vi "DATA.vi"(6 "Torsiometro":refnum<vi>, 7 "simulazione":bool, 8 "error in (no error)":errorcluster, 9 "BANCO":i32=1, 10 "variant":variant, 11 "Queue Name":string) -> (0 "error out":errorcluster, 2 "Stopped":bool)   [LabVIEW 2019]
uses:
  TypeDef/MISURE WT.ctl
  TypeDef/Cluster INFO.ctl
  TypeDef/WT SELECTION.ctl
  TypeDef/Definizione linea.ctl
  TypeDef/Collegamenti_elettrici.ctl
  TypeDef/Control Calcoli.ctl
  TypeDef/Cluster MISURE.ctl
  TypeDef/MISURE NM.ctl
  TypeDef/Cluster misure ALL.ctl
  TypeDef/Cluster NI.ctl
  cDAQ_PLC Folder/controls/StatoAO_cdaq.ctl
  cDAQ_PLC Folder/controls/statoDO_Cdaq.ctl
  TypeDef/ClusterRes.ctl
  TypeDef/INTERFACCIA.ctl
  TypeDef/Lista AO sistema.ctl
  TypeDef/DOinterfaccia.ctl
  cDAQ_PLC Folder/ST1200_LIST_IO/STATO PLC 1.ctl
  cDAQ_PLC Folder/ST1200_LIST_IO/Uscite PLC 1.ctl
  cDAQ_PLC Folder/controls/statoAO_plc_1.ctl
  cDAQ_PLC Folder/ST1200_LIST_IO/StatoDO_PLC_1.ctl
  SINUS PENTA SANTERNO/controls/Parametri inverter letti.ctl
  cDAQ_PLC Folder/ST1200_LIST_IO/STATO PLC 2.ctl
  cDAQ_PLC Folder/ST1200_LIST_IO/Uscite PLC 2.ctl
  cDAQ_PLC Folder/controls/statoAO_plc_2.ctl
  cDAQ_PLC Folder/ST1200_LIST_IO/StatoDO_PLC_2.ctl
  cDAQ_PLC Folder/ST1200_LIST_IO/STATO PLC 3.ctl
  cDAQ_PLC Folder/ST1200_LIST_IO/Uscite PLC 3.ctl
  cDAQ_PLC Folder/controls/statoAO_plc_3.ctl
  cDAQ_PLC Folder/ST1200_LIST_IO/StatoDO_PLC_3.ctl
  DCREG/Parametri DCREG letti.ctl
  TypeDef/sett T e R.ctl
  <vilib>/Analysis/baseanly.llb/Mean (DBL).vi
  Globals.vi
  <vilib>/Utility/file.llb/Read Delimited Spreadsheet (string).vi
  Global prova in corso.vi
  <vilib>/Analysis/NI_AALBase.lvlib
panel:
  out "Cluster READ NI":T1 {"AI (4-20mA)"."AI 15" format="%#_6f"; "AI (4-20mA)"."AI 14" format="%#_6f"; "AI (4-20mA)"."AI 13" format="%#_6f"; "AI (4-20mA)"."AI 11" format="%#_6f"; "AI (4-20mA)"."AI 10" format="%#_6f"; "AI (4-20mA)"."AI 9" format="%#_6f"; "AI (4-20mA)"."AI 4" format="%#_6f"; "AI (4-20mA)"."AI 12" format="%#_6f"; "AI (4-20mA)"."AI 0" format="%#_6f"; "AI (4-20mA)"."AI 1" format="%#_6f"; "AI (4-20mA)"."AI 2" format="%#_6f"; "AI (4-20mA)"."AI 3" format="%#_6f"; "AI (4-20mA)"."AI 5" format="%#_6f"; "AI (4-20mA)"."AI 6" format="%#_6f"; "AI (4-20mA)"."AI 7" format="%#_6f"; "AI (4-20mA)"."AI 8" format="%#_6f"; "AI (0-10V)"."AI 31" format="%#_6f"; "AI (0-10V)"."AI 30" format="%#_6f"; "AI (0-10V)"."AI 29" format="%#_6f"; "AI (0-10V)"."AI 28" format="%#_6f"; "AI (0-10V)"."AI 27" format="%#_6f"; "AI (0-10V)"."AI 26" format="%#_6f"; "AI (0-10V)"."AI 25" format="%#_6f"; "AI (0-10V)"."AI 24" format="%#_6f"; "AI (0-10V)"."AI 23" format="%#_6f"; "AI (0-10V)"."AI 22" format="%#_6f"; "AI (0-10V)"."AI 21" format="%#_6f"; "AI (0-10V)"."AI 20" format="%#_6f"; "AI (0-10V)"."AI 19" format="%#_6f"; "AI (0-10V)"."AI 18" format="%#_6f"; "AI (0-10V)"."AI 17" format="%#_6f"; "AI (0-10V)"."AI 16" format="%#_6f"; "AI (0-10V)"."AI 15" format="%#_6f"; "AI (0-10V)"."AI 14" format="%#_6f"; "AI (0-10V)"."AI 13" format="%#_6f"; "AI (0-10V)"."AI 11" format="%#_6f"; "AI (0-10V)"."AI 10" format="%#_6f"; "AI (0-10V)"."AI 9" format="%#_6f"; "AI (0-10V)"."AI 4" format="%#_6f"; "AI (0-10V)"."AI 12" format="%#_6f"; "AI (0-10V)"."AI 0" format="%#_6f"; "AI (0-10V)"."AI 1" format="%#_6f"; "AI (0-10V)"."AI 2" format="%#_6f"; "AI (0-10V)"."AI 3" format="%#_6f"; "AI (0-10V)"."AI 5" format="%#_6f"; "AI (0-10V)"."AI 6" format="%#_6f"; "AI (0-10V)"."AI 7" format="%#_6f"; "AI (0-10V)"."AI 8" format="%#_6f"}
  out "tamb":dbl
  out "Acq res resistomat":bool=TRUE
  out "simulazione 2":bool
  out "assoc input sensori":string[][](array[string])
  out "Elements in queue":i32
  out "Task READ WT ok":bool
  out "Caratteristiche sensori in":string[][](array[string])
  out "SEND_Main2?":bool
  out "SEND_Main?":bool
  in  "Tab Control":T4(tab)
  out "Cluster Resistenze":T5
  out "MISURE WT":T6
  out "Cluster MISURE":T7={"MISURE NM"={"Banco"="", "Anno"="", "Numero"="", "Ntabella"="", "Misura"="", "Tipo Prova"="", "ProgressivoAcq"="", "Descrizione"="", "Data_ora"="", "t. acq [h:m:s]"="", "t. acq [min]"="", "t. acq [s]"="", "n [rpm]"="", "f [Hz]"="", "U1[V]"="", "U2 [V]"="", "U3 [V]"="", "U123_media [V]"="", "I1[A]"="", "I2[A]"="", "I3[A]"="", "I123_media [A]*I"="", "I_123_sbil [%]"="", "Ulin[V]"="", "Uc [V]"="", "Uaux [V]"="", "Ilin[A]*I"="", "Imar[A]"="", "Iaux[A]"="", "Uarm[V]"="", "Uecc[V]"="", "Iarm[A]*I"="", "Iecc[A]"="", "pf"="", "P1 [W]"="", "P1 [kW]"="", "Q [VAR]"="", "Q [kVAR]"="", "S [VA]"="", "S [kVA]"="", "P1arm[W]"="", "P1ecc[W]"="", "Parm[kW]"="", "P1ecc[kW]"="", "Cond[uF]"="", "P1_linea_6fili[W]"="", "P1_linea_6fili[kW]"="", "eta_gr_6fili [%]"="", "eta_inverter_6fili [%]"="", "pf_linea_6fili"="", "U4 [V]"="", "U5 [V]"="", "U6 [V]"="", "U456_media [V]"="", "I4 [A]"="", "I5 [A]"="", "I6 [A]"="", "I456_media [A]"="", "C [Nm]*C"="", "Cric [Nm]"="", "Cric\\Cnom"="", "Iric[A]"="", "Iric\\Inom"="", "P2_mecc [W]"="", "P2_mecc [kW]"="", "eta motore [%]"="", "Scorr[%]"="", "Tamb[°C]"="", "R1[ohm]"="", "R2[ohm]"="", "R3[ohm]"="", "Rmedia[ohm]"="", "DT_R1[°C]"="", "DT_R2[°C]"="", "DT_R3[°C]"="", "DT_media[°C]"="", "R_marcia[ohm]"="", "R_aux[ohm]"="", "DT_marcia[°C]"="", "DT_aux[°C]"="", "R_Arm[ohm]"="", "R_Ecc[ohm]"="", "DT_Arm[°C]"="", "DT_Ecc[°C]"="", "TambFreddo[°C]"="", "R1_freddo[ohm]"="", "R2_freddo[ohm]"="", "R3_freddo[ohm]"="", "Rmedia_freddo[ohm]"="", "R_Marcia_freddo[ohm]"="", "R_Aux_freddo[ohm]"="", "R_Arm_freddo[ohm]"="", "R_Ecc_freddo[ohm]"="", "TC1 [°C]"="", "TC2 [°C]"="", "TC3 [°C]"="", "TC4 [°C]"="", "TC5 [°C]"="", "TC6 [°C]"="", "TC7 [°C]"="", "TC8 [°C]"="", "PT1000_1[°C]"="", "PT1000_2[°C]"="", "PT1000_3[°C]"="", "Vdc eccitatrice[V]"="", "Idc eccitatrice[A]"="", "Vdc rotore[V]"="", "Idc rotore[A]"="", "Vac rotore[V]"="", "Iac rotore[V]"="", "V dinamo[V]"="", "Portata Q"="", "Pressione H"="", "U1'[V]"="", "U2'[V]"="", "U3'[V]"="", "I1'[A]"="", "I2'[A]"="", "I3'[A]"="", "U''R-N"="", "U''S-N"="", "U'' T-N"="", "U''R-S"="", "U''R-T"="", "U''S-T"="", "I1''[A]"="", "I2''[A]"="", "I3''[A]"="", "F''[Hz]"="", "P''[kW]"="", "CosFi''"="", "PT1000_4[°C]"="", "Scorta 3"=""}, "MISURE ALL"={"Cluster READ NI"={"AI (0-10V)"={"AI 0"=0.0, "AI 1"=0.0, "AI 2"=0.0, "AI 3"=0.0, "AI 4"=0.0, "AI 5"=0.0, "AI 6"=0.0, "AI 7"=0.0, "AI 8"=0.0, "AI 9"=0.0, "AI 10"=0.0, "AI 11"=0.0, "AI 12"=0.0, "AI 13"=0.0, "AI 14"=0.0, "AI 15"=0.0, "AI 16"=0.0, "AI 17"=0.0, "AI 18"=0.0, "AI 19"=0.0, "AI 20"=0.0, "AI 21"=0.0, "AI 22"=0.0, "AI 23"=0.0, "AI 24"=0.0, "AI 25"=0.0, "AI 26"=0.0, "AI 27"=0.0, "AI 28"=0.0, "AI 29"=0.0, "AI 30"=0.0, "AI 31"=0.0}, "StatoAO_Cdaq[0-10V]"={"AO 1"=0.0, "AO 2"=0.0, "AO 3"=0.0, "AO 4"=0.0}, "Contatori [rpm]"={"RPM 1"=0.0, "RPM 2"=0.0}, "StatoAO_Cdaq [4-20mA]"={"Cdaq_AO [0-10V] 0 for Torque"=0.0, "Cdaq_AO [0-10V] 1"=0.0, "Cdaq_AO [0-10V] 2"=0.0, "Cdaq_AO [0-10V] 3"=0.0}, "StatoDO_Cdaq"={"Scorta 0"=FALSE, "Scorta 1"=FALSE, "Scorta 2"=FALSE, "Scorta 3"=FALSE, "Scorta 4"=FALSE, "Scorta 5"=FALSE, "Scorta 6"=FALSE, "Scorta 7"=FALSE, "Scorta 8"=FALSE, "Scorta 9"=FALSE, "Scorta 10"=FALSE, "Scorta 11"=FALSE, "Scorta 12"=FALSE, "Scorta 13"=FALSE, "Scorta 14"=FALSE, "Scorta 15"=FALSE, "Scorta 16"=FALSE, "Scorta 17"=FALSE, "Scorta 18"=FALSE, "Scorta 19"=FALSE, "Scorta 20"=FALSE, "Scorta 21"=FALSE, "Scorta 22"=FALSE, "Scorta 23"=FALSE, "Scorta 24"=FALSE, "Scorta 25"=FALSE, "Scorta 26"=FALSE, "Scorta 27"=FALSE, "Scorta 28"=FALSE, "Scorta 29"=FALSE, "Scorta 30"=FALSE, "Scorta 31"=FALSE}, "DI"={"Scorta 0"=FALSE, "Scorta 1"=FALSE, "Scorta 2"=FALSE, "Scorta 3"=FALSE, "Scorta 4"=FALSE, "Scorta 5"=FALSE, "Scorta 6"=FALSE, "Scorta 7"=FALSE, "Scorta 8"=FALSE, "Scorta 9"=FALSE, "Scorta 10"=FALSE, "Scorta 11"=FALSE, "Scorta 12"=FALSE, "Scorta 13"=FALSE, "Scorta 14"=FALSE, "Scorta 15"=FALSE, "Scorta 16"=FALSE, "Scorta 17"=FALSE, "Scorta 18"=FALSE, "Scorta 19"=FALSE, "Scorta 20"=FALSE, "Scorta 21"=FALSE, "Scorta 22"=FALSE, "Scorta 23"=FALSE, "Scorta 24"=FALSE, "Scorta 25"=FALSE, "Scorta 26"=FALSE, "Scorta 27"=FALSE, "Scorta 28"=FALSE, "Scorta 29"=FALSE, "Scorta 30"=FALSE, "Scorta 31"=FALSE}, "AI (4-20mA)"={"AI 0"=0.0, "AI 1"=0.0, "AI 2"=0.0, "AI 3"=0.0, "AI 4"=0.0, "AI 5"=0.0, "AI 6"=0.0, "AI 7"=0.0, "AI 8"=0.0, "AI 9"=0.0, "AI 10"=0.0, "AI 11"=0.0, "AI 12"=0.0, "AI 13"=0.0, "AI 14"=0.0, "AI 15"=0.0}, "TC [°C]"={"tc 1"=0.0, "tc 2"=0.0, "tc 3"=0.0, "tc 4"=0.0}, "NI Read Values"={"RPM"=0.0, "Frequency"=0.0, "Mod 1"={"Torsiometro 1"=0.0, "Torsiometro 2"=0.0, "Strin Gauge 1"=0.0, "Strin Gauge 2"=0.0}, "Mod 2"={"Termocoppia 1"=0.0, "Termocoppia 2"=0.0, "Termocoppia 3"=0.0, "Termocoppia 4"=0.0}, "Mod 3"={"PT 100 1"=0.0, "PT 100 2"=0.0, "PT 100 3"=0.0, "PT 100 4"=0.0}}}, "MISURE WT"={"URMS 1"=0.0, "IRMS 1"=0.0, "P 1"=0.0, "S 1"=0.0, "Q 1"=0.0, "LAMBDA 1"=0.0, "PHI 1"=0.0, "F U 1"=0.0, "F I 1"=0.0, "NONE 1"=0.0, "URMS 2"=0.0, "IRMS 2"=0.0, "P 2"=0.0, "S 2"=0.0, "Q 2"=0.0, "LAMBDA 2"=0.0, "PHI 2"=0.0, "F U 2"=0.0, "F I 2"=0.0, "NONE 2"=0.0, "URMS 3"=0.0, "IRMS 3"=0.0, "P 3"=0.0, "S 3"=0.0, "Q 3"=0.0, "LAMBDA 3"=0.0, "PHI 3"=0.0, "F U 3"=0.0, "F I 3"=0.0, "NONE 3"=0.0, "URMS SIGMA"=0.0, "IRMS SIGMA"=0.0, "P SIGMA"=0.0, "S SIGMA"=0.0, "Q SIGMA"=0.0, "LAMBDA SIGMA"=0.0, "PHI SIGMA"=0.0, "F U SIGMA"=0.0, "F I SIGMA"=0.0, "NONE 4"=0.0}, "Resistenze Resistomat"={"Res Ch1"=0.0, "Res Ch2"=0.0, "Res Ch3"=0.0, "Tamb"=0.0}, "INTERFACCIA"={"AI"={"Portate"=[], "Pressioni"=[], "Coppie[Nm]"=[], "Valvole prop %"=[], "RPM"=[], "Livelli"=[], "Temperature"=[], "Riferimenti %"=[], "TENSIONI"=[], "CORRENTI"=[]}, "DI (logici)"={"Start da pulsantiera"=FALSE, "Stop da pulsantiera"=FALSE, "Reset da pulsantiera"=FALSE, "Sistema OK"=FALSE, "Collaudo abilitato"=FALSE, "Potenza trifase abilitata"=FALSE, "Potenza monofase abilitata"=FALSE, "Potenza DC abilitata"=FALSE, "Potenza DC ECC abilitata"=FALSE, "Start alimentazione AC"=FALSE, "Start alimentazione DC"=FALSE, "Start DC eccitazione"=FALSE, "Teleruttore WT abilitato"=FALSE, "Teleruttore Resistomat abilitato"=FALSE, "Teleruttore corto fasi"=FALSE, "Ramo 1 resistomat"=FALSE, "Ramo 2 resistomat"=FALSE, "Ramo 3 resistomat"=FALSE, "B1 Scelta linea elettrica 1"=FALSE, "B1 Scelta linea elettrica 2"=FALSE, "B1 Scelta linea elettrica 3"=FALSE, "B1 Scelta linea elettrica 4"=FALSE, "B1 Scelta linea elettrica 5"=FALSE, "B2 Scelta linea elettrica 1"=FALSE, "B2 Scelta linea elettrica 2"=FALSE, "B2 Scelta linea elettrica 3"=FALSE, "B2 Scelta linea elettrica 4"=FALSE, "B2 Scelta linea elettrica 5"=FALSE, "Rotore bloccato 1"=FALSE, "Rotore bloccato 2"=FALSE, "FRENO 1 abilitato"=FALSE, "FRENO 1 run"=FALSE, "FRENO 1 senso rotaz"=FALSE, "FRENO 1 ctrl velocità"=FALSE, "FRENO 2 abilitato"=FALSE, "FRENO 2 run"=FALSE, "FRENO 2 senso rotaz"=FALSE, "FRENO 2 ctrl velocità"=FALSE, "ALIM 1 abilitato"=FALSE, "ALIM 1 run"=FALSE, "ALIM 2 abilitato"=FALSE, "ALIM 2 run"=FALSE, "ALIM 3 abilitato"=FALSE, "ALIM 3 run"=FALSE, "FRENO 1 ctrl coppia"=FALSE, "FRENO 2 ctrl coppia"=FALSE, "FRENO 3 ctrl coppia"=FALSE, "DI (logici) aggiuntivi impianto"={"Solo freno abilitato"=FALSE, "Carico resistivo abilitato"=FALSE, "AFE+freno abilitato"=FALSE, "Protezioni chiuse"=FALSE, "Start potenza AFE"=FALSE, "AFE in marcia"=FALSE}, "Misura corrente diretta WT"=FALSE, "Misura corrente sens ext"=FALSE, "Sens ext abilitati"=FALSE}, "AO non scalati"={"FRENO1 rif vel"=0.0, "FRENO1 rif Coppia"=0.0, "FRENO2 rif vel"=0.0, "FRENO2 rif Coppia"=0.0, "ALIM1 rif V"=0.0, "ALIM1 rif F"=0.0, "ALIM2 rif V"=0.0, "ALIM2 rif F"=0.0, "ALIM3 rif V"=0.0, "ALIM3 rif F"=0.0, "Fnom keb"=0.0, "Rpm nom keb"=0.0, "Pnom keb"=0.0, "Inom keb"=0.0, "Vnom keb"=0.0, "Rpm max keb"=0.0, "Tempo rampa keb"=0.0, "Tipo Mot keb"=0.0, "FRENO  rif Coppia "=0.0, "FRENO  rif  Corrente"=0.0}, "AO scalati"={"FRENO1 rif vel"=0.0, "FRENO1 rif Coppia"=0.0, "FRENO2 rif vel"=0.0, "FRENO2 rif Coppia"=0.0, "ALIM1 rif V"=0.0, "ALIM1 rif F"=0.0, "ALIM2 rif V"=0.0, "ALIM2 rif F"=0.0, "ALIM3 rif V"=0.0, "ALIM3 rif F"=0.0, "Fnom keb"=0.0, "Rpm nom keb"=0.0, "Pnom keb"=0.0, "Inom keb"=0.0, "Vnom keb"=0.0, "Rpm max keb"=0.0, "Tempo rampa keb"=0.0, "Tipo Mot keb"=0.0, "FRENO  rif Coppia "=0.0, "FRENO  rif  Corrente"=0.0}, "DO (logici)"={"Scelta banco 1"=FALSE, "Scelta banco 2"=FALSE, "Scelta banco 3"=FALSE, "FRENO 1 abilita"=FALSE, "FRENO 1 start"=FALSE, "FRENO 1 senso rotaz"=FALSE, "FRENO 1 ctrl velocità"=FALSE, "FRENO 2 abilita"=FALSE, "FRENO 2 start"=FALSE, "FRENO 2 senso rotaz"=FALSE, "FRENO 2 ctrl velocità"=FALSE, "ALIM 1 abilita"=FALSE, "ALIM 1 start"=FALSE, "ALIM 2 abilita"=FALSE, "ALIM 2 start"=FALSE, "ALIM 3 abilita"=FALSE, "ALIM 3 start"=FALSE, "Abilita linea trifase"=FALSE, "Abilita linea monofase"=FALSE, "Abilita linea dc"=FALSE, "Abilita linea dc eccit"=FALSE, "B1 Linea elettrica 1"=FALSE, "B1 Linea elettrica 2"=FALSE, "B1 Linea elettrica 3"=FALSE, "B1 Linea elettrica 4"=FALSE, "B1 Linea elettrica 5"=FALSE, "B2 Linea elettrica 1"=FALSE, "B2 Linea elettrica 2"=FALSE, "B2 Linea elettrica 3"=FALSE, "B2 Linea elettrica 4"=FALSE, "B2 Linea elettrica 5"=FALSE, "Start potenza AC"=FALSE, "Stop pontenza AC"=FALSE, "Start potenza DC"=FALSE, "Stop potenza DC"=FALSE, "Start potenza eccitaz"=FALSE, "Stop potenza eccitaz"=FALSE, "Reset allarmi"=FALSE, "watchdog"=FALSE, "Scala torsiometro B1"=FALSE, "Controllo torsiom B1"=FALSE, "Scala torsiometro B2"=FALSE, "Controllo torsiom B2"=FALSE, "Teleruttore WT abilita"=FALSE, "Teleruttore Resistomat abilita"=FALSE, "Teleruttore corto fasi"=FALSE, "Ramo 1 resistomat"=FALSE, "Ramo 2 resistomat"=FALSE, "Ramo 3 resistomat"=FALSE, "Collaudo in corso"=FALSE, "Allarme presente"=FALSE, "Enable Res Meter"=FALSE, "Bypass Res Meter"=FALSE, "2nd canale Res Meter"=FALSE, "Scala 200/2000 res meter"=FALSE, "Taratura res meter"=FALSE, "FRENO 1 ctrl coppia"=FALSE, "FRENO 2 ctrl coppia"=FALSE, "FRENO 3 ctrl coppia"=FALSE, "Aggiuntivi impianto"={"Senso rotazione alim 1"=FALSE, "Senso rotazione alim 2"=FALSE}, "ALIM 1 stop"=FALSE, "ALIM 2 stop"=FALSE, "ALIM 3 stop"=FALSE, "FRENO 1 stop"=FALSE, "FRENO 2 stop"=FALSE, "FRENO 3 stop"=FALSE, "B1 configurazione freno B"=FALSE, "B2 configurazione freno B"=FALSE, "Abilita scrittura KEB"=FALSE, "Bench Selection (0-B1,1-B2)"=FALSE, "Select current mode"=FALSE, "Select torque mode"=FALSE, "Select speed mode"=FALSE, "Start"=FALSE, "Stop"=FALSE, "Block"=FALSE, "Enable Force mode"=FALSE, "Abilita linea 125 A"=FALSE, "Abilita linea 63 A"=FALSE, "Abilita linea 16 A"=FALSE, "Aum Tensione Variac"=FALSE, "Dim Tesnione Variac"=FALSE, "Abilita ellectro stractura"=FALSE, "Risprinito Emergence"=FALSE, "Abilita collaudo"=FALSE, "Disabilita collaudo"=FALSE, "External Alaram"=FALSE, "Enable external program"=FALSE, "Reset"=FALSE, "Abilita Ingresso Variac"=FALSE, "Abilita Ventilatore Variac"=FALSE, "Abilita Uscita Variac "=FALSE}}, "FREDDO resistomat"={"Res Ch1"=0.0, "Res Ch2"=0.0, "tAMB"=0.0, "Res Ch3"=0.0}, "STATO PLC 1"={"USCITE PLC"={"AO (real) 2"={"SCORTA 1"=0.0, "SCORTA 2"=0.0, "SCORTA 3"=0.0, "SCORTA 4"=0.0, "SCORTA 5"=0.0, "SCORTA 6"=0.0, "SCORTA 7"=0.0, "SCORTA 8"=0.0}, "statoAO_PLC out"={"Rif Lim coppia freno [%]"=nan, "Rif rpm freno [%]"=nan, "Rif coppia freno [%]"=0.0, "Rif V alimentatore [%]"=0.0, "Rif F alimentatore [%]"=0.0}, "DO (bit)"={"Scelta banco 1"=FALSE, "Set dati motore freno 2"=FALSE, "Diretto inverter"=FALSE, "Filtro LC"=FALSE, "Marcia ALIM (1s)"=FALSE, "Marcia FRENO (1s)"=FALSE, "Stop AFE (1s)"=FALSE, "Stop freno (1s)"=FALSE, "Reset allarmi"=FALSE, "Watchdog"=FALSE, "Senso rotazione"=FALSE, "Abilita collaudo (1s)"=FALSE, "Disabilita collaudo (1s)"=FALSE, "Abilitazione ALIM"=FALSE, "Abilitazione FRENO"=FALSE, "Teleruttore WT"=FALSE, "Senso rot motore prova"=FALSE, "Scorta 7"=FALSE, "Scorta 8"=FALSE, "Scorta 9"=FALSE, "Scorta 10"=FALSE, "Scorta 11"=FALSE, "Scorta 12"=FALSE, "Scorta 13"=FALSE}}, "Stato DI_PLC"={"Sistema OK"=FALSE, "Rotore bloccato"=FALSE, "Scorta 1"=FALSE, "Prova diretto inverter"=FALSE, "Prova con filtro LC"=FALSE, "Teleruttore WT abilitato"=FALSE, "Alim sinus penta abilitato"=FALSE, "Alim sinus penta in marcia"=FALSE, "Freno abilitato"=FALSE, "Freno in marcia"=FALSE, "Senso rotazione freno"=FALSE, "Potenza abilitata"=FALSE, "Scorta 3"=FALSE, "Scorta 4"=FALSE, "scorta 5"=FALSE, "scorta 6"=FALSE}, "AI plc"={"Allarmi 1"=0.0, "Allarmi 2"=0.0, "Scorta 1"=0.0, "Scorta 2"=0.0, "RPM mot prova"=0.0, "I mot prova"=0.0, "RPM freno"=0.0, "I freno"=0.0, "Scorta 3"=0.0, "Scorta 4"=0.0}}, "Res Ch2"=0.0, "Res Ch2 2"=0.0, "FREDDO res meter"={"Res Ch1"=0.0, "Res Ch2"=0.0, "tAMB"=0.0, "Res Ch3"=0.0}, "Resistenze Res Meter"={"Res Ch1"=0.0, "Res Ch2"=0.0, "Res Ch3"=0.0, "Tamb"=0.0}, "READ SINUS PENTA"={"Menù Misure motore (M000-M030)"={"Rif vel a regime (int)"=0, "Rif vel a regime (dec)"=0, "Rif vel dopo rampe (int)"=0, "Rif vel dopo rampe (dec)"=0, "RPM motore (int)"=0, "RPM motore (dec)"=0, "FREQout inverter"=0, "Rif coppia a regime(Nm)"=0, "Richiesta di coppia (Nm)"=0, "Coppia generata dal motore(Nm)"=0, "Rif coppia a regime(%)"=0, "Richiesta di coppia (%)"=0, "Coppia generata dal motore(%)"=0, "Coppia max richiesta prima delle rampe(Nm)"=0, "Coppia max richiesta dopo le rampe(Nm)"=0, "Limite di velocità prima delle rampe"=0, "Limite di velocità dopo le rampe"=0, "Coppia max richiesta prima delle rampe(%)"=0, "Coppia max richiesta dopo le rampe(%)"=0, "Rif di flusso"=0, "Corrente di uscita"=0, "Capacità termica del motore"=0, "Tensione di uscita"=0, "Potenza di uscita"=0, "Energia consumata (LSword)"=0, "Energia consumata (MSword)"=0, "Tensione bus DC"=0, "Tensione di rete"=0}, "Menù regolatore PID (M018-M024)"={"Rif PID a regime(%)"=0, "Rif pid dopo rampe(%)"=0, "Retroazione del pid(%)"=0, "Errore del pid(%)"=0, "uscita del pid(%)"=0, "Rif del pid dopo le rampe"=0, "Retroazione del pid"=0}, "Menù ingressi digitali (M031-M036)"={"Ingressi digitali ritardati"=0, "Ingressi digitali istantanei"=0, "Moresettiera comando loc"=0, "Morsett comando da seriale"=0, "Morsett comando bus di campo"=0, "Ing dig ausiliari da morsettiera"=0, "Ing dig ausiliari da seriale"=0}, "Menù riferimenti (M037-M051)"={"Rif analog est REF"=0, "Rif analog est AIN1"=0, "Rif analog est AIN2"=0, "Rif analog est XAIN4"=0, "Rif analog est XAIN5"=0, "Rif velocità da seriale(int)"=0, "Rif velocità bus di campo(int)"=0, "Rif coppia da seriale"=0, "Rif coppia bus di campo"=0, "Rif del PID da seriale"=0, "Rif del PID da bus di campo"=0, "Retroazione del PID da seriale"=0, "Retroazione del PIDda bus di campo"=0, "Rif da encoder"=0, "Rif in frequenza"=0, "Rif velocità da seriale(dec)"=0, "Rif velocità bus di campo(dec)"=0}, "Menù rampe (P009-P033)"={"Tempo di dec rampa di vel 1"=0, "Tempo di acc rampa di vel 2"=0, "Tempo di dec rampa di vel 2"=0, "Tempo di acc rampa di vel 1"=0, "Unità di mis tempi rampe vel 1/2"=0, "Tempo di acc rampa di vel 3"=0, "Tempo di dec rampa di vel 3"=0, "Tempo di acc rampa di vel 4"=0, "Tempo di dec rampa di vel 4"=0, "Unità di mis tempi rampe vel 3/4"=0, "Selettore arrottondam rampe"=0, "Tempo di arrotond iniz rampa acc"=0, "Tempo di arrotond finale rampa acc"=0, "Tempo di arrotond iniz rampa dec"=0, "Tempo di rampa di salita rif coppia"=0, "Tempo di rampa di discesa rif coppia"=0, "Unità di misura rampa coppia"=0, "Tempo rampa acc marcia jog"=0, "Tempo rampa dec marcia jog"=0, "Reset acc ai cambi pendenza"=0, "rampa di acc in fire mode"=0, "rampa di dec in fire mode"=0, "Tempo di arrotond finale rampa dec"=0}, "Menù controllo motore(C008-C128)"={"Numero motori configurati"=0, "Tipo algoritmo di controllo Mot1"=0, "Tipo rif Mot1"=0, "Tensione nominale rete"=0, "Retroaz di vel da encoder Mot1"=0, "Tipo curva V/f Mot1"=0, "Rotazione delle fasi Mot1"=0, "Freq nominale del motore Mot1"=0, "RPM nominali del motore Mot1"=0, "Potenza nominale del motore Mot1"=0, "Corrente nominale del motore Mot1"=0, "Tensione nominale del motore mot1"=0, "Potenza a vuoto del motore Mot1"=0, "Corrente a vuoto del motore Mot1"=0, "Resistenza statorica del motore Mot1"=0, "Induttanza di dispersione Mot1"=0, "Induttanza mutua motore"=0, "Costante di tempo rotorica"=0, "Costante di tempo filtro pb"=0, "Velocità minima motore"=0, "Velocità massima motore"=0}, "Menù configurazione PID"={"Selezione riferimento n.1"=0, "Selezione retroazione n.1"=0, "Modalità di fuzionamento PID"=0, "Termine derivativo calcolato su err o mis"=0, "Proporz moltiplica deriv e integrale"=0, "Azione del PID"=0}, "ID"=0.0, "Menù uscite digitali"={"MDO4 Inverter pronto"=0}, "Fcarrier"={"Fcarrier Min (Hz)"=0, "Fcarrier Max (Hz)"=0}, "stato inverter M089"=0.0, "Riferimenti"={"Rif tensione"=0, "Rif velocità"=0}, "Comunicazione"=FALSE, "Modalità stop"=0.0}, "STATO PLC 2"={"USCITE PLC"={"AO (real) 2"={"SCORTA 1"=0.0, "SCORTA 2"=0.0, "SCORTA 3"=0.0, "SCORTA 4"=0.0, "SCORTA 5"=0.0, "SCORTA 6"=0.0, "SCORTA 7"=0.0, "SCORTA 8"=0.0}, "statoAO_PLC out"={"Condensatori"=0.0, "Scorta 1"=0.0, "Scorta 2"=0.0}, "DO (bit)"={"Relè misura resistomat"=FALSE, "Misura res ramo 1"=FALSE, "Misura res ramo 2"=FALSE, "Misura res ramo 3"=FALSE, "Scelta banco 2"=FALSE, "Scala Torsiometro"=FALSE, "Ctrl torsiometro"=FALSE, "Select current mode"=FALSE, "Select Torque mode"=FALSE, "Select speed mode"=FALSE, "Watchdog"=FALSE, "Scorta"=FALSE, "Scorta 2"=FALSE, "Scorta 3"=FALSE, "Scorta 4"=FALSE, "Scorta 5"=FALSE, "Bench selection"=FALSE, "External alarm"=FALSE, "Enable external program"=FALSE, "Reset allarmi"=FALSE, "Start"=FALSE, "Stop"=FALSE, "Block"=FALSE, "Scorta 6"=FALSE}}, "Stato DI_PLC"={"Sistema ok"=FALSE, "Relè Resistomat abilitato"=FALSE, "Freno abilitato"=FALSE, "Freno in marcia"=FALSE, "scorta b"=FALSE, "scorta a"=FALSE, "scorta 1"=FALSE, "scorta 2"=FALSE, "scorta 3"=FALSE, "scorta 4"=FALSE, "Scorta 5"=FALSE, "Scorta 6"=FALSE, "Scorta 7"=FALSE, "Scorta 8"=FALSE, "Scorta 9"=FALSE, "Scorta 10"=FALSE}, "AI plc"={"Allarmi 1"=0.0, "Allarmi 2"=0.0, "TC 1"=0.0, "TC 2"=0.0, "TC 3"=0.0, "TC 4"=0.0, "TC 5"=0.0, "TC 6"=0.0, "TC 7"=0.0, "TC 8"=0.0, "PT1000 1"=0.0, "PT1000 2"=0.0, "PT1000 3"=0.0, "PT1000 4"=0.0}}, "STATO PLC 3"={"USCITE PLC"={"AO (real) 2"={"SCORTA 1"=0.0, "SCORTA 2"=0.0, "SCORTA 3"=0.0, "SCORTA 4"=0.0, "SCORTA 5"=0.0, "SCORTA 6"=0.0, "SCORTA 7"=0.0, "SCORTA 8"=0.0}, "statoAO_PLC out"={"Rif velocità alimentatore"=0.0, "Scorta"=0.0, "Tipo Motore  keb"=0.0, "I nom keb"=0.0, "RPM nom keb"=0.0, "V nom keb"=0.0, "F nom keb"=0.0, "t rampa keb"=0.0}, "DO (bit)"={"Select linea Inverter"=FALSE, "Abilita sense wattmetro"=FALSE, "Bypass filtro LC"=FALSE, "Filtro LC"=FALSE, "Bypass trasformatore"=FALSE, "Trasformatore"=FALSE, "Abilita uscite variac"=FALSE, "Abilita linea 125 A"=FALSE, "Abilita linea 63 A"=FALSE, "Abilita linea 16 A"=FALSE, "Abilita Scrittura Dati Keb"=FALSE, "Abilita alimentatore"=FALSE, "Marcia alimentatore (1s)"=FALSE, "Stop alimentatore (1s)"=FALSE, "Senso rot mot prova"=FALSE, "Watchdog"=FALSE, "Aumenta tensione variac"=FALSE, "Diminuisci tensione variac "=FALSE, "Blocco elettroserrature"=FALSE, "Ripristino emergence"=FALSE, "Abilita ingresso variac"=FALSE, "Abilita ventilatore variac"=FALSE, "Reset Allarm"=FALSE, "Scorta 1"=FALSE, "Scorta 2"=FALSE, "Scorta 3"=FALSE, "Scorta 4"=FALSE, "Scorta 5"=FALSE, "Scorta 6"=FALSE, "Scorta 7"=FALSE, "Scorta 8"=FALSE, "Scorta 9"=FALSE, "Abilita collaudo"=FALSE, "Disabilita collaudo "=FALSE, "Scorta 10"=FALSE, "Scorta 11"=FALSE, "Scorta 12"=FALSE, "Scorta 13"=FALSE, "Scorta 14"=FALSE, "Scorta 15"=FALSE}}, "Stato DI_PLC"={"Sistema OK"=FALSE, "Rotore bloccato"=FALSE, "Filtro LC"=FALSE, "Bypass Filtro LC"=FALSE, "Scelta Trasformatore"=FALSE, "Scelta Bypass trasformatore"=FALSE, "Teleruttore wt abilitato"=FALSE, "Alimentatore abilitato"=FALSE, "Alimentatore in marcia"=FALSE, "Scorta 1"=FALSE, "Scorta 2"=FALSE, "Scorta 3"=FALSE, "Potenza abilitata"=FALSE, "Alimentatore in allarme"=FALSE, "Scorta 4"=FALSE, "Conferma dati KEB"=FALSE, "Scorta 5"=FALSE, "Warning Inverter Alimentatore"=FALSE, "Variac Abilitato"=FALSE, "Linea 125 A abilitata"=FALSE, "Linea 63 A abilitata"=FALSE, "Linea 16 A abilitata"=FALSE, "Scorta 6"=FALSE, "Enable force mode"=FALSE}, "AI plc"={"Allarmi 1"=0.0, "Allarmi 2"=0.0, "RPM motore prova"=0.0, "Corrente motore prova"=0.0, "RPM freno"=0.0, "Corrente freno"=0.0, "Tipo motore keb"=0.0, "I nom keb"=0.0, "RPM nom keb"=0.0, "V nom keb"=0.0, "F nom keb"=0.0, "T rampa keb"=0.0, "scorta"=0.0, "Scorta 2"=0.0}}, "DCREG"={"Parametri di misura"={"M000"=0.0, "M001"=0.0, "M002"=0.0, "M003"=0.0, "M004"=0.0, "M005"=0.0, "M006"=0.0, "M007"=0.0, "M008"=0.0, "M009"=0.0, "M010"=0.0, "M011"=0.0, "M012"=0.0, "M013"=0.0, "M014"=0.0, "M015"=0.0, "M016"=0.0, "M017"=0.0, "M018"=0.0, "M019"=0.0, "M020"=0.0, "M021"=0.0, "M022"=0.0, "M023"=0.0, "M024"=0.0, "M025"=0.0, "M026"=0.0, "M027"=0.0, "M028"=0.0, "M029"=0.0, "M030"=0.0, "M031"=0.0}, "Parametri di programmazione"={"P000"=0.0, "P001"=0.0, "P002"=0.0, "P003"=0.0, "P004"=0.0, "P005"=0.0, "P006"=0.0, "P010"=0.0, "P011"=0.0, "P012"=0.0, "P013"=0.0, "P014"=0.0, "P015"=0.0, "P016"=0.0, "P030"=0.0, "P031"=0.0, "P032"=0.0, "P033"=0.0, "P034"=0.0, "P035"=0.0, "P036"=0.0, "P037"=0.0, "P038"=0.0, "P039"=0.0, "P040"=0.0, "P050"=0.0, "P051"=0.0, "P052"=0.0, "P053"=0.0, "P054"=0.0, "P055"=0.0, "P056"=0.0, "P057"=0.0, "P058"=0.0, "P059"=0.0, "P060"=0.0, "P061"=0.0, "P062"=0.0, "P070"=0.0, "P071"=0.0, "P073"=0.0, "P074"=0.0, "P076"=0.0, "P077"=0.0, "P079"=0.0, "P080"=0.0, "P082"=0.0, "P083"=0.0, "P084"=0.0, "P085"=0.0, "P086"=0.0, "P087"=0.0, "P088"=0.0, "P100"=0.0, "P101"=0.0, "P102"=0.0, "P103"=0.0, "P104"=0.0, "P110"=0.0, "P111"=0.0, "P120"=0.0, "P121"=0.0, "P122"=0.0, "P123"=0.0, "P124"=0.0, "P125"=0.0, "P126"=0.0, "P127"=0.0, "P128"=0.0, "P129"=0.0, "P130"=0.0, "P131"=0.0, "P132"=0.0, "P133"=0.0, "P134"=0.0, "P150"=0.0, "P151"=0.0, "P152"=0.0, "P153"=0.0, "P154"=0.0, "P155"=0.0, "P156"=0.0, "P157"=0.0, "P158"=0.0, "P170"=0.0, "P171"=0.0, "P172"=0.0, "P173"=0.0, "P174"=0.0, "P175"=0.0, "P176"=0.0, "P177"=0.0, "P178"=0.0, "P179"=0.0, "P180"=0.0, "P181"=0.0, "P182"=0.0, "P183"=0.0, "P184"=0.0, "P185"=0.0, "P186"=0.0, "P187"=0.0, "P188"=0.0, "P189"=0.0, "P190"=0.0, "P191"=0.0, "P192"=0.0, "P193"=0.0, "P194"=0.0, "P195"=0.0, "P196"=0.0, "P197"=0.0, "P198"=0.0, "P199"=0.0, "P211"=0.0, "P212"=0.0, "P213"=0.0, "P214"=0.0, "P215"=0.0, "P216"=0.0, "P217"=0.0, "P221"=0.0, "P222"=0.0, "P223"=0.0, "P224"=0.0, "P230"=0.0, "P231"=0.0, "P240"=0.0, "P250"=0.0, "P251"=0.0}, "Parametri di configurazione"={"C000"=0.0, "C001"=0.0, "C002"=0.0, "C010"=0.0, "C011"=0.0, "C012"=0.0, "C014"=0.0, "C015"=0.0, "C016"=0.0, "C017"=0.0, "C018"=0.0, "C030"=0.0, "C050"=0.0, "C051"=0.0, "C052"=0.0, "C060"=0.0, "C061"=0.0, "C062"=0.0, "C063"=0.0, "C070"=0.0, "C072"=0.0, "C074"=0.0, "C090"=0.0, "C091"=0.0, "C092"=0.0, "C093"=0.0, "C094"=0.0, "C100"=0.0, "C101"=0.0, "C102"=0.0, "C103"=0.0, "C105"=0.0, "C106"=0.0, "C107"=0.0, "C108"=0.0, "C110"=0.0, "C111"=0.0, "C112"=0.0, "C120"=0.0, "C121"=0.0, "C122"=0.0, "C130"=0.0, "C131"=0.0, "C132"=0.0, "C133"=0.0, "C134"=0.0, "C135"=0.0, "C141"=0.0, "C142"=0.0, "C143"=0.0, "C150"=0.0, "C151"=0.0, "C153"=0.0, "C154"=0.0, "C155"=0.0, "C156"=0.0, "C157"=0.0, "C158"=0.0, "C159"=0.0, "C160"=0.0, "C161"=0.0, "C162"=0.0, "C163"=0.0, "C164"=0.0, "C165"=0.0, "C170"=0.0}, "Codice allarme"=0.0, "Comunicazione"=FALSE}}} {"MISURE ALL"."Cluster READ NI"."AI (4-20mA)"."AI 15" format="%#_6f"; "MISURE ALL"."Cluster READ NI"."AI (4-20mA)"."AI 14" format="%#_6f"; "MISURE ALL"."Cluster READ NI"."AI (4-20mA)"."AI 13" format="%#_6f"; "MISURE ALL"."Cluster READ NI"."AI (4-20mA)"."AI 11" format="%#_6f"; "MISURE ALL"."Cluster READ NI"."AI (4-20mA)"."AI 10" format="%#_6f"; "MISURE ALL"."Cluster READ NI"."AI (4-20mA)"."AI 9" format="%#_6f"; "MISURE ALL"."Cluster READ NI"."AI (4-20mA)"."AI 4" format="%#_6f"; "MISURE ALL"."Cluster READ NI"."AI (4-20mA)"."AI 12" format="%#_6f"; "MISURE ALL"."Cluster READ NI"."AI (4-20mA)"."AI 0" format="%#_6f"; "MISURE ALL"."Cluster READ NI"."AI (4-20mA)"."AI 1" format="%#_6f"; "MISURE ALL"."Cluster READ NI"."AI (4-20mA)"."AI 2" format="%#_6f"; "MISURE ALL"."Cluster READ NI"."AI (4-20mA)"."AI 3" format="%#_6f"; "MISURE ALL"."Cluster READ NI"."AI (4-20mA)"."AI 5" format="%#_6f"; "MISURE ALL"."Cluster READ NI"."AI (4-20mA)"."AI 6" format="%#_6f"; "MISURE ALL"."Cluster READ NI"."AI (4-20mA)"."AI 7" format="%#_6f"; "MISURE ALL"."Cluster READ NI"."AI (4-20mA)"."AI 8" format="%#_6f"; "MISURE ALL"."Cluster READ NI"."AI (0-10V)"."AI 31" format="%#_6f"; "MISURE ALL"."Cluster READ NI"."AI (0-10V)"."AI 30" format="%#_6f"; "MISURE ALL"."Cluster READ NI"."AI (0-10V)"."AI 29" format="%#_6f"; "MISURE ALL"."Cluster READ NI"."AI (0-10V)"."AI 28" format="%#_6f"; "MISURE ALL"."Cluster READ NI"."AI (0-10V)"."AI 27" format="%#_6f"; "MISURE ALL"."Cluster READ NI"."AI (0-10V)"."AI 26" format="%#_6f"; "MISURE ALL"."Cluster READ NI"."AI (0-10V)"."AI 25" format="%#_6f"; "MISURE ALL"."Cluster READ NI"."AI (0-10V)"."AI 24" format="%#_6f"; "MISURE ALL"."Cluster READ NI"."AI (0-10V)"."AI 23" format="%#_6f"; "MISURE ALL"."Cluster READ NI"."AI (0-10V)"."AI 22" format="%#_6f"; "MISURE ALL"."Cluster READ NI"."AI (0-10V)"."AI 21" format="%#_6f"; "MISURE ALL"."Cluster READ NI"."AI (0-10V)"."AI 20" format="%#_6f"; "MISURE ALL"."Cluster READ NI"."AI (0-10V)"."AI 19" format="%#_6f"; "MISURE ALL"."Cluster READ NI"."AI (0-10V)"."AI 18" format="%#_6f"; "MISURE ALL"."Cluster READ NI"."AI (0-10V)"."AI 17" format="%#_6f"; "MISURE ALL"."Cluster READ NI"."AI (0-10V)"."AI 16" format="%#_6f"; "MISURE ALL"."Cluster READ NI"."AI (0-10V)"."AI 15" format="%#_6f"; "MISURE ALL"."Cluster READ NI"."AI (0-10V)"."AI 14" format="%#_6f"; "MISURE ALL"."Cluster READ NI"."AI (0-10V)"."AI 13" format="%#_6f"; "MISURE ALL"."Cluster READ NI"."AI (0-10V)"."AI 11" format="%#_6f"; "MISURE ALL"."Cluster READ NI"."AI (0-10V)"."AI 10" format="%#_6f"; "MISURE ALL"."Cluster READ NI"."AI (0-10V)"."AI 9" format="%#_6f"; "MISURE ALL"."Cluster READ NI"."AI (0-10V)"."AI 4" format="%#_6f"; "MISURE ALL"."Cluster READ NI"."AI (0-10V)"."AI 12" format="%#_6f"; "MISURE ALL"."Cluster READ NI"."AI (0-10V)"."AI 0" format="%#_6f"; "MISURE ALL"."Cluster READ NI"."AI (0-10V)"."AI 1" format="%#_6f"; "MISURE ALL"."Cluster READ NI"."AI (0-10V)"."AI 2" format="%#_6f"; "MISURE ALL"."Cluster READ NI"."AI (0-10V)"."AI 3" format="%#_6f"; "MISURE ALL"."Cluster READ NI"."AI (0-10V)"."AI 5" format="%#_6f"; "MISURE ALL"."Cluster READ NI"."AI (0-10V)"."AI 6" format="%#_6f"; "MISURE ALL"."Cluster READ NI"."AI (0-10V)"."AI 7" format="%#_6f"; "MISURE ALL"."Cluster READ NI"."AI (0-10V)"."AI 8" format="%#_6f"}
  out "DATI UL":T29
  out "DATI NM":T30
  out "Cluster INFO":T31={"Scelta wattmetro"={"Wattmetro"=enum."No Selection"}, "SET RPM"=0.0, "SET TEMP"=0.0, "Array banchi"=[{"Nome"="Elettropompa", "Tors. scala1"=0, "Tors. scala2"=0, "rpm"=0, "TAMB"=0, "Indici Temperature"=[0, 1], "Indice freno"=1, "alimentatore trifase"=0, "alimentatore monofase"=0, "alimentatore dc arm"=0, "alimentatore dc ecc"=0, "alimentatore dc mp"=0}, {"Nome"="Sommersa", "Tors. scala1"=0, "Tors. scala2"=0, "rpm"=0, "TAMB"=1, "Indici Temperature"=[0, 1], "Indice freno"=0, "alimentatore trifase"=0, "alimentatore monofase"=0, "alimentatore dc arm"=0, "alimentatore dc ecc"=0, "alimentatore dc mp"=0}], "Array valvole linee avvio/fermata"=[], "banco selezionato"=0, "Nomi valvole prop sistema"=[], "canale-- sensore"=[], "Attriti B1"=[], "Attriti B2"=[], "Collegamento elettrico"={"ALIMENTAZIONE ELETTRICA"=enum."AC TRIFASE", "ID"=0, "#rami freddo\\eq term resmeter"=0, "#rami riscaldamento resmeter"=0, "#rami freddo\\eq term resistomat"=0, "#rami riscaldamento resistomat"=0, "CALCOLI"=enum."AC TRIFASE"}, "lingua"=0, "Costanti collaudo"={"P [bar]"=0.0, "T amb. [°C]"=0.0, "Umidità [%]"=0.0, "T acqua [°C] 2"=0.0}, "OPZIONI MISURE RES"={"MISURA A FREDDO"=enum."RESISTOMAT", "MISURA EQ. TERMICO"=enum."RESISTOMAT", "MISURA DT PROVA IN CORSO"=enum."RESISTOMAT - CON FERMATE", "MISURE PRIMA E DOPO"=enum."RESISTOMAT", "STRUMENTI PRESENTI"=enum."NESSUNO"}, "Dati targa motore"={"Vnom"=0.0, "Fnom"=0.0, "Inom"=0.0, "Cnom"=0.0, "Npoli"=0.0, "Scorta 1"=0.0, "Scorta 2"=0.0, "Scorta 3"=0.0}}
  out "LOOP TIME (ms)":u32
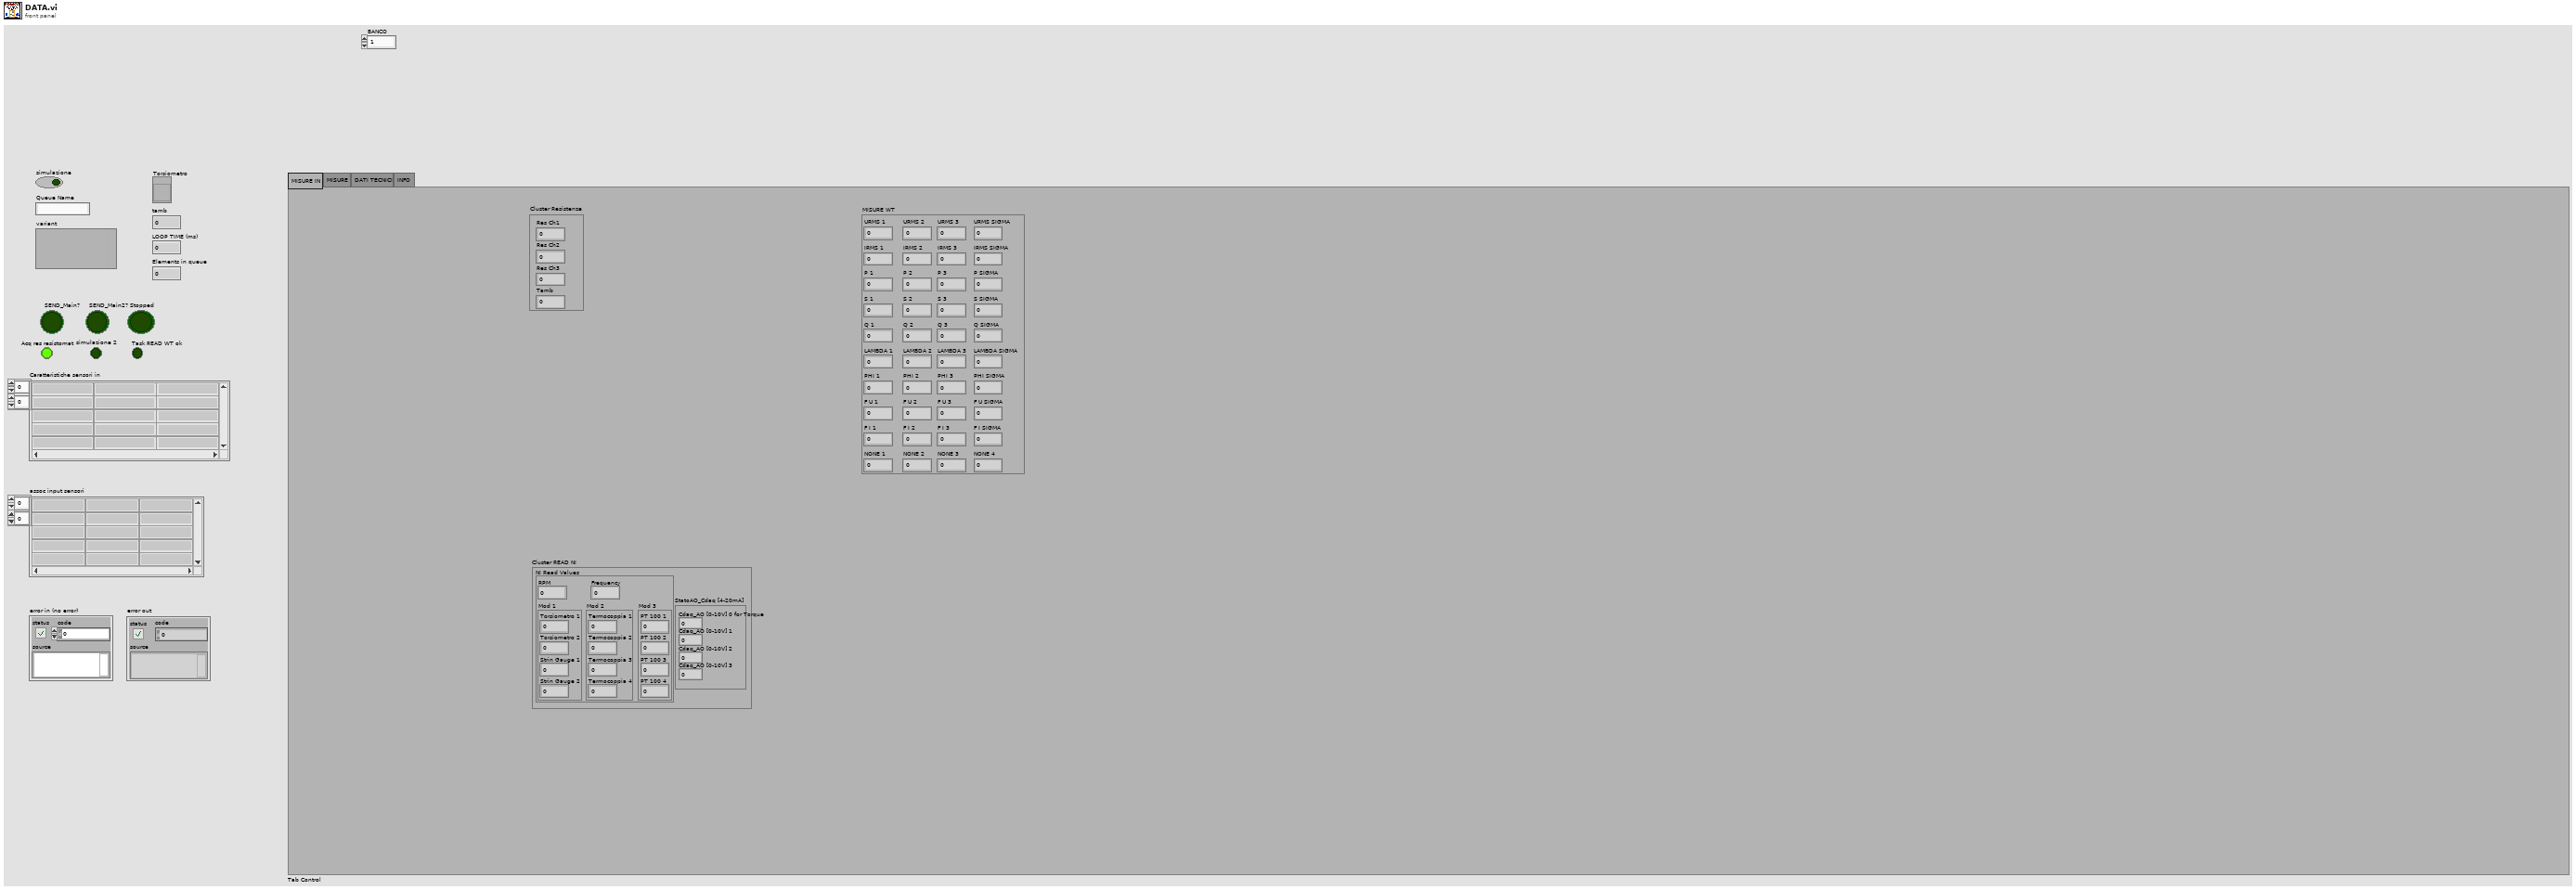
[diagram p1: front panel]
types:
  T1 = typedef "Cluster NI.ctl" = cluster{"AI (0-10V)":cluster{"AI 0":dbl, "AI 1":dbl, "AI 2":dbl, "AI 3":dbl, "AI 4":dbl, "AI 5":dbl, "AI 6":dbl, "AI 7":dbl, "AI 8":dbl, "AI 9":dbl, "AI 10":dbl, "AI 11":dbl, "AI 12":dbl, "AI 13":dbl, "AI 14":dbl, "AI 15":dbl, "AI 16":dbl, "AI 17":dbl, "AI 18":dbl, "AI 19":dbl, "AI 20":dbl, "AI 21":dbl, "AI 22":dbl, "AI 23":dbl, "AI 24":dbl, "AI 25":dbl, "AI 26":dbl, "AI 27":dbl, "AI 28":dbl, "AI 29":dbl, "AI 30":dbl, "AI 31":dbl}, "StatoAO_Cdaq[0-10V]":cluster{"AO 1":dbl, "AO 2":dbl, "AO 3":dbl, "AO 4":dbl}, "Contatori [rpm]":cluster{"RPM 1":dbl, "RPM 2":dbl}, "StatoAO_Cdaq [4-20mA]":T2, "StatoDO_Cdaq":T3, "DI":cluster{"Scorta 0":bool, "Scorta 1":bool, "Scorta 2":bool, "Scorta 3":bool, "Scorta 4":bool, "Scorta 5":bool, "Scorta 6":bool, "Scorta 7":bool, "Scorta 8":bool, "Scorta 9":bool, "Scorta 10":bool, "Scorta 11":bool, "Scorta 12":bool, "Scorta 13":bool, "Scorta 14":bool, "Scorta 15":bool, "Scorta 16":bool, "Scorta 17":bool, "Scorta 18":bool, "Scorta 19":bool, "Scorta 20":bool, "Scorta 21":bool, "Scorta 22":bool, "Scorta 23":bool, "Scorta 24":bool, "Scorta 25":bool, "Scorta 26":bool, "Scorta 27":bool, "Scorta 28":bool, "Scorta 29":bool, "Scorta 30":bool, "Scorta 31":bool}, "AI (4-20mA)":cluster{"AI 0":dbl, "AI 1":dbl, "AI 2":dbl, "AI 3":dbl, "AI 4":dbl, "AI 5":dbl, "AI 6":dbl, "AI 7":dbl, "AI 8":dbl, "AI 9":dbl, "AI 10":dbl, "AI 11":dbl, "AI 12":dbl, "AI 13":dbl, "AI 14":dbl, "AI 15":dbl}, "TC [°C]":cluster{"tc 1":dbl, "tc 2":dbl, "tc 3":dbl, "tc 4":dbl}, "NI Read Values":cluster{"RPM":dbl, "Frequency":dbl, "Mod 1":cluster{"Torsiometro 1":dbl, "Torsiometro 2":dbl, "Strin Gauge 1":dbl, "Strin Gauge 2":dbl}, "Mod 2":cluster{"Termocoppia 1":dbl, "Termocoppia 2":dbl, "Termocoppia 3":dbl, "Termocoppia 4":dbl}, "Mod 3":cluster{"PT 100 1":dbl, "PT 100 2":dbl, "PT 100 3":dbl, "PT 100 4":dbl}}}
  T2 = typedef "StatoAO_cdaq.ctl" = cluster{"Cdaq_AO [0-10V] 0 for Torque":dbl, "Cdaq_AO [0-10V] 1":dbl, "Cdaq_AO [0-10V] 2":dbl, "Cdaq_AO [0-10V] 3":dbl}
  T3 = typedef "statoDO_Cdaq.ctl" = cluster{"Scorta 0":bool, "Scorta 1":bool, "Scorta 2":bool, "Scorta 3":bool, "Scorta 4":bool, "Scorta 5":bool, "Scorta 6":bool, "Scorta 7":bool, "Scorta 8":bool, "Scorta 9":bool, "Scorta 10":bool, "Scorta 11":bool, "Scorta 12":bool, "Scorta 13":bool, "Scorta 14":bool, "Scorta 15":bool, "Scorta 16":bool, "Scorta 17":bool, "Scorta 18":bool, "Scorta 19":bool, "Scorta 20":bool, "Scorta 21":bool, "Scorta 22":bool, "Scorta 23":bool, "Scorta 24":bool, "Scorta 25":bool, "Scorta 26":bool, "Scorta 27":bool, "Scorta 28":bool, "Scorta 29":bool, "Scorta 30":bool, "Scorta 31":bool}
  T4 = enum32{"MISURE IN", "MISURE", "DATI TECNICI", "INFO"}
  T5 = typedef "ClusterRes.ctl" = cluster{"Res Ch1":dbl, "Res Ch2":dbl, "Res Ch3":dbl, "Tamb":dbl}
  T6 = typedef "MISURE WT.ctl" = cluster{"URMS 1":dbl, "IRMS 1":dbl, "P 1":dbl, "S 1":dbl, "Q 1":dbl, "LAMBDA 1":dbl, "PHI 1":dbl, "F U 1":dbl, "F I 1":dbl, "NONE 1":dbl, "URMS 2":dbl, "IRMS 2":dbl, "P 2":dbl, "S 2":dbl, "Q 2":dbl, "LAMBDA 2":dbl, "PHI 2":dbl, "F U 2":dbl, "F I 2":dbl, "NONE 2":dbl, "URMS 3":dbl, "IRMS 3":dbl, "P 3":dbl, "S 3":dbl, "Q 3":dbl, "LAMBDA 3":dbl, "PHI 3":dbl, "F U 3":dbl, "F I 3":dbl, "NONE 3":dbl, "URMS SIGMA":dbl, "IRMS SIGMA":dbl, "P SIGMA":dbl, "S SIGMA":dbl, "Q SIGMA":dbl, "LAMBDA SIGMA":dbl, "PHI SIGMA":dbl, "F U SIGMA":dbl, "F I SIGMA":dbl, "NONE 4":dbl}
  T7 = typedef "Cluster MISURE.ctl" = cluster{"MISURE NM":T8, "MISURE ALL":T9}
  T8 = typedef "MISURE NM.ctl" = cluster{"Banco":string, "Anno":string, "Numero":string, "Ntabella":string, "Misura":string, "Tipo Prova":string, "ProgressivoAcq":string, "Descrizione":string, "Data_ora":string, "t. acq [h:m:s]":string, "t. acq [min]":string, "t. acq [s]":string, "n [rpm]":string, "f [Hz]":string, "U1[V]":string, "U2 [V]":string, "U3 [V]":string, "U123_media [V]":string, "I1[A]":string, "I2[A]":string, "I3[A]":string, "I123_media [A]*I":string, "I_123_sbil [%]":string, "Ulin[V]":string, "Uc [V]":string, "Uaux [V]":string, "Ilin[A]*I":string, "Imar[A]":string, "Iaux[A]":string, "Uarm[V]":string, "Uecc[V]":string, "Iarm[A]*I":string, "Iecc[A]":string, "pf":string, "P1 [W]":string, "P1 [kW]":string, "Q [VAR]":string, "Q [kVAR]":string, "S [VA]":string, "S [kVA]":string, "P1arm[W]":string, "P1ecc[W]":string, "Parm[kW]":string, "P1ecc[kW]":string, "Cond[uF]":string, "P1_linea_6fili[W]":string, "P1_linea_6fili[kW]":string, "eta_gr_6fili [%]":string, "eta_inverter_6fili [%]":string, "pf_linea_6fili":string, "U4 [V]":string, "U5 [V]":string, "U6 [V]":string, "U456_media [V]":string, "I4 [A]":string, "I5 [A]":string, "I6 [A]":string, "I456_media [A]":string, "C [Nm]*C":string, "Cric [Nm]":string, "Cric\\Cnom":string, "Iric[A]":string, "Iric\\Inom":string, "P2_mecc [W]":string, "P2_mecc [kW]":string, "eta motore [%]":string, "Scorr[%]":string, "Tamb[°C]":string, "R1[ohm]":string, "R2[ohm]":string, "R3[ohm]":string, "Rmedia[ohm]":string, "DT_R1[°C]":string, "DT_R2[°C]":string, "DT_R3[°C]":string, "DT_media[°C]":string, "R_marcia[ohm]":string, "R_aux[ohm]":string, "DT_marcia[°C]":string, "DT_aux[°C]":string, "R_Arm[ohm]":string, "R_Ecc[ohm]":string, "DT_Arm[°C]":string, "DT_Ecc[°C]":string, "TambFreddo[°C]":string, "R1_freddo[ohm]":string, "R2_freddo[ohm]":string, "R3_freddo[ohm]":string, "Rmedia_freddo[ohm]":string, "R_Marcia_freddo[ohm]":string, "R_Aux_freddo[ohm]":string, "R_Arm_freddo[ohm]":string, "R_Ecc_freddo[ohm]":string, "TC1 [°C]":string, "TC2 [°C]":string, "TC3 [°C]":string, "TC4 [°C]":string, "TC5 [°C]":string, "TC6 [°C]":string, "TC7 [°C]":string, "TC8 [°C]":string, "PT1000_1[°C]":string, "PT1000_2[°C]":string, "PT1000_3[°C]":string, "Vdc eccitatrice[V]":string, "Idc eccitatrice[A]":string, "Vdc rotore[V]":string, "Idc rotore[A]":string, "Vac rotore[V]":string, "Iac rotore[V]":string, "V dinamo[V]":string, "Portata Q":string, "Pressione H":string, "U1'[V]":string, "U2'[V]":string, "U3'[V]":string, "I1'[A]":string, "I2'[A]":string, "I3'[A]":string, "U''R-N":string, "U''S-N":string, "U'' T-N":string, "U''R-S":string, "U''R-T":string, "U''S-T":string, "I1''[A]":string, "I2''[A]":string, "I3''[A]":string, "F''[Hz]":string, "P''[kW]":string, "CosFi''":string, "PT1000_4[°C]":string, "Scorta 3":string}
  T9 = typedef "Cluster misure ALL.ctl" = cluster{"Cluster READ NI":T1, "MISURE WT":T6, "Resistenze Resistomat":T5, "INTERFACCIA":T10, "FREDDO resistomat":cluster{"Res Ch1":dbl, "Res Ch2":dbl, "tAMB":dbl, "Res Ch3":dbl}, "STATO PLC 1":T15, "Res Ch2":dbl, "Res Ch2 2":dbl, "FREDDO res meter":cluster{"Res Ch1":dbl, "Res Ch2":dbl, "tAMB":dbl, "Res Ch3":dbl}, "Resistenze Res Meter":T5, "READ SINUS PENTA":T19, "STATO PLC 2":T20, "STATO PLC 3":T24, "DCREG":T28}
  T10 = typedef "INTERFACCIA.ctl" = cluster{"AI":cluster{"Portate":T11[], "Pressioni":T11[], "Coppie[Nm]":T11[], "Valvole prop %":T11[], "RPM":T11[], "Livelli":T11[], "Temperature":T11[], "Riferimenti %":T11[], "TENSIONI":T11[], "CORRENTI":T11[]}, "DI (logici)":cluster{"Start da pulsantiera":bool, "Stop da pulsantiera":bool, "Reset da pulsantiera":bool, "Sistema OK":bool, "Collaudo abilitato":bool, "Potenza trifase abilitata":bool, "Potenza monofase abilitata":bool, "Potenza DC abilitata":bool, "Potenza DC ECC abilitata":bool, "Start alimentazione AC":bool, "Start alimentazione DC":bool, "Start DC eccitazione":bool, "Teleruttore WT abilitato":bool, "Teleruttore Resistomat abilitato":bool, "Teleruttore corto fasi":bool, "Ramo 1 resistomat":bool, "Ramo 2 resistomat":bool, "Ramo 3 resistomat":bool, "B1 Scelta linea elettrica 1":bool, "B1 Scelta linea elettrica 2":bool, "B1 Scelta linea elettrica 3":bool, "B1 Scelta linea elettrica 4":bool, "B1 Scelta linea elettrica 5":bool, "B2 Scelta linea elettrica 1":bool, "B2 Scelta linea elettrica 2":bool, "B2 Scelta linea elettrica 3":bool, "B2 Scelta linea elettrica 4":bool, "B2 Scelta linea elettrica 5":bool, "Rotore bloccato 1":bool, "Rotore bloccato 2":bool, "FRENO 1 abilitato":bool, "FRENO 1 run":bool, "FRENO 1 senso rotaz":bool, "FRENO 1 ctrl velocità":bool, "FRENO 2 abilitato":bool, "FRENO 2 run":bool, "FRENO 2 senso rotaz":bool, "FRENO 2 ctrl velocità":bool, "ALIM 1 abilitato":bool, "ALIM 1 run":bool, "ALIM 2 abilitato":bool, "ALIM 2 run":bool, "ALIM 3 abilitato":bool, "ALIM 3 run":bool, "FRENO 1 ctrl coppia":bool, "FRENO 2 ctrl coppia":bool, "FRENO 3 ctrl coppia":bool, "DI (logici) aggiuntivi impianto":cluster{"Solo freno abilitato":bool, "Carico resistivo abilitato":bool, "AFE+freno abilitato":bool, "Protezioni chiuse":bool, "Start potenza AFE":bool, "AFE in marcia":bool}, "Misura corrente diretta WT":bool, "Misura corrente sens ext":bool, "Sens ext abilitati":bool}, "AO non scalati":T13, "AO scalati":T13, "DO (logici)":T14}
  T11 = typedef "ClusterMisura_e_Unità_INPUT.ctl" = cluster{"Misura":dbl, "UM":T12, "Descrizione":string}
  T12 = typedef "UnitàMisura.ctl" = enum16{"V", "mA", "Bar", "RPM", "m3/s", "m3/min", "m3/h", "l/s", "l/min", "in3/min", "ft3/min", "gpm", "igpm", "igph", "%", "°C", "m", "Nm", "A"}
  T13 = typedef "Lista AO sistema.ctl" = cluster{"FRENO1 rif vel":dbl, "FRENO1 rif Coppia":dbl, "FRENO2 rif vel":dbl, "FRENO2 rif Coppia":dbl, "ALIM1 rif V":dbl, "ALIM1 rif F":dbl, "ALIM2 rif V":dbl, "ALIM2 rif F":dbl, "ALIM3 rif V":dbl, "ALIM3 rif F":dbl, "Fnom keb":dbl, "Rpm nom keb":dbl, "Pnom keb":dbl, "Inom keb":dbl, "Vnom keb":dbl, "Rpm max keb":dbl, "Tempo rampa keb":dbl, "Tipo Mot keb":dbl, "FRENO  rif Coppia ":dbl, "FRENO  rif  Corrente":dbl}
  T14 = typedef "DOinterfaccia.ctl" = cluster{"Scelta banco 1":bool, "Scelta banco 2":bool, "Scelta banco 3":bool, "FRENO 1 abilita":bool, "FRENO 1 start":bool, "FRENO 1 senso rotaz":bool, "FRENO 1 ctrl velocità":bool, "FRENO 2 abilita":bool, "FRENO 2 start":bool, "FRENO 2 senso rotaz":bool, "FRENO 2 ctrl velocità":bool, "ALIM 1 abilita":bool, "ALIM 1 start":bool, "ALIM 2 abilita":bool, "ALIM 2 start":bool, "ALIM 3 abilita":bool, "ALIM 3 start":bool, "Abilita linea trifase":bool, "Abilita linea monofase":bool, "Abilita linea dc":bool, "Abilita linea dc eccit":bool, "B1 Linea elettrica 1":bool, "B1 Linea elettrica 2":bool, "B1 Linea elettrica 3":bool, "B1 Linea elettrica 4":bool, "B1 Linea elettrica 5":bool, "B2 Linea elettrica 1":bool, "B2 Linea elettrica 2":bool, "B2 Linea elettrica 3":bool, "B2 Linea elettrica 4":bool, "B2 Linea elettrica 5":bool, "Start potenza AC":bool, "Stop pontenza AC":bool, "Start potenza DC":bool, "Stop potenza DC":bool, "Start potenza eccitaz":bool, "Stop potenza eccitaz":bool, "Reset allarmi":bool, "watchdog":bool, "Scala torsiometro B1":bool, "Controllo torsiom B1":bool, "Scala torsiometro B2":bool, "Controllo torsiom B2":bool, "Teleruttore WT abilita":bool, "Teleruttore Resistomat abilita":bool, "Teleruttore corto fasi":bool, "Ramo 1 resistomat":bool, "Ramo 2 resistomat":bool, "Ramo 3 resistomat":bool, "Collaudo in corso":bool, "Allarme presente":bool, "Enable Res Meter":bool, "Bypass Res Meter":bool, "2nd canale Res Meter":bool, "Scala 200/2000 res meter":bool, "Taratura res meter":bool, "FRENO 1 ctrl coppia":bool, "FRENO 2 ctrl coppia":bool, "FRENO 3 ctrl coppia":bool, "Aggiuntivi impianto":cluster{"Senso rotazione alim 1":bool, "Senso rotazione alim 2":bool}, "ALIM 1 stop":bool, "ALIM 2 stop":bool, "ALIM 3 stop":bool, "FRENO 1 stop":bool, "FRENO 2 stop":bool, "FRENO 3 stop":bool, "B1 configurazione freno B":bool, "B2 configurazione freno B":bool, "Abilita scrittura KEB":bool, "Bench Selection (0-B1,1-B2)":bool, "Select current mode":bool, "Select torque mode":bool, "Select speed mode":bool, "Start":bool, "Stop":bool, "Block":bool, "Enable Force mode":bool, "Abilita linea 125 A":bool, "Abilita linea 63 A":bool, "Abilita linea 16 A":bool, "Aum Tensione Variac":bool, "Dim Tesnione Variac":bool, "Abilita ellectro stractura":bool, "Risprinito Emergence":bool, "Abilita collaudo":bool, "Disabilita collaudo":bool, "External Alaram":bool, "Enable external program":bool, "Reset":bool, "Abilita Ingresso Variac":bool, "Abilita Ventilatore Variac":bool, "Abilita Uscita Variac ":bool}
  T15 = typedef "STATO PLC 1.ctl" = cluster{"USCITE PLC":T16, "Stato DI_PLC":cluster{"Sistema OK":bool, "Rotore bloccato":bool, "Scorta 1":bool, "Prova diretto inverter":bool, "Prova con filtro LC":bool, "Teleruttore WT abilitato":bool, "Alim sinus penta abilitato":bool, "Alim sinus penta in marcia":bool, "Freno abilitato":bool, "Freno in marcia":bool, "Senso rotazione freno":bool, "Potenza abilitata":bool, "Scorta 3":bool, "Scorta 4":bool, "scorta 5":bool, "scorta 6":bool}, "AI plc":cluster{"Allarmi 1":dbl, "Allarmi 2":dbl, "Scorta 1":dbl, "Scorta 2":dbl, "RPM mot prova":dbl, "I mot prova":dbl, "RPM freno":dbl, "I freno":dbl, "Scorta 3":dbl, "Scorta 4":dbl}}
  T16 = typedef "Uscite PLC 1.ctl" = cluster{"AO (real) 2":cluster{"SCORTA 1":dbl, "SCORTA 2":dbl, "SCORTA 3":dbl, "SCORTA 4":dbl, "SCORTA 5":dbl, "SCORTA 6":dbl, "SCORTA 7":dbl, "SCORTA 8":dbl}, "statoAO_PLC out":T17, "DO (bit)":T18}
  T17 = typedef "statoAO_plc_1.ctl" = cluster{"Rif Lim coppia freno [%]":dbl, "Rif rpm freno [%]":dbl, "Rif coppia freno [%]":dbl, "Rif V alimentatore [%]":dbl, "Rif F alimentatore [%]":dbl}
  T18 = typedef "StatoDO_PLC_1.ctl" = cluster{"Scelta banco 1":bool, "Set dati motore freno 2":bool, "Diretto inverter":bool, "Filtro LC":bool, "Marcia ALIM (1s)":bool, "Marcia FRENO (1s)":bool, "Stop AFE (1s)":bool, "Stop freno (1s)":bool, "Reset allarmi":bool, "Watchdog":bool, "Senso rotazione":bool, "Abilita collaudo (1s)":bool, "Disabilita collaudo (1s)":bool, "Abilitazione ALIM":bool, "Abilitazione FRENO":bool, "Teleruttore WT":bool, "Senso rot motore prova":bool, "Scorta 7":bool, "Scorta 8":bool, "Scorta 9":bool, "Scorta 10":bool, "Scorta 11":bool, "Scorta 12":bool, "Scorta 13":bool}
  T19 = typedef "Parametri inverter letti.ctl" = cluster{"Menù Misure motore (M000-M030)":cluster{"Rif vel a regime (int)":u16, "Rif vel a regime (dec)":u16, "Rif vel dopo rampe (int)":u16, "Rif vel dopo rampe (dec)":u16, "RPM motore (int)":u16, "RPM motore (dec)":u16, "FREQout inverter":u16, "Rif coppia a regime(Nm)":u16, "Richiesta di coppia (Nm)":u16, "Coppia generata dal motore(Nm)":u16, "Rif coppia a regime(%)":u16, "Richiesta di coppia (%)":u16, "Coppia generata dal motore(%)":u16, "Coppia max richiesta prima delle rampe(Nm)":u16, "Coppia max richiesta dopo le rampe(Nm)":u16, "Limite di velocità prima delle rampe":u16, "Limite di velocità dopo le rampe":u16, "Coppia max richiesta prima delle rampe(%)":u16, "Coppia max richiesta dopo le rampe(%)":u16, "Rif di flusso":u16, "Corrente di uscita":u16, "Capacità termica del motore":u16, "Tensione di uscita":u16, "Potenza di uscita":u16, "Energia consumata (LSword)":u16, "Energia consumata (MSword)":u16, "Tensione bus DC":u16, "Tensione di rete":u16}, "Menù regolatore PID (M018-M024)":cluster{"Rif PID a regime(%)":u16, "Rif pid dopo rampe(%)":u16, "Retroazione del pid(%)":u16, "Errore del pid(%)":u16, "uscita del pid(%)":u16, "Rif del pid dopo le rampe":u16, "Retroazione del pid":u16}, "Menù ingressi digitali (M031-M036)":cluster{"Ingressi digitali ritardati":u16, "Ingressi digitali istantanei":u16, "Moresettiera comando loc":u16, "Morsett comando da seriale":u16, "Morsett comando bus di campo":u16, "Ing dig ausiliari da morsettiera":u16, "Ing dig ausiliari da seriale":u16}, "Menù riferimenti (M037-M051)":cluster{"Rif analog est REF":u16, "Rif analog est AIN1":u16, "Rif analog est AIN2":u16, "Rif analog est XAIN4":u16, "Rif analog est XAIN5":u16, "Rif velocità da seriale(int)":u16, "Rif velocità bus di campo(int)":u16, "Rif coppia da seriale":u16, "Rif coppia bus di campo":u16, "Rif del PID da seriale":u16, "Rif del PID da bus di campo":u16, "Retroazione del PID da seriale":u16, "Retroazione del PIDda bus di campo":u16, "Rif da encoder":u16, "Rif in frequenza":u16, "Rif velocità da seriale(dec)":u16, "Rif velocità bus di campo(dec)":u16}, "Menù rampe (P009-P033)":cluster{"Tempo di dec rampa di vel 1":u16, "Tempo di acc rampa di vel 2":u16, "Tempo di dec rampa di vel 2":u16, "Tempo di acc rampa di vel 1":u16, "Unità di mis tempi rampe vel 1/2":u16, "Tempo di acc rampa di vel 3":u16, "Tempo di dec rampa di vel 3":u16, "Tempo di acc rampa di vel 4":u16, "Tempo di dec rampa di vel 4":u16, "Unità di mis tempi rampe vel 3/4":u16, "Selettore arrottondam rampe":u16, "Tempo di arrotond iniz rampa acc":u16, "Tempo di arrotond finale rampa acc":u16, "Tempo di arrotond iniz rampa dec":u16, "Tempo di rampa di salita rif coppia":u16, "Tempo di rampa di discesa rif coppia":u16, "Unità di misura rampa coppia":u16, "Tempo rampa acc marcia jog":u16, "Tempo rampa dec marcia jog":u16, "Reset acc ai cambi pendenza":u16, "rampa di acc in fire mode":u16, "rampa di dec in fire mode":u16, "Tempo di arrotond finale rampa dec":u16}, "Menù controllo motore(C008-C128)":cluster{"Numero motori configurati":u16, "Tipo algoritmo di controllo Mot1":u16, "Tipo rif Mot1":u16, "Tensione nominale rete":u16, "Retroaz di vel da encoder Mot1":u16, "Tipo curva V/f Mot1":u16, "Rotazione delle fasi Mot1":u16, "Freq nominale del motore Mot1":u16, "RPM nominali del motore Mot1":u16, "Potenza nominale del motore Mot1":u16, "Corrente nominale del motore Mot1":u16, "Tensione nominale del motore mot1":u16, "Potenza a vuoto del motore Mot1":u16, "Corrente a vuoto del motore Mot1":u16, "Resistenza statorica del motore Mot1":u16, "Induttanza di dispersione Mot1":u16, "Induttanza mutua motore":u16, "Costante di tempo rotorica":u16, "Costante di tempo filtro pb":u16, "Velocità minima motore":u16, "Velocità massima motore":u16}, "Menù configurazione PID":cluster{"Selezione riferimento n.1":u16, "Selezione retroazione n.1":u16, "Modalità di fuzionamento PID":u16, "Termine derivativo calcolato su err o mis":u16, "Proporz moltiplica deriv e integrale":u16, "Azione del PID":u16}, "ID":dbl, "Menù uscite digitali":cluster{"MDO4 Inverter pronto":u16}, "Fcarrier":cluster{"Fcarrier Min (Hz)":u16, "Fcarrier Max (Hz)":u16}, "stato inverter M089":dbl, "Riferimenti":cluster{"Rif tensione":u16, "Rif velocità":u16}, "Comunicazione":bool, "Modalità stop":dbl}
  T20 = typedef "STATO PLC 2.ctl" = cluster{"USCITE PLC":T21, "Stato DI_PLC":cluster{"Sistema ok":bool, "Relè Resistomat abilitato":bool, "Freno abilitato":bool, "Freno in marcia":bool, "scorta b":bool, "scorta a":bool, "scorta 1":bool, "scorta 2":bool, "scorta 3":bool, "scorta 4":bool, "Scorta 5":bool, "Scorta 6":bool, "Scorta 7":bool, "Scorta 8":bool, "Scorta 9":bool, "Scorta 10":bool}, "AI plc":cluster{"Allarmi 1":dbl, "Allarmi 2":dbl, "TC 1":dbl, "TC 2":dbl, "TC 3":dbl, "TC 4":dbl, "TC 5":dbl, "TC 6":dbl, "TC 7":dbl, "TC 8":dbl, "PT1000 1":dbl, "PT1000 2":dbl, "PT1000 3":dbl, "PT1000 4":dbl}}
  T21 = typedef "Uscite PLC 2.ctl" = cluster{"AO (real) 2":cluster{"SCORTA 1":dbl, "SCORTA 2":dbl, "SCORTA 3":dbl, "SCORTA 4":dbl, "SCORTA 5":dbl, "SCORTA 6":dbl, "SCORTA 7":dbl, "SCORTA 8":dbl}, "statoAO_PLC out":T22, "DO (bit)":T23}
  T22 = typedef "statoAO_plc_2.ctl" = cluster{"Condensatori":dbl, "Scorta 1":dbl, "Scorta 2":dbl}
  T23 = typedef "StatoDO_PLC_2.ctl" = cluster{"Relè misura resistomat":bool, "Misura res ramo 1":bool, "Misura res ramo 2":bool, "Misura res ramo 3":bool, "Scelta banco 2":bool, "Scala Torsiometro":bool, "Ctrl torsiometro":bool, "Select current mode":bool, "Select Torque mode":bool, "Select speed mode":bool, "Watchdog":bool, "Scorta":bool, "Scorta 2":bool, "Scorta 3":bool, "Scorta 4":bool, "Scorta 5":bool, "Bench selection":bool, "External alarm":bool, "Enable external program":bool, "Reset allarmi":bool, "Start":bool, "Stop":bool, "Block":bool, "Scorta 6":bool}
  T24 = typedef "STATO PLC 3.ctl" = cluster{"USCITE PLC":T25, "Stato DI_PLC":cluster{"Sistema OK":bool, "Rotore bloccato":bool, "Filtro LC":bool, "Bypass Filtro LC":bool, "Scelta Trasformatore":bool, "Scelta Bypass trasformatore":bool, "Teleruttore wt abilitato":bool, "Alimentatore abilitato":bool, "Alimentatore in marcia":bool, "Scorta 1":bool, "Scorta 2":bool, "Scorta 3":bool, "Potenza abilitata":bool, "Alimentatore in allarme":bool, "Scorta 4":bool, "Conferma dati KEB":bool, "Scorta 5":bool, "Warning Inverter Alimentatore":bool, "Variac Abilitato":bool, "Linea 125 A abilitata":bool, "Linea 63 A abilitata":bool, "Linea 16 A abilitata":bool, "Scorta 6":bool, "Enable force mode":bool}, "AI plc":cluster{"Allarmi 1":dbl, "Allarmi 2":dbl, "RPM motore prova":dbl, "Corrente motore prova":dbl, "RPM freno":dbl, "Corrente freno":dbl, "Tipo motore keb":dbl, "I nom keb":dbl, "RPM nom keb":dbl, "V nom keb":dbl, "F nom keb":dbl, "T rampa keb":dbl, "scorta":dbl, "Scorta 2":dbl}}
  T25 = typedef "Uscite PLC 3.ctl" = cluster{"AO (real) 2":cluster{"SCORTA 1":dbl, "SCORTA 2":dbl, "SCORTA 3":dbl, "SCORTA 4":dbl, "SCORTA 5":dbl, "SCORTA 6":dbl, "SCORTA 7":dbl, "SCORTA 8":dbl}, "statoAO_PLC out":T26, "DO (bit)":T27}
  T26 = typedef "statoAO_plc_3.ctl" = cluster{"Rif velocità alimentatore":dbl, "Scorta":dbl, "Tipo Motore  keb":dbl, "I nom keb":dbl, "RPM nom keb":dbl, "V nom keb":dbl, "F nom keb":dbl, "t rampa keb":dbl}
  T27 = typedef "StatoDO_PLC_3.ctl" = cluster{"Select linea Inverter":bool, "Abilita sense wattmetro":bool, "Bypass filtro LC":bool, "Filtro LC":bool, "Bypass trasformatore":bool, "Trasformatore":bool, "Abilita uscite variac":bool, "Abilita linea 125 A":bool, "Abilita linea 63 A":bool, "Abilita linea 16 A":bool, "Abilita Scrittura Dati Keb":bool, "Abilita alimentatore":bool, "Marcia alimentatore (1s)":bool, "Stop alimentatore (1s)":bool, "Senso rot mot prova":bool, "Watchdog":bool, "Aumenta tensione variac":bool, "Diminuisci tensione variac ":bool, "Blocco elettroserrature":bool, "Ripristino emergence":bool, "Abilita ingresso variac":bool, "Abilita ventilatore variac":bool, "Reset Allarm":bool, "Scorta 1":bool, "Scorta 2":bool, "Scorta 3":bool, "Scorta 4":bool, "Scorta 5":bool, "Scorta 6":bool, "Scorta 7":bool, "Scorta 8":bool, "Scorta 9":bool, "Abilita collaudo":bool, "Disabilita collaudo ":bool, "Scorta 10":bool, "Scorta 11":bool, "Scorta 12":bool, "Scorta 13":bool, "Scorta 14":bool, "Scorta 15":bool}
  T28 = typedef "Parametri DCREG letti.ctl" = cluster{"Parametri di misura":cluster{"M000":dbl, "M001":dbl, "M002":dbl, "M003":dbl, "M004":dbl, "M005":dbl, "M006":dbl, "M007":dbl, "M008":dbl, "M009":dbl, "M010":dbl, "M011":dbl, "M012":dbl, "M013":dbl, "M014":dbl, "M015":dbl, "M016":dbl, "M017":dbl, "M018":dbl, "M019":dbl, "M020":dbl, "M021":dbl, "M022":dbl, "M023":dbl, "M024":dbl, "M025":dbl, "M026":dbl, "M027":dbl, "M028":dbl, "M029":dbl, "M030":dbl, "M031":dbl}, "Parametri di programmazione":cluster{"P000":dbl, "P001":dbl, "P002":dbl, "P003":dbl, "P004":dbl, "P005":dbl, "P006":dbl, "P010":dbl, "P011":dbl, "P012":dbl, "P013":dbl, "P014":dbl, "P015":dbl, "P016":dbl, "P030":dbl, "P031":dbl, "P032":dbl, "P033":dbl, "P034":dbl, "P035":dbl, "P036":dbl, "P037":dbl, "P038":dbl, "P039":dbl, "P040":dbl, "P050":dbl, "P051":dbl, "P052":dbl, "P053":dbl, "P054":dbl, "P055":dbl, "P056":dbl, "P057":dbl, "P058":dbl, "P059":dbl, "P060":dbl, "P061":dbl, "P062":dbl, "P070":dbl, "P071":dbl, "P073":dbl, "P074":dbl, "P076":dbl, "P077":dbl, "P079":dbl, "P080":dbl, "P082":dbl, "P083":dbl, "P084":dbl, "P085":dbl, "P086":dbl, "P087":dbl, "P088":dbl, "P100":dbl, "P101":dbl, "P102":dbl, "P103":dbl, "P104":dbl, "P110":dbl, "P111":dbl, "P120":dbl, "P121":dbl, "P122":dbl, "P123":dbl, "P124":dbl, "P125":dbl, "P126":dbl, "P127":dbl, "P128":dbl, "P129":dbl, "P130":dbl, "P131":dbl, "P132":dbl, "P133":dbl, "P134":dbl, "P150":dbl, "P151":dbl, "P152":dbl, "P153":dbl, "P154":dbl, "P155":dbl, "P156":dbl, "P157":dbl, "P158":dbl, "P170":dbl, "P171":dbl, "P172":dbl, "P173":dbl, "P174":dbl, "P175":dbl, "P176":dbl, "P177":dbl, "P178":dbl, "P179":dbl, "P180":dbl, "P181":dbl, "P182":dbl, "P183":dbl, "P184":dbl, "P185":dbl, "P186":dbl, "P187":dbl, "P188":dbl, "P189":dbl, "P190":dbl, "P191":dbl, "P192":dbl, "P193":dbl, "P194":dbl, "P195":dbl, "P196":dbl, "P197":dbl, "P198":dbl, "P199":dbl, "P211":dbl, "P212":dbl, "P213":dbl, "P214":dbl, "P215":dbl, "P216":dbl, "P217":dbl, "P221":dbl, "P222":dbl, "P223":dbl, "P224":dbl, "P230":dbl, "P231":dbl, "P240":dbl, "P250":dbl, "P251":dbl}, "Parametri di configurazione":cluster{"C000":dbl, "C001":dbl, "C002":dbl, "C010":dbl, "C011":dbl, "C012":dbl, "C014":dbl, "C015":dbl, "C016":dbl, "C017":dbl, "C018":dbl, "C030":dbl, "C050":dbl, "C051":dbl, "C052":dbl, "C060":dbl, "C061":dbl, "C062":dbl, "C063":dbl, "C070":dbl, "C072":dbl, "C074":dbl, "C090":dbl, "C091":dbl, "C092":dbl, "C093":dbl, "C094":dbl, "C100":dbl, "C101":dbl, "C102":dbl, "C103":dbl, "C105":dbl, "C106":dbl, "C107":dbl, "C108":dbl, "C110":dbl, "C111":dbl, "C112":dbl, "C120":dbl, "C121":dbl, "C122":dbl, "C130":dbl, "C131":dbl, "C132":dbl, "C133":dbl, "C134":dbl, "C135":dbl, "C141":dbl, "C142":dbl, "C143":dbl, "C150":dbl, "C151":dbl, "C153":dbl, "C154":dbl, "C155":dbl, "C156":dbl, "C157":dbl, "C158":dbl, "C159":dbl, "C160":dbl, "C161":dbl, "C162":dbl, "C163":dbl, "C164":dbl, "C165":dbl, "C170":dbl}, "Codice allarme":dbl, "Comunicazione":bool}
  T29 = cluster{"Numero":dbl, "Data":dbl, "Test Engineer":dbl, "Cliente":dbl, "Tipo Pompa":dbl, "Costruttore":dbl, "n°serie":dbl, "Q [GPM]":dbl, "H [PSI]":dbl, "n [RPM]":dbl, "Diametro girante":dbl, "Linea asp. [mm]":dbl, "Linea prem. [mm]":dbl, "Dislivello [mm]":dbl, "Note1":dbl, "Note2":dbl, "Note3":dbl, "Note4":dbl, "n°giranti":dbl, "D1 girante [mm]":dbl, "B2 girante [mm]":dbl, "materiale":dbl, "oring":dbl, "mod.girante":dbl, "mod.lcorpo p":dbl, "Note5":dbl, "Note6":dbl}
  T30 = cluster{"Numero":dbl, "Tipo Pompa":dbl, "Costruttore":dbl, "n°serie":dbl, "Tipo Motore":dbl, "Costruttore":dbl, "n°serie":dbl, "Tipologia":dbl, "Tipo Inverter":dbl, "Costruttore":dbl, "n°serie":dbl, "Tipologia":dbl, "Data":dbl, "Nome Cliente":dbl, "Test Engineer":dbl, "Q1 [m3/h]":dbl, "H1 [m]":dbl, "Q2 [m3/h]":dbl, "H2 [m]":dbl, "Qmax [m3/h]":dbl, "Hmax [m]":dbl, "n° giranti":dbl, "MEI":dbl, "EEI":dbl, "IE":dbl, "fn [Hz]":dbl, "Un [V]":dbl, "In [A]":dbl, "P1 [W]":dbl, "P2 [W]":dbl, "Crun [uF]":dbl, "Cstart [uF]":dbl, "Uc [V]":dbl, "Numero Poli":dbl, "n [rpm]":dbl, "Tn [Nm]":dbl, "pfn":dbl, "etp [p.u.]":dbl, "etg [p.u.]":dbl, "C.I.":dbl, "Collegamento":dbl, "Peso [kg]":dbl, "Servizio":dbl, "IP":dbl, "Ru-w [Ohm]":dbl, "Temp0 [°C]":dbl, "DTavv. [°C]":dbl, "DTcassa [°C]":dbl, "IIr [A]":dbl, "TIr [Nm]":dbl, "Note1":dbl, "Note2":dbl, "Note3":dbl, "Note4":dbl, "Dislivello [m]":dbl, "Tubo d1n [DN]":dbl, "Tubo d1 [mm]":dbl, "Tubo1 lungh [mm]":dbl, "Tubo1 rug1":dbl, "Tubo d2n [DN]":dbl, "Tubo d2 [mm]":dbl, "Tubo2 lungh [mm]":dbl, "Tubo2 rug1":dbl, "Cono1 d1 [mm]":dbl, "Cono1 d2 [mm]":dbl, "Cono1 l [mm]":dbl, "Cono2 d1 [mm]":dbl, "Cono2 d2 [mm]":dbl, "Cono2 l [mm]":dbl, "Note5":dbl, "Note6":dbl, "n° giranti":dbl, "D1 girante [mm]":dbl, "B2 girante [mm]":dbl, "materiale":dbl, "tenuta":dbl, "oring":dbl, "mod.girante":dbl, "mod.corpo p":dbl, "Note7":dbl, "Note8":dbl, "Pacco":dbl, "d int. [mm]":dbl, "d est. [mm]":dbl, "d est.rotore[mm]":dbl, "Traferro [mm]":dbl, "Costruzione":dbl, "Note9":dbl, "Note10":dbl, "f mod. [kHz]":dbl, "Mod. Pot. [A]":dbl, "Taglia [W]":dbl, "Tipologia":dbl}
  T31 = typedef "Cluster INFO.ctl" = cluster{"Scelta wattmetro":cluster{"Wattmetro":T32}, "SET RPM":dbl, "SET TEMP":dbl, "Array banchi":T33[], "Array valvole linee avvio/fermata":cluster{"Valvole avvio":cluster{"Set valvole avvio?":bool, "% valvole avvio":dbl[]}, "Valvole fermata":cluster{"Set valvole fermata?":bool, "% valvole fermata":dbl[]}}[], "banco selezionato":i8, "Nomi valvole prop sistema":string[], "canale-- sensore":string[][], "Attriti B1":dbl[][], "Attriti B2":dbl[][], "Collegamento elettrico":cluster{"ALIMENTAZIONE ELETTRICA":T34, "ID":i16, "#rami freddo\\eq term resmeter":i16, "#rami riscaldamento resmeter":i16, "#rami freddo\\eq term resistomat":i16, "#rami riscaldamento resistomat":i16, "CALCOLI":T35}, "lingua":i16, "Costanti collaudo":cluster{"P [bar]":dbl, "T amb. [°C]":dbl, "Umidità [%]":dbl, "T acqua [°C] 2":dbl}, "OPZIONI MISURE RES":cluster{"MISURA A FREDDO":enum16{"NESSUNO", "RESISTOMAT", "RES METER", "ENTRAMBI"}, "MISURA EQ. TERMICO":enum16{"NESSUNO", "RESISTOMAT", "RES METER", "ENTRAMBI"}, "MISURA DT PROVA IN CORSO":enum16{"NESSUNO", "RESISTOMAT - CON FERMATE", "RES METER - CON FERMATE", "RES METER - CONTINUO"}, "MISURE PRIMA E DOPO":enum16{"NESSUNO", "RESISTOMAT", "RES METER"}, "STRUMENTI PRESENTI":enum16{"NESSUNO", "RESISTOMAT", "RES METER", "ENTRAMBI"}}, "Dati targa motore":cluster{"Vnom":dbl, "Fnom":dbl, "Inom":dbl, "Cnom":dbl, "Npoli":dbl, "Scorta 1":dbl, "Scorta 2":dbl, "Scorta 3":dbl}}
  T32 = typedef "WT SELECTION.ctl" = enum32{"No Selection", "WT230", "WT333", "WT1800", "WT330", "VIW", "APLUS"}
  T33 = typedef "Definizione linea.ctl" = cluster{"Nome":string, "Tors. scala1":i32, "Tors. scala2":i32, "rpm":i32, "TAMB":i32, "Indici Temperature":i16[], "Indice freno":i16, "alimentatore trifase":i16, "alimentatore monofase":i16, "alimentatore dc arm":i16, "alimentatore dc ecc":i16, "alimentatore dc mp":i16}
  T34 = typedef "Collegamenti_elettrici.ctl" = enum16{"AC TRIFASE", "AC TRIFASE + FRENO", "AC MONOFASE", "DC CON ECCITAZIONE", "DC CON ECCITAZIONE + FRENO", "DC NO ECCITAZIONE", "DC NO ECCITAZIONE + FRENO", "FRENO TRASC + AFE", "SOLO FRENO", "CARICO RESISTIVO", "GENERICO", "SOLO ACQUISITORE", "SCORTA 4", "SCORTA 5", "SCORTA 6"}
  T35 = typedef "Control Calcoli.ctl" = enum16{"AC TRIFASE", "AC MONOFASE", "DC ECCITAZIONE", "DC NO ECCITAZIONE", "POMPA TRIFASE", "POMPA MONOFASE", "GENERICO", "TRASFORMATORE", "ALTERNATORE TRASCINATO", "GRUPPO ELETTROGENO"}
  T36 = enum16{"INITIALIZE", "MEDIA", "MEDIA TUTTO", "RESET BUFFER"}
  T37 = cluster{"Array of elements":cluster{"String":string, "variant":variant}[], "Single element":cluster{"String":string, "variant":variant}, "enque at\nopposite end (F)":bool, "no replications (F)":bool}
  T38 = cluster{"Res Ch1":dbl, "Res Ch2":dbl, "tAMB":dbl, "Res Ch3":dbl}
  T39 = typedef "sett T e R.ctl" = cluster{"Tamb[°C]":dbl, "Ru-w":dbl, "Rmarcia":dbl, "Raux":dbl, "Tamb Freddo[°C]":dbl, "Ru-w freddo":dbl, "Rmarcia freddo":dbl, "Raux freddop":dbl, "TC1":dbl, "TC2":dbl, "TC3":dbl, "TC4":dbl, "TC5":dbl, "TC6":dbl, "TC7":dbl, "TC8":dbl}
  T40 = cluster{"Cluster NPSH":refnum<vi>, "Cluster ctrl NPSH":refnum<vi>}
  T41 = cluster{"Value":bool, "Qref":dbl, "Htot ref":dbl, "MODALITA' SCELTA Qref Htot ref":enum32{"Imposta manualmente", "Parti da QH Freddo", "Parti da QH Regime"}}
  T42 = enum8{"Enabled", "Disabled", "Disabled and Grayed Out"}
  T43 = cluster{"RPM":dbl, "Frequency":dbl, "Mod 1":cluster{"Torsiometro 1":dbl, "Torsiometro 2":dbl, "Strin Gauge 1":dbl, "Strin Gauge 2":dbl}, "Mod 2":cluster{"Termocoppia 1":dbl, "Termocoppia 2":dbl, "Termocoppia 3":dbl, "Termocoppia 4":dbl}, "Mod 3":cluster{"PT 100 1":dbl, "PT 100 2":dbl, "PT 100 3":dbl, "PT 100 4":dbl}}
  T44 = enum32{"Imposta manualmente", "Parti da QH Freddo", "Parti da QH Regime"}
  T45 = typedef "cluster NPSH.ctl" = cluster{"Scostamento Q":dbl, "Scostamento Htot":dbl, "Q ref":dbl, "Htot ref":dbl}
  T46 = enum32{"Invalid", "Standard", "Closed", "Hidden", "Minimized", "Maximized"}
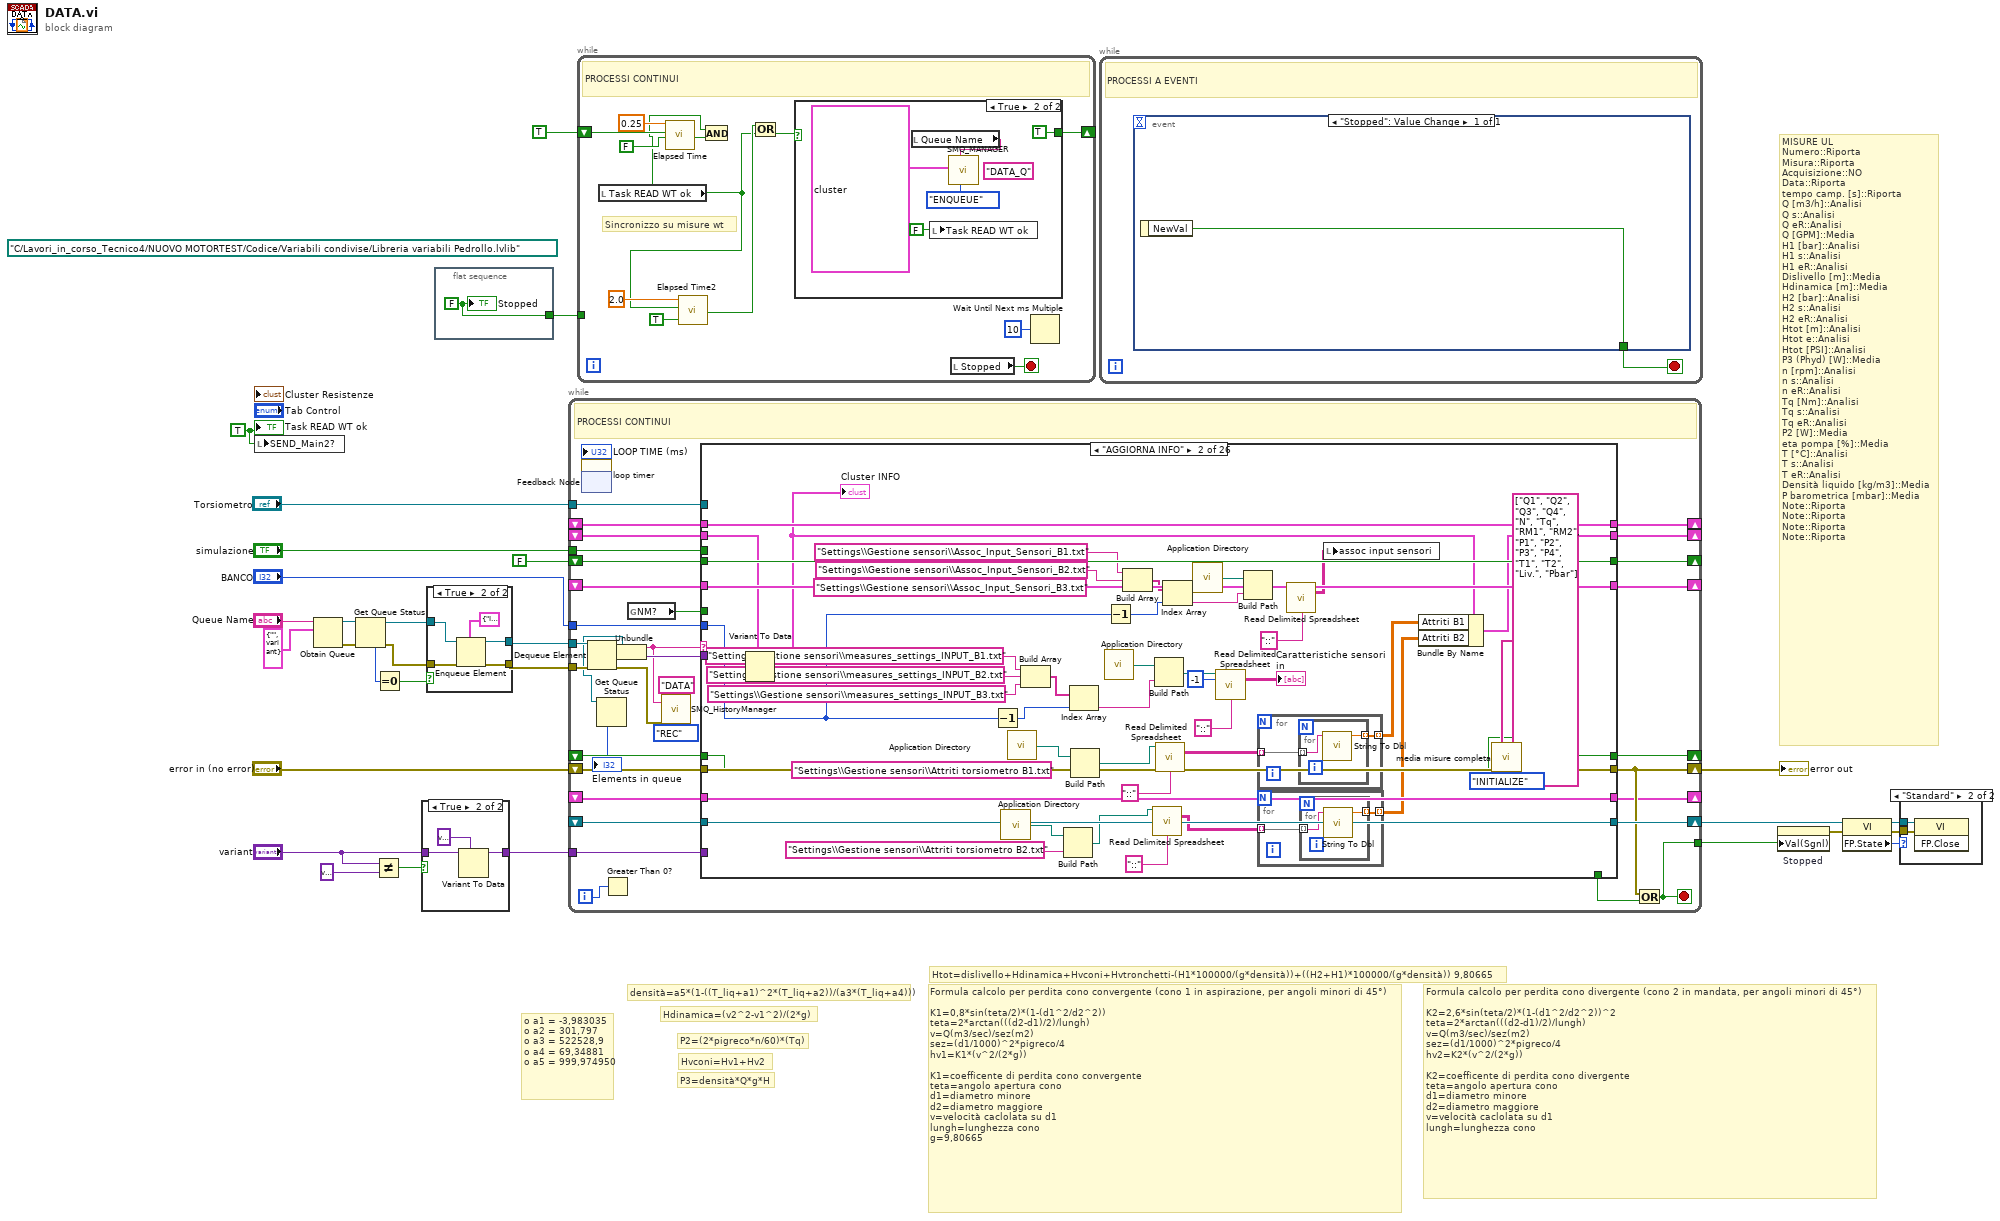
[diagram p0: block diagram]
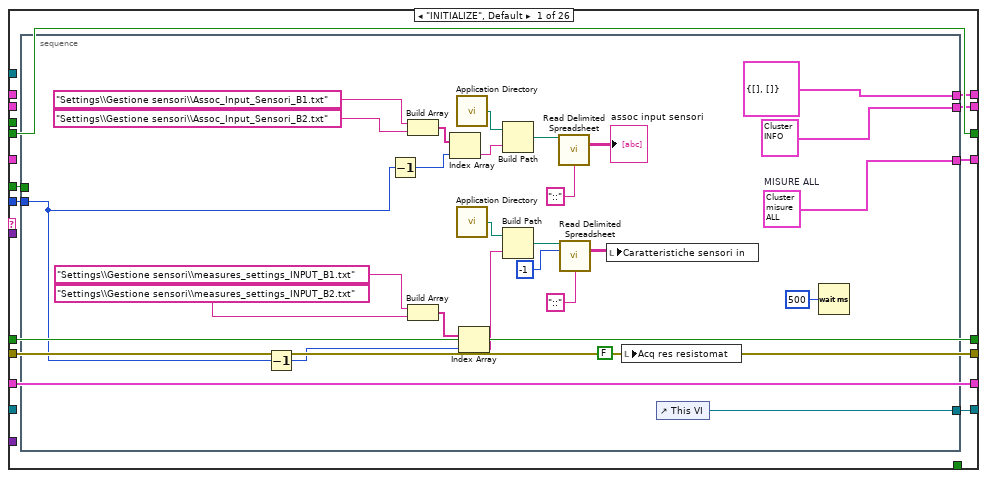
[diagram p6: hidden frame]
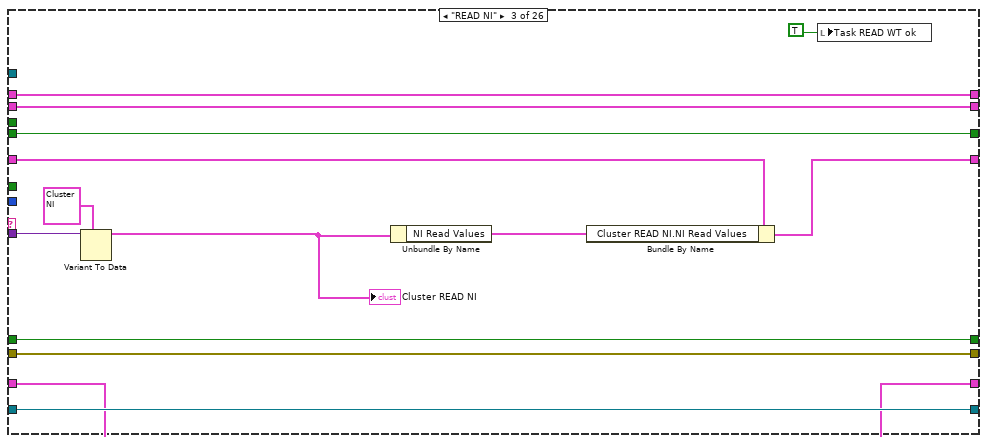
[diagram p7: hidden frame]
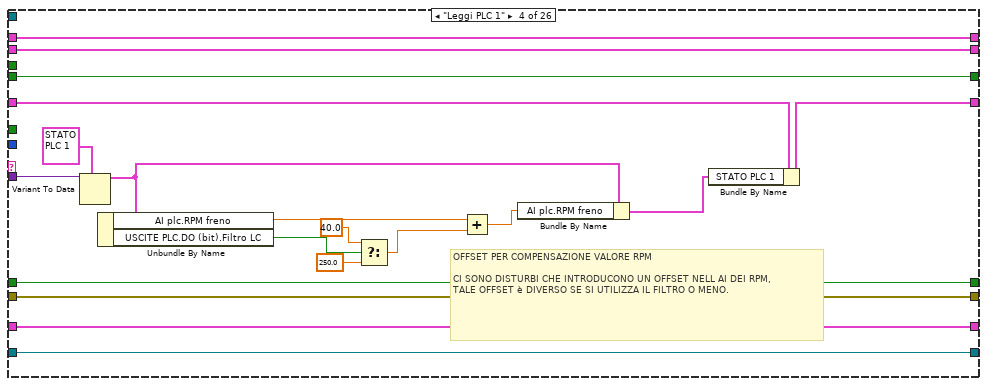
[diagram p8: hidden frame]
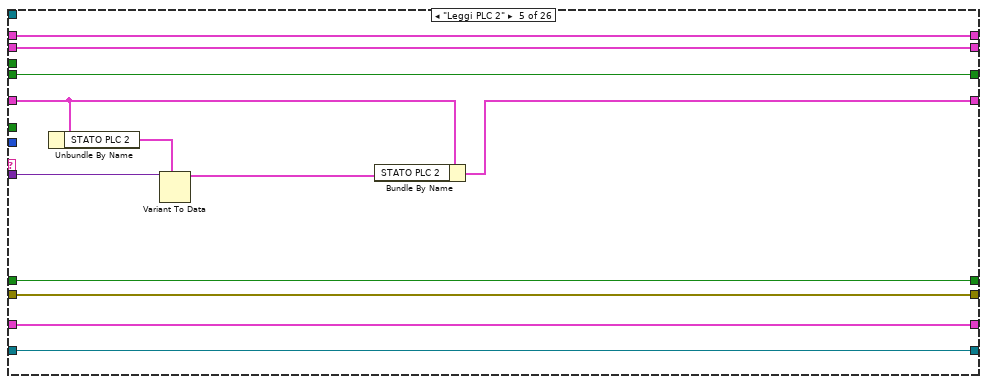
[diagram p9: hidden frame]
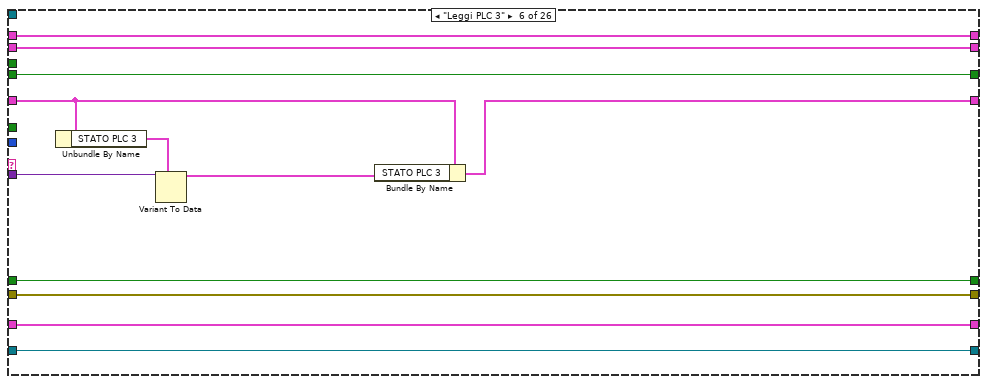
[diagram p10: hidden frame]
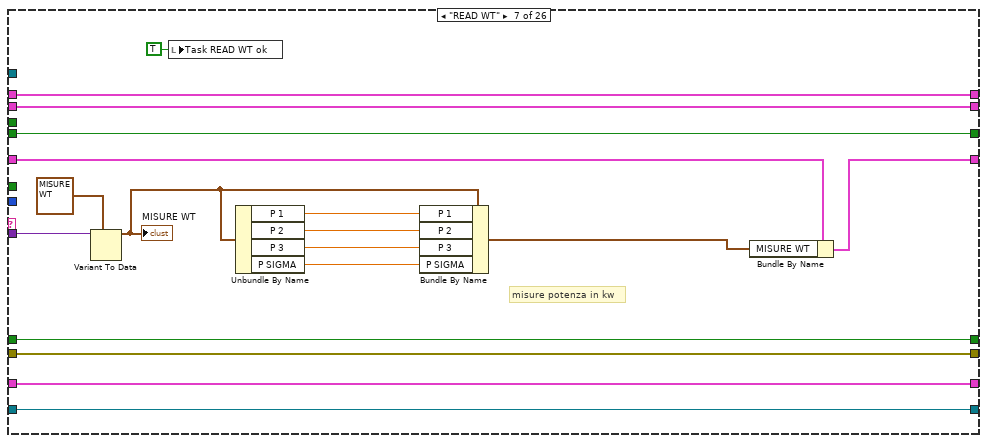
[diagram p11: hidden frame]
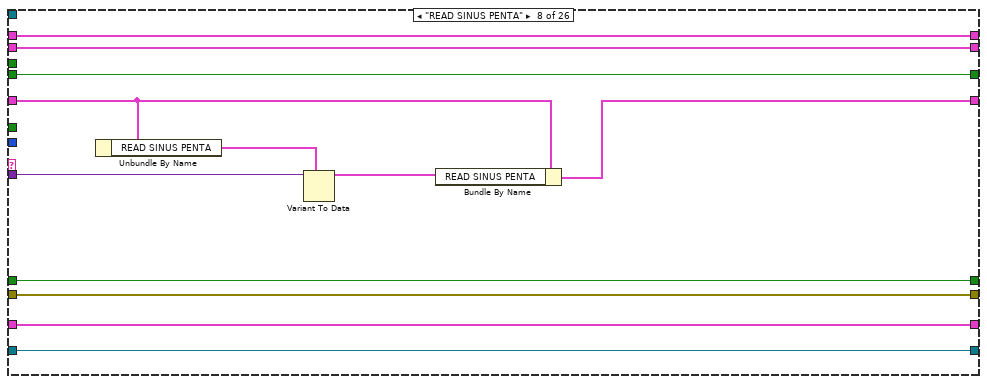
[diagram p12: hidden frame]
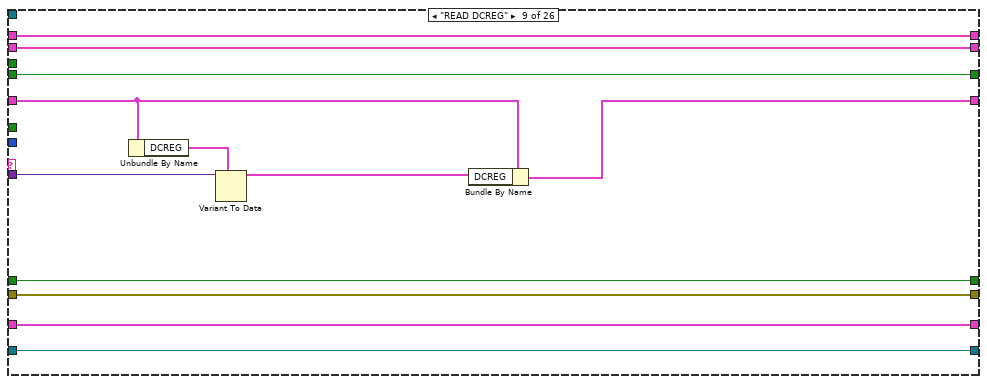
[diagram p13: hidden frame]
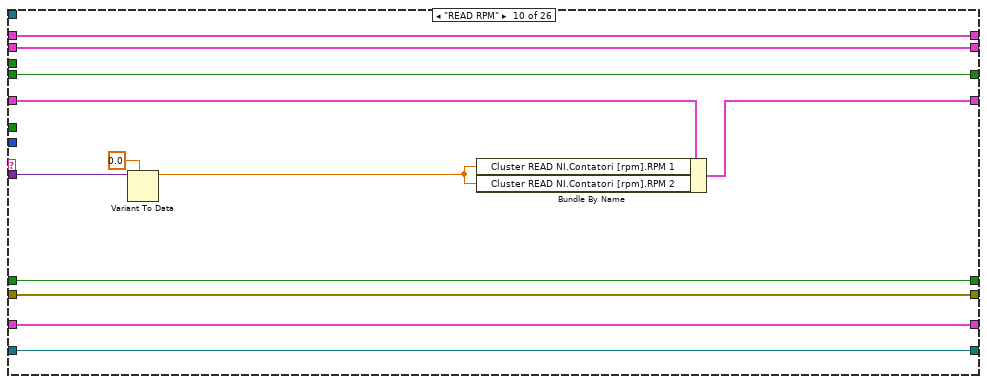
[diagram p14: hidden frame]
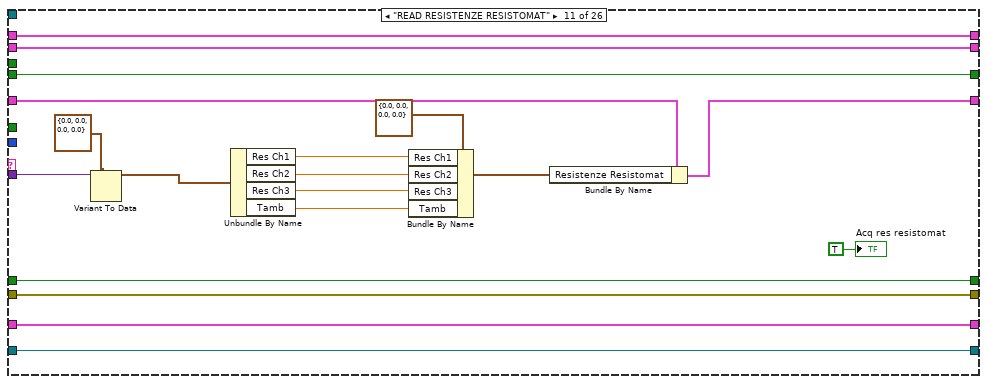
[diagram p15: hidden frame]
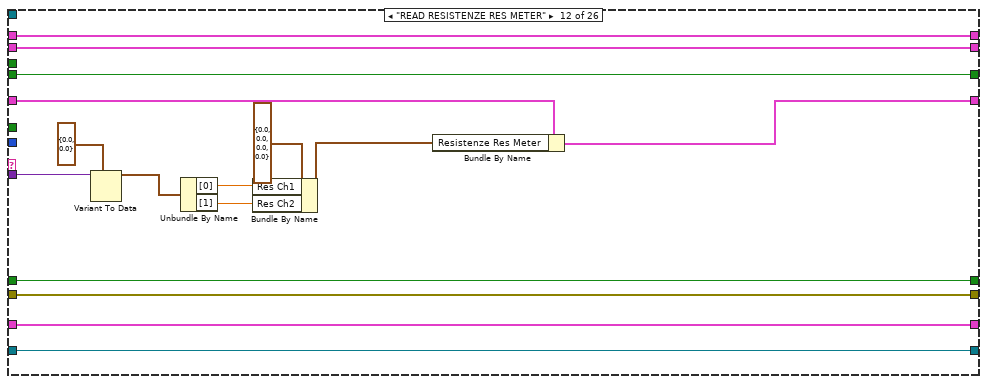
[diagram p16: hidden frame]
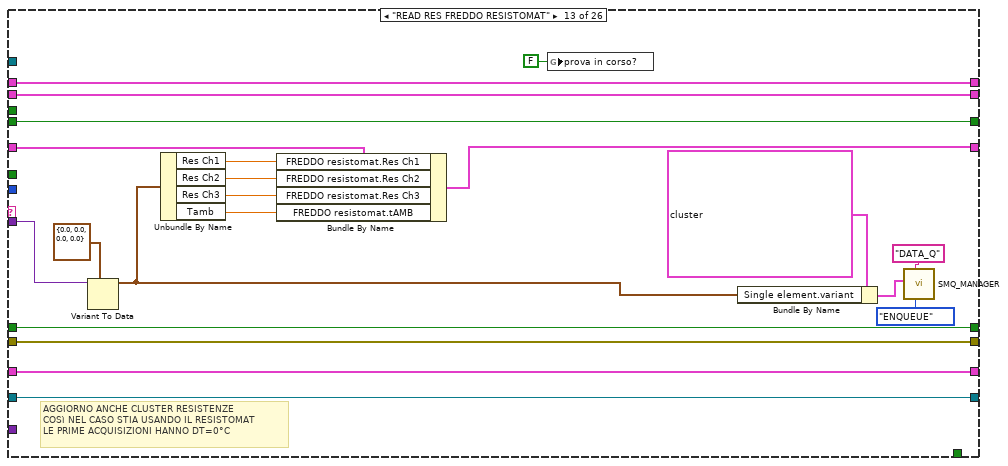
[diagram p17: hidden frame]
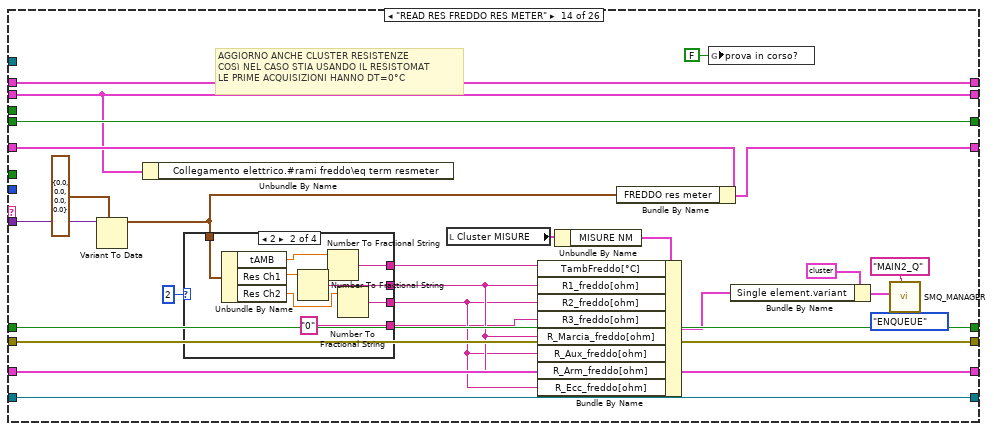
[diagram p18: hidden frame]
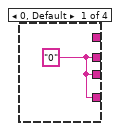
[diagram p19: hidden frame]
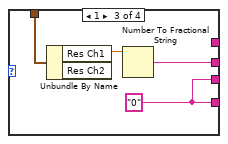
[diagram p20: hidden frame]
diagram:
  (unwired) path "C:/Lavori_in_corso_Tecnico4/NUOVO MOTORTEST/Codice/Variabili condivise/Libreria variabili Pedrollo.lvlib" ("Path")
  w1 = TRUE
  # "o a1 = -3,983035\no a2 = 301,797\no a3 = 522528,9\no a4 = 69,34881\no a5 = 999,974950"
  # "densità=a5*(1-((T_liq+a1)^2*(T_liq+a2))/(a3*(T_liq+a4)))"
  # "P2=(2*pigreco*n/60)*(Tq)"
  # "P3=densità*Q*g*H"
  # "Hdinamica=(v2^2-v1^2)/(2*g)"
  # "Hvconi=Hv1+Hv2"
  # "Formula calcolo per perdita cono divergente (cono 2 in mandata, per angoli minori di 45°)\n\nK2=2,6*sin(teta/2)*(1-(d1^2/d2^2))^2\nteta=2*arctan(((d2-d1)/2)/lungh)\nv=Q(m3/sec)/sez(m2)\nsez=(d1/1000)^2*pigreco/4\nhv2=K2*(v^2/(2*g))\n\nK2=coefficente di perdita cono divergente\nteta=angolo apertura cono\nd1=diametro minore\nd2=diametro maggiore\nv=velocità caclolata su d1 \nlungh=lunghezza cono"
  # "Formula calcolo per perdita cono convergente (cono 1 in aspirazione, per angoli minori di 45°)\n\nK1=0,8*sin(teta/2)*(1-(d1^2/d2^2))\nteta=2*arctan(((d2-d1)/2)/lungh)\nv=Q(m3/sec)/sez(m2)\nsez=(d1/1000)^2*pigreco/4\nhv1=K1*(v^2/(2*g))\n\nK1=coefficente di perdita cono convergente\nteta=angolo apertura cono\nd1=diametro minore\nd2=diametro maggiore\nv=velocità caclolata su d1\nlungh=lunghezza cono\ng=9,80665"
  # "Htot=dislivello+Hdinamica+Hvconi+Hvtronchetti-(H1*100000/(g*densità))+((H2+H1)*100000/(g*densità)) 9,80665"
  # "MISURE UL\nNumero::Riporta\nMisura::Riporta\nAcquisizione::NO\nData::Riporta\ntempo camp. [s]::Riporta\nQ [m3/h]::Analisi\nQ s::Analisi\nQ eR::Analisi\nQ [GPM]::Media\nH1 [bar]::Analisi\nH1 s::Analisi\nH1 eR::Analisi\nDislivello [m]::Media\nHdinamica [m]::Media\nH2 [bar]::Analisi\nH2 s::Analisi\nH2 eR::Analisi\nHtot [m]::Analisi\nHtot e::Analisi\nHtot [PSI]::Analisi\nP3 (Phyd) [W]::Media\nn [rpm]::Analisi\nn s::Analisi\nn eR::Analisi\nTq [Nm]::Analisi\nTq s::Analisi\nTq eR::Analisi\nP2 [W]::Media\neta pompa [%]::Media\nT [°C]::Analisi\nT s::Analisi\nT eR::Analisi\nDensità liquido [kg/m3]::Media\nP barometrica [mbar]::Media\nNote::Riporta\nNote::Riporta\nNote::Riporta\nNote::Riporta"
  n1 = local write "SEND_Main2?"(w1) -> ()
  n2 = Obtain Queue(name (unnamed)="Queue Name", element data type=cluster{"String":string, "variant":variant} {"String"="", "variant"=variant} ("element")) -> (queue out=w9:refnum<queue>, error out=w8:errorcluster)  [unwired: 3 in, 1 out]
  n3 = Get Queue Status(queue=w9, error in (no error)=w8) -> (queue out=w13:refnum<queue>, error out=w12:errorcluster, # elements in queue=w11:i32)  [unwired: 1 in, 5 out]
  n4 = Not Equal?(x="variant", y=variant) -> (x != y?=w22:bool)
  n5 = Equal To 0?(x=w11) -> (x = 0?=w10:bool)
  n6 = case shown="True" w22 {
    tunnel: [w30 w33] -> w20
    tunnel: "variant" -> [w30 w31]
    frame False {
    }
    frame True {
      n7 = Variant To Data(type=variant, Variant=w31) -> (data=w33:variant)  [unwired: 1 in, 1 out]
    }
  }
  n8 = case shown="True" w10 {
    tunnel: w13 -> [w34 w40]
    tunnel: w12 -> [w35 w39]
    tunnel: [w34 w38] -> w7
    tunnel: [w35 w37] -> w6
    frame False {
    }
    frame True {
      n9 = Enqueue Element(queue=w40, element=cluster{"String":string, "variant":variant} {"String"="INITIALIZE", "variant"=variant}, error in (no error)=w39) -> (queue out=w38:refnum<queue>, error out=w37:errorcluster)  [unwired: 1 in, 1 out]
    }
  }
  n10 = flat-sequence {
    tunnel: [w41] -> w14
    frame #0 {
      w41 = FALSE ("Stop")
      "Stopped" <- w41
    }
  }
  n11 = while {
    shift-right: [w78] -> w16
    shift-left: _ -> [w77]
    shift-right: [w74] -> w28
    shift-left: "error in (no error)" -> [w76]
    tunnel: w20 -> [w73]
    tunnel: w7 -> [w71]
    tunnel: w6 -> [w72]
    tunnel: [w68] -> w25
    shift-right: [w67] -> _
    shift-left: FALSE -> [w66]
    shift-right: [w60] -> _
    shift-left: _ -> [w59]
    shift-right: [w58] -> _
    shift-left: _ -> [w57]
    shift-right: [w52] -> _
    shift-left: _ -> [w51]
    shift-right: [w50] -> _
    shift-left: _ -> [w49]
    shift-right: [w48] -> _
    shift-left: _ -> [w47]
    tunnel: "simulazione" -> [w46]
    tunnel: "BANCO" -> [w43]
    tunnel: "Torsiometro" -> [w42]
    i -> [w53]
    stop <- w68 stop-if-true
    # "PROCESSI CONTINUI"
    n12 = feedback #1() -> (w55:u32)  [unwired: 1 in]
    n13 = call <userlib>:"loop timer.vi"("millisecond timer IN"=w55) -> ("millisecond timer OUT"=w56:u32, "LOOP TIME (ms)"=→"LOOP TIME (ms)":u32)  [unwired: 9 in]
    n14 = feedback-in #1(w56) -> ()
    n15 = Dequeue Element(queue=w71, error in (no error)=w72) -> (queue out=w45:refnum<queue>, element=w70:cluster{"String":string, "variant":variant}, error out=w63:errorcluster)  [unwired: 1 in, 1 out]
    n16 = Get Queue Status(queue=w45) -> (# elements in queue=→"Elements in queue":i32)  [unwired: 2 in, 7 out]
    n17 = Greater Than 0?(x=w53) -> ()  [unwired: 1 out]
    n18 = Unbundle(w70) -> ("String"=w64:string, "variant"=w69:variant)
    n19 = global read "Globals.vi" "NM?"() -> (w61:bool)
    n20 = call <userlib>:"SMQ_HistoryManager.vi"("Caller VI"="DATA", "State"=w64, "error in (no error)"=w63, "Function"=enum16{"INITIALIZE", "REC", "STOP"}."REC") -> ()  [unwired: 14 in, 2 out]
    n21 = case shown="\"AGGIORNA INFO\"" w64 {
      tunnel: [_ _ _ _ _ _ _ _ _ _ _ _ _ _ _ _ _ _ _ _ _ _ _ _ _ TRUE] -> w75
      tunnel: [w88 w162 w184 w203 w215 w227 w245 w257 w269 w281 w300 w316 w337 w362 w395 w411 w429 w441 w452 w462 w472 w523 w534 w558 w585 w594] -> w78
      tunnel: w77 -> [_ w162 w184 w203 w215 w227 w245 w257 w269 w281 w300 w316 w337 w362 w395 w411 w429 w441 w452 w462 w472 w523 w534 w558 w585 w594]
      tunnel: w76 -> [w87 w157 w183 w202 w214 w226 w244 w256 w268 w280 w299 w315 w336 w361 w394 w410 w428 w440 w451 w461 w475 w522 w533 w557 w586 w593]
      tunnel: [w87 w156 w183 w202 w214 w226 w244 w256 w268 w280 w299 w315 w336 w361 w394 w410 w428 w440 w451 w461 w475 w522 w533 w553 w586 w593] -> w74
      tunnel: w73 -> [_ _ _ _ _ _ _ _ _ _ _ _ _ _ _ _ _ _ _ _ _ _ _ _ _ _]
      tunnel: w69 -> [_ w159 w181 w196 w208 w220 w242 w250 w262 w272 w297 w313 w328 w354 w387 w402 w419 w437 w445 w457 w466 w521 w532 _ _ _]
      tunnel: [w86 w161 w182 w201 w213 w225 w243 w255 w267 w279 w298 w314 w335 w360 w393 w409 w427 w439 w450 w460 w474 w519 w524 w551 w584 w592] -> w67
      tunnel: w66 -> [w86 w161 w182 w201 w213 w225 w243 w255 w267 w279 w298 w314 w335 w360 w393 w409 w427 w439 w450 w460 w474 _ w524 w551 w584 w592]
      tunnel: w61 -> [w85 _ _ _ _ _ _ _ _ _ _ _ _ _ _ _ _ w436 _ _ _ _ _ _ _ _]
      tunnel: [w84 w160 w177 w193 w206 w218 w240 w246 w258 w273 w295 w311 w332 w355 w388 w400 w418 w438 w449 w459 w470 w518 w529 w545 w583 w591] -> w60
      tunnel: w59 -> [_ w160 w178 w194 w205 w217 w235 w247 w259 w274 w296 w312 w329 w356 w389 w401 w415 w438 w449 w459 w470 w518 w529 w546 w583 w591]
      tunnel: [w83 w118 w175 w200 w212 w224 w236 w254 w266 w278 w294 w310 w330 w344 w384 w408 w414 w434 w443 w458 w473 w517 w528 w535 w582 w590] -> w58
      tunnel: w57 -> [_ w158 w175 w200 w212 w224 w236 w254 w266 w278 w294 w310 w330 w344 w384 w408 w414 w434 w443 w458 w473 w517 w528 w535 w582 w590]
      tunnel: [w82 w153 w173 w199 w211 w223 w239 w253 w265 w277 w293 w309 w334 w359 w392 w407 w426 w433 w448 w456 w471 w516 w527 w549 w581 w589] -> w52
      tunnel: w51 -> [w82 w153 w173 w199 w211 w223 w239 w253 w265 w277 w293 w309 w334 w359 w392 w407 w426 w433 w448 _ w471 w516 w527 w549 w581 w589]
      tunnel: [w81 w152 w179 w198 w210 w222 w238 w252 w264 w276 w292 w308 w333 w358 w391 w406 w425 w432 w447 w455 w469 w515 w526 w550 w580 w588] -> w50
      tunnel: w49 -> [w81 w152 w179 w198 w210 w222 w238 w252 w264 w276 w292 w308 w333 w358 w391 w406 w425 w432 w447 w455 _ w515 w526 w550 w580 w588]
      tunnel: [w80 w151 w176 w197 w209 w221 w237 w251 w263 w275 w291 w307 w331 w357 w390 w405 w413 w431 w446 w454 w467 w514 w525 w536 w579 w587] -> w48
      tunnel: w47 -> [_ w151 w176 w197 w209 w221 w237 w251 w263 w275 w291 w307 w331 w357 w390 w405 w413 w431 w446 w454 w468 w514 w525 w536 w579 w587]
      tunnel: w46 -> [_ _ _ _ _ _ _ _ _ _ _ _ _ _ _ _ _ _ _ _ _ _ _ w541 _ _]
      tunnel: w43 -> [w79 w115 _ _ _ _ _ _ _ _ _ _ _ _ _ _ _ _ _ _ _ _ _ w542 _ _]
      tunnel: w42 -> [_ _ _ _ _ _ _ _ _ _ _ _ _ _ _ _ _ _ _ _ _ _ _ w538 _ _]
      frame "INITIALIZE", Default {
        n22 = stacked-sequence {
          tunnel: [w114] -> w88
          tunnel: w85 -> [_]
          tunnel: [w111] -> w84
          tunnel: [T31 {"Scelta wattmetro"={"Wattmetro"=enum."No Selection"}, "SET RPM"=0.0, "SET TEMP"=0.0, "Array banchi"=[{"Nome"="Elettropompa", "Tors. scala1"=0, "Tors. scala2"=0, "rpm"=0, "TAMB"=0, "Indici Temperature"=[0, 1], "Indice freno"=1, "alimentatore trifase"=0, "alimentatore monofase"=0, "alimentatore dc arm"=0, "alimentatore dc ecc"=0, "alimentatore dc mp"=0}, {"Nome"="Sommersa", "Tors. scala1"=0, "Tors. scala2"=0, "rpm"=0, "TAMB"=1, "Indici Temperature"=[0, 1], "Indice freno"=0, "alimentatore trifase"=0, "alimentatore monofase"=0, "alimentatore dc arm"=0, "alimentatore dc ecc"=0, "alimentatore dc mp"=0}], "Array valvole linee avvio/fermata"=[], "banco selezionato"=0, "Nomi valvole prop sistema"=[], "canale-- sensore"=[], "Attriti B1"=[], "Attriti B2"=[], "Collegamento elettrico"={"ALIMENTAZIONE ELETTRICA"=enum."AC TRIFASE", "ID"=0, "#rami freddo\\eq term resmeter"=0, "#rami riscaldamento resmeter"=0, "#rami freddo\\eq term resistomat"=0, "#rami riscaldamento resistomat"=0, "CALCOLI"=enum."AC TRIFASE"}, "lingua"=0, "Costanti collaudo"={"P [bar]"=0.0, "T amb. [°C]"=0.0, "Umidità [%]"=0.0, "T acqua [°C] 2"=0.0}, "OPZIONI MISURE RES"={"MISURA A FREDDO"=enum."RESISTOMAT", "MISURA EQ. TERMICO"=enum."RESISTOMAT", "MISURA DT PROVA IN CORSO"=enum."RESISTOMAT - CON FERMATE", "MISURE PRIMA E DOPO"=enum."RESISTOMAT", "STRUMENTI PRESENTI"=enum."NESSUNO"}, "Dati targa motore"={"Vnom"=0.0, "Fnom"=0.0, "Inom"=0.0, "Cnom"=0.0, "Npoli"=0.0, "Scorta 1"=0.0, "Scorta 2"=0.0, "Scorta 3"=0.0}} ("Cluster INFO 2")] -> w83
          tunnel: [cluster{dbl[], dbl[]} {[], []} ("output cluster")] -> w80
          tunnel: w79 -> [w93]
          frame #0 {
            w111 = T9 {"Cluster READ NI"={"AI (0-10V)"={"AI 0"=0.0, "AI 1"=0.0, "AI 2"=0.0, "AI 3"=0.0, "AI 4"=0.0, "AI 5"=0.0, "AI 6"=0.0, "AI 7"=0.0, "AI 8"=0.0, "AI 9"=0.0, "AI 10"=0.0, "AI 11"=0.0, "AI 12"=0.0, "AI 13"=0.0, "AI 14"=0.0, "AI 15"=0.0, "AI 16"=0.0, "AI 17"=0.0, "AI 18"=0.0, "AI 19"=0.0, "AI 20"=0.0, "AI 21"=0.0, "AI 22"=0.0, "AI 23"=0.0, "AI 24"=0.0, "AI 25"=0.0, "AI 26"=0.0, "AI 27"=0.0, "AI 28"=0.0, "AI 29"=0.0, "AI 30"=0.0, "AI 31"=0.0}, "StatoAO_Cdaq[0-10V]"={"AO 1"=0.0, "AO 2"=0.0, "AO 3"=0.0, "AO 4"=0.0}, "Contatori [rpm]"={"RPM 1"=0.0, "RPM 2"=0.0}, "StatoAO_Cdaq [4-20mA]"={"Cdaq_AO [0-10V] 0 for Torque"=0.0, "Cdaq_AO [0-10V] 1"=0.0, "Cdaq_AO [0-10V] 2"=0.0, "Cdaq_AO [0-10V] 3"=0.0}, "StatoDO_Cdaq"={"Scorta 0"=FALSE, "Scorta 1"=FALSE, "Scorta 2"=FALSE, "Scorta 3"=FALSE, "Scorta 4"=FALSE, "Scorta 5"=FALSE, "Scorta 6"=FALSE, "Scorta 7"=FALSE, "Scorta 8"=FALSE, "Scorta 9"=FALSE, "Scorta 10"=FALSE, "Scorta 11"=FALSE, "Scorta 12"=FALSE, "Scorta 13"=FALSE, "Scorta 14"=FALSE, "Scorta 15"=FALSE, "Scorta 16"=FALSE, "Scorta 17"=FALSE, "Scorta 18"=FALSE, "Scorta 19"=FALSE, "Scorta 20"=FALSE, "Scorta 21"=FALSE, "Scorta 22"=FALSE, "Scorta 23"=FALSE, "Scorta 24"=FALSE, "Scorta 25"=FALSE, "Scorta 26"=FALSE, "Scorta 27"=FALSE, "Scorta 28"=FALSE, "Scorta 29"=FALSE, "Scorta 30"=FALSE, "Scorta 31"=FALSE}, "DI"={"Scorta 0"=FALSE, "Scorta 1"=FALSE, "Scorta 2"=FALSE, "Scorta 3"=FALSE, "Scorta 4"=FALSE, "Scorta 5"=FALSE, "Scorta 6"=FALSE, "Scorta 7"=FALSE, "Scorta 8"=FALSE, "Scorta 9"=FALSE, "Scorta 10"=FALSE, "Scorta 11"=FALSE, "Scorta 12"=FALSE, "Scorta 13"=FALSE, "Scorta 14"=FALSE, "Scorta 15"=FALSE, "Scorta 16"=FALSE, "Scorta 17"=FALSE, "Scorta 18"=FALSE, "Scorta 19"=FALSE, "Scorta 20"=FALSE, "Scorta 21"=FALSE, "Scorta 22"=FALSE, "Scorta 23"=FALSE, "Scorta 24"=FALSE, "Scorta 25"=FALSE, "Scorta 26"=FALSE, "Scorta 27"=FALSE, "Scorta 28"=FALSE, "Scorta 29"=FALSE, "Scorta 30"=FALSE, "Scorta 31"=FALSE}, "AI (4-20mA)"={"AI 0"=0.0, "AI 1"=0.0, "AI 2"=0.0, "AI 3"=0.0, "AI 4"=0.0, "AI 5"=0.0, "AI 6"=0.0, "AI 7"=0.0, "AI 8"=0.0, "AI 9"=0.0, "AI 10"=0.0, "AI 11"=0.0, "AI 12"=0.0, "AI 13"=0.0, "AI 14"=0.0, "AI 15"=0.0}, "TC [°C]"={"tc 1"=0.0, "tc 2"=0.0, "tc 3"=0.0, "tc 4"=0.0}, "NI Read Values"={"RPM"=0.0, "Frequency"=0.0, "Mod 1"={"Torsiometro 1"=0.0, "Torsiometro 2"=0.0, "Strin Gauge 1"=0.0, "Strin Gauge 2"=0.0}, "Mod 2"={"Termocoppia 1"=0.0, "Termocoppia 2"=0.0, "Termocoppia 3"=0.0, "Termocoppia 4"=0.0}, "Mod 3"={"PT 100 1"=0.0, "PT 100 2"=0.0, "PT 100 3"=0.0, "PT 100 4"=0.0}}}, "MISURE WT"={"URMS 1"=0.0, "IRMS 1"=0.0, "P 1"=0.0, "S 1"=0.0, "Q 1"=0.0, "LAMBDA 1"=0.0, "PHI 1"=0.0, "F U 1"=0.0, "F I 1"=0.0, "NONE 1"=0.0, "URMS 2"=0.0, "IRMS 2"=0.0, "P 2"=0.0, "S 2"=0.0, "Q 2"=0.0, "LAMBDA 2"=0.0, "PHI 2"=0.0, "F U 2"=0.0, "F I 2"=0.0, "NONE 2"=0.0, "URMS 3"=0.0, "IRMS 3"=0.0, "P 3"=0.0, "S 3"=0.0, "Q 3"=0.0, "LAMBDA 3"=0.0, "PHI 3"=0.0, "F U 3"=0.0, "F I 3"=0.0, "NONE 3"=0.0, "URMS SIGMA"=0.0, "IRMS SIGMA"=0.0, "P SIGMA"=0.0, "S SIGMA"=0.0, "Q SIGMA"=0.0, "LAMBDA SIGMA"=0.0, "PHI SIGMA"=0.0, "F U SIGMA"=0.0, "F I SIGMA"=0.0, "NONE 4"=0.0}, "Resistenze Resistomat"={"Res Ch1"=0.0, "Res Ch2"=0.0, "Res Ch3"=0.0, "Tamb"=0.0}, "INTERFACCIA"={"AI"={"Portate"=[], "Pressioni"=[], "Coppie[Nm]"=[], "Valvole prop %"=[], "RPM"=[], "Livelli"=[], "Temperature"=[], "Riferimenti %"=[], "TENSIONI"=[], "CORRENTI"=[]}, "DI (logici)"={"Start da pulsantiera"=FALSE, "Stop da pulsantiera"=FALSE, "Reset da pulsantiera"=FALSE, "Sistema OK"=FALSE, "Collaudo abilitato"=FALSE, "Potenza trifase abilitata"=FALSE, "Potenza monofase abilitata"=FALSE, "Potenza DC abilitata"=FALSE, "Potenza DC ECC abilitata"=FALSE, "Start alimentazione AC"=FALSE, "Start alimentazione DC"=FALSE, "Start DC eccitazione"=FALSE, "Teleruttore WT abilitato"=FALSE, "Teleruttore Resistomat abilitato"=FALSE, "Teleruttore corto fasi"=FALSE, "Ramo 1 resistomat"=FALSE, "Ramo 2 resistomat"=FALSE, "Ramo 3 resistomat"=FALSE, "B1 Scelta linea elettrica 1"=FALSE, "B1 Scelta linea elettrica 2"=FALSE, "B1 Scelta linea elettrica 3"=FALSE, "B1 Scelta linea elettrica 4"=FALSE, "B1 Scelta linea elettrica 5"=FALSE, "B2 Scelta linea elettrica 1"=FALSE, "B2 Scelta linea elettrica 2"=FALSE, "B2 Scelta linea elettrica 3"=FALSE, "B2 Scelta linea elettrica 4"=FALSE, "B2 Scelta linea elettrica 5"=FALSE, "Rotore bloccato 1"=FALSE, "Rotore bloccato 2"=FALSE, "FRENO 1 abilitato"=FALSE, "FRENO 1 run"=FALSE, "FRENO 1 senso rotaz"=FALSE, "FRENO 1 ctrl velocità"=FALSE, "FRENO 2 abilitato"=FALSE, "FRENO 2 run"=FALSE, "FRENO 2 senso rotaz"=FALSE, "FRENO 2 ctrl velocità"=FALSE, "ALIM 1 abilitato"=FALSE, "ALIM 1 run"=FALSE, "ALIM 2 abilitato"=FALSE, "ALIM 2 run"=FALSE, "ALIM 3 abilitato"=FALSE, "ALIM 3 run"=FALSE, "FRENO 1 ctrl coppia"=FALSE, "FRENO 2 ctrl coppia"=FALSE, "FRENO 3 ctrl coppia"=FALSE, "DI (logici) aggiuntivi impianto"={"Solo freno abilitato"=FALSE, "Carico resistivo abilitato"=FALSE, "AFE+freno abilitato"=FALSE, "Protezioni chiuse"=FALSE, "Start potenza AFE"=FALSE, "AFE in marcia"=FALSE}, "Misura corrente diretta WT"=FALSE, "Misura corrente sens ext"=FALSE, "Sens ext abilitati"=FALSE}, "AO non scalati"={"FRENO1 rif vel"=0.0, "FRENO1 rif Coppia"=0.0, "FRENO2 rif vel"=0.0, "FRENO2 rif Coppia"=0.0, "ALIM1 rif V"=0.0, "ALIM1 rif F"=0.0, "ALIM2 rif V"=0.0, "ALIM2 rif F"=0.0, "ALIM3 rif V"=0.0, "ALIM3 rif F"=0.0, "Fnom keb"=0.0, "Rpm nom keb"=0.0, "Pnom keb"=0.0, "Inom keb"=0.0, "Vnom keb"=0.0, "Rpm max keb"=0.0, "Tempo rampa keb"=0.0, "Tipo Mot keb"=0.0, "FRENO  rif Coppia "=0.0, "FRENO  rif  Corrente"=0.0}, "AO scalati"={"FRENO1 rif vel"=0.0, "FRENO1 rif Coppia"=0.0, "FRENO2 rif vel"=0.0, "FRENO2 rif Coppia"=0.0, "ALIM1 rif V"=0.0, "ALIM1 rif F"=0.0, "ALIM2 rif V"=0.0, "ALIM2 rif F"=0.0, "ALIM3 rif V"=0.0, "ALIM3 rif F"=0.0, "Fnom keb"=0.0, "Rpm nom keb"=0.0, "Pnom keb"=0.0, "Inom keb"=0.0, "Vnom keb"=0.0, "Rpm max keb"=0.0, "Tempo rampa keb"=0.0, "Tipo Mot keb"=0.0, "FRENO  rif Coppia "=0.0, "FRENO  rif  Corrente"=0.0}, "DO (logici)"={"Scelta banco 1"=FALSE, "Scelta banco 2"=FALSE, "Scelta banco 3"=FALSE, "FRENO 1 abilita"=FALSE, "FRENO 1 start"=FALSE, "FRENO 1 senso rotaz"=FALSE, "FRENO 1 ctrl velocità"=FALSE, "FRENO 2 abilita"=FALSE, "FRENO 2 start"=FALSE, "FRENO 2 senso rotaz"=FALSE, "FRENO 2 ctrl velocità"=FALSE, "ALIM 1 abilita"=FALSE, "ALIM 1 start"=FALSE, "ALIM 2 abilita"=FALSE, "ALIM 2 start"=FALSE, "ALIM 3 abilita"=FALSE, "ALIM 3 start"=FALSE, "Abilita linea trifase"=FALSE, "Abilita linea monofase"=FALSE, "Abilita linea dc"=FALSE, "Abilita linea dc eccit"=FALSE, "B1 Linea elettrica 1"=FALSE, "B1 Linea elettrica 2"=FALSE, "B1 Linea elettrica 3"=FALSE, "B1 Linea elettrica 4"=FALSE, "B1 Linea elettrica 5"=FALSE, "B2 Linea elettrica 1"=FALSE, "B2 Linea elettrica 2"=FALSE, "B2 Linea elettrica 3"=FALSE, "B2 Linea elettrica 4"=FALSE, "B2 Linea elettrica 5"=FALSE, "Start potenza AC"=FALSE, "Stop pontenza AC"=FALSE, "Start potenza DC"=FALSE, "Stop potenza DC"=FALSE, "Start potenza eccitaz"=FALSE, "Stop potenza eccitaz"=FALSE, "Reset allarmi"=FALSE, "watchdog"=FALSE, "Scala torsiometro B1"=FALSE, "Controllo torsiom B1"=FALSE, "Scala torsiometro B2"=FALSE, "Controllo torsiom B2"=FALSE, "Teleruttore WT abilita"=FALSE, "Teleruttore Resistomat abilita"=FALSE, "Teleruttore corto fasi"=FALSE, "Ramo 1 resistomat"=FALSE, "Ramo 2 resistomat"=FALSE, "Ramo 3 resistomat"=FALSE, "Collaudo in corso"=FALSE, "Allarme presente"=FALSE, "Enable Res Meter"=FALSE, "Bypass Res Meter"=FALSE, "2nd canale Res Meter"=FALSE, "Scala 200/2000 res meter"=FALSE, "Taratura res meter"=FALSE, "FRENO 1 ctrl coppia"=FALSE, "FRENO 2 ctrl coppia"=FALSE, "FRENO 3 ctrl coppia"=FALSE, "Aggiuntivi impianto"={"Senso rotazione alim 1"=FALSE, "Senso rotazione alim 2"=FALSE}, "ALIM 1 stop"=FALSE, "ALIM 2 stop"=FALSE, "ALIM 3 stop"=FALSE, "FRENO 1 stop"=FALSE, "FRENO 2 stop"=FALSE, "FRENO 3 stop"=FALSE, "B1 configurazione freno B"=FALSE, "B2 configurazione freno B"=FALSE, "Abilita scrittura KEB"=FALSE, "Bench Selection (0-B1,1-B2)"=FALSE, "Select current mode"=FALSE, "Select torque mode"=FALSE, "Select speed mode"=FALSE, "Start"=FALSE, "Stop"=FALSE, "Block"=FALSE, "Enable Force mode"=FALSE, "Abilita linea 125 A"=FALSE, "Abilita linea 63 A"=FALSE, "Abilita linea 16 A"=FALSE, "Aum Tensione Variac"=FALSE, "Dim Tesnione Variac"=FALSE, "Abilita ellectro stractura"=FALSE, "Risprinito Emergence"=FALSE, "Abilita collaudo"=FALSE, "Disabilita collaudo"=FALSE, "External Alaram"=FALSE, "Enable external program"=FALSE, "Reset"=FALSE, "Abilita Ingresso Variac"=FALSE, "Abilita Ventilatore Variac"=FALSE, "Abilita Uscita Variac "=FALSE}}, "FREDDO resistomat"={"Res Ch1"=0.0, "Res Ch2"=0.0, "tAMB"=0.0, "Res Ch3"=0.0}, "STATO PLC 1"={"USCITE PLC"={"AO (real) 2"={"SCORTA 1"=0.0, "SCORTA 2"=0.0, "SCORTA 3"=0.0, "SCORTA 4"=0.0, "SCORTA 5"=0.0, "SCORTA 6"=0.0, "SCORTA 7"=0.0, "SCORTA 8"=0.0}, "statoAO_PLC out"={"Rif Lim coppia freno [%]"=nan, "Rif rpm freno [%]"=nan, "Rif coppia freno [%]"=0.0, "Rif V alimentatore [%]"=0.0, "Rif F alimentatore [%]"=0.0}, "DO (bit)"={"Scelta banco 1"=FALSE, "Set dati motore freno 2"=FALSE, "Diretto inverter"=FALSE, "Filtro LC"=FALSE, "Marcia ALIM (1s)"=FALSE, "Marcia FRENO (1s)"=FALSE, "Stop AFE (1s)"=FALSE, "Stop freno (1s)"=FALSE, "Reset allarmi"=FALSE, "Watchdog"=FALSE, "Senso rotazione"=FALSE, "Abilita collaudo (1s)"=FALSE, "Disabilita collaudo (1s)"=FALSE, "Abilitazione ALIM"=FALSE, "Abilitazione FRENO"=FALSE, "Teleruttore WT"=FALSE, "Senso rot motore prova"=FALSE, "Scorta 7"=FALSE, "Scorta 8"=FALSE, "Scorta 9"=FALSE, "Scorta 10"=FALSE, "Scorta 11"=FALSE, "Scorta 12"=FALSE, "Scorta 13"=FALSE}}, "Stato DI_PLC"={"Sistema OK"=FALSE, "Rotore bloccato"=FALSE, "Scorta 1"=FALSE, "Prova diretto inverter"=FALSE, "Prova con filtro LC"=FALSE, "Teleruttore WT abilitato"=FALSE, "Alim sinus penta abilitato"=FALSE, "Alim sinus penta in marcia"=FALSE, "Freno abilitato"=FALSE, "Freno in marcia"=FALSE, "Senso rotazione freno"=FALSE, "Potenza abilitata"=FALSE, "Scorta 3"=FALSE, "Scorta 4"=FALSE, "scorta 5"=FALSE, "scorta 6"=FALSE}, "AI plc"={"Allarmi 1"=0.0, "Allarmi 2"=0.0, "Scorta 1"=0.0, "Scorta 2"=0.0, "RPM mot prova"=0.0, "I mot prova"=0.0, "RPM freno"=0.0, "I freno"=0.0, "Scorta 3"=0.0, "Scorta 4"=0.0}}, "Res Ch2"=0.0, "Res Ch2 2"=0.0, "FREDDO res meter"={"Res Ch1"=0.0, "Res Ch2"=0.0, "tAMB"=0.0, "Res Ch3"=0.0}, "Resistenze Res Meter"={"Res Ch1"=0.0, "Res Ch2"=0.0, "Res Ch3"=0.0, "Tamb"=0.0}, "READ SINUS PENTA"={"Menù Misure motore (M000-M030)"={"Rif vel a regime (int)"=0, "Rif vel a regime (dec)"=0, "Rif vel dopo rampe (int)"=0, "Rif vel dopo rampe (dec)"=0, "RPM motore (int)"=0, "RPM motore (dec)"=0, "FREQout inverter"=0, "Rif coppia a regime(Nm)"=0, "Richiesta di coppia (Nm)"=0, "Coppia generata dal motore(Nm)"=0, "Rif coppia a regime(%)"=0, "Richiesta di coppia (%)"=0, "Coppia generata dal motore(%)"=0, "Coppia max richiesta prima delle rampe(Nm)"=0, "Coppia max richiesta dopo le rampe(Nm)"=0, "Limite di velocità prima delle rampe"=0, "Limite di velocità dopo le rampe"=0, "Coppia max richiesta prima delle rampe(%)"=0, "Coppia max richiesta dopo le rampe(%)"=0, "Rif di flusso"=0, "Corrente di uscita"=0, "Capacità termica del motore"=0, "Tensione di uscita"=0, "Potenza di uscita"=0, "Energia consumata (LSword)"=0, "Energia consumata (MSword)"=0, "Tensione bus DC"=0, "Tensione di rete"=0}, "Menù regolatore PID (M018-M024)"={"Rif PID a regime(%)"=0, "Rif pid dopo rampe(%)"=0, "Retroazione del pid(%)"=0, "Errore del pid(%)"=0, "uscita del pid(%)"=0, "Rif del pid dopo le rampe"=0, "Retroazione del pid"=0}, "Menù ingressi digitali (M031-M036)"={"Ingressi digitali ritardati"=0, "Ingressi digitali istantanei"=0, "Moresettiera comando loc"=0, "Morsett comando da seriale"=0, "Morsett comando bus di campo"=0, "Ing dig ausiliari da morsettiera"=0, "Ing dig ausiliari da seriale"=0}, "Menù riferimenti (M037-M051)"={"Rif analog est REF"=0, "Rif analog est AIN1"=0, "Rif analog est AIN2"=0, "Rif analog est XAIN4"=0, "Rif analog est XAIN5"=0, "Rif velocità da seriale(int)"=0, "Rif velocità bus di campo(int)"=0, "Rif coppia da seriale"=0, "Rif coppia bus di campo"=0, "Rif del PID da seriale"=0, "Rif del PID da bus di campo"=0, "Retroazione del PID da seriale"=0, "Retroazione del PIDda bus di campo"=0, "Rif da encoder"=0, "Rif in frequenza"=0, "Rif velocità da seriale(dec)"=0, "Rif velocità bus di campo(dec)"=0}, "Menù rampe (P009-P033)"={"Tempo di dec rampa di vel 1"=0, "Tempo di acc rampa di vel 2"=0, "Tempo di dec rampa di vel 2"=0, "Tempo di acc rampa di vel 1"=0, "Unità di mis tempi rampe vel 1/2"=0, "Tempo di acc rampa di vel 3"=0, "Tempo di dec rampa di vel 3"=0, "Tempo di acc rampa di vel 4"=0, "Tempo di dec rampa di vel 4"=0, "Unità di mis tempi rampe vel 3/4"=0, "Selettore arrottondam rampe"=0, "Tempo di arrotond iniz rampa acc"=0, "Tempo di arrotond finale rampa acc"=0, "Tempo di arrotond iniz rampa dec"=0, "Tempo di rampa di salita rif coppia"=0, "Tempo di rampa di discesa rif coppia"=0, "Unità di misura rampa coppia"=0, "Tempo rampa acc marcia jog"=0, "Tempo rampa dec marcia jog"=0, "Reset acc ai cambi pendenza"=0, "rampa di acc in fire mode"=0, "rampa di dec in fire mode"=0, "Tempo di arrotond finale rampa dec"=0}, "Menù controllo motore(C008-C128)"={"Numero motori configurati"=0, "Tipo algoritmo di controllo Mot1"=0, "Tipo rif Mot1"=0, "Tensione nominale rete"=0, "Retroaz di vel da encoder Mot1"=0, "Tipo curva V/f Mot1"=0, "Rotazione delle fasi Mot1"=0, "Freq nominale del motore Mot1"=0, "RPM nominali del motore Mot1"=0, "Potenza nominale del motore Mot1"=0, "Corrente nominale del motore Mot1"=0, "Tensione nominale del motore mot1"=0, "Potenza a vuoto del motore Mot1"=0, "Corrente a vuoto del motore Mot1"=0, "Resistenza statorica del motore Mot1"=0, "Induttanza di dispersione Mot1"=0, "Induttanza mutua motore"=0, "Costante di tempo rotorica"=0, "Costante di tempo filtro pb"=0, "Velocità minima motore"=0, "Velocità massima motore"=0}, "Menù configurazione PID"={"Selezione riferimento n.1"=0, "Selezione retroazione n.1"=0, "Modalità di fuzionamento PID"=0, "Termine derivativo calcolato su err o mis"=0, "Proporz moltiplica deriv e integrale"=0, "Azione del PID"=0}, "ID"=0.0, "Menù uscite digitali"={"MDO4 Inverter pronto"=0}, "Fcarrier"={"Fcarrier Min (Hz)"=0, "Fcarrier Max (Hz)"=0}, "stato inverter M089"=0.0, "Riferimenti"={"Rif tensione"=0, "Rif velocità"=0}, "Comunicazione"=FALSE, "Modalità stop"=0.0}, "STATO PLC 2"={"USCITE PLC"={"AO (real) 2"={"SCORTA 1"=0.0, "SCORTA 2"=0.0, "SCORTA 3"=0.0, "SCORTA 4"=0.0, "SCORTA 5"=0.0, "SCORTA 6"=0.0, "SCORTA 7"=0.0, "SCORTA 8"=0.0}, "statoAO_PLC out"={"Condensatori"=0.0, "Scorta 1"=0.0, "Scorta 2"=0.0}, "DO (bit)"={"Relè misura resistomat"=FALSE, "Misura res ramo 1"=FALSE, "Misura res ramo 2"=FALSE, "Misura res ramo 3"=FALSE, "Scelta banco 2"=FALSE, "Scala Torsiometro"=FALSE, "Ctrl torsiometro"=FALSE, "Select current mode"=FALSE, "Select Torque mode"=FALSE, "Select speed mode"=FALSE, "Watchdog"=FALSE, "Scorta"=FALSE, "Scorta 2"=FALSE, "Scorta 3"=FALSE, "Scorta 4"=FALSE, "Scorta 5"=FALSE, "Bench selection"=FALSE, "External alarm"=FALSE, "Enable external program"=FALSE, "Reset allarmi"=FALSE, "Start"=FALSE, "Stop"=FALSE, "Block"=FALSE, "Scorta 6"=FALSE}}, "Stato DI_PLC"={"Sistema ok"=FALSE, "Relè Resistomat abilitato"=FALSE, "Freno abilitato"=FALSE, "Freno in marcia"=FALSE, "scorta b"=FALSE, "scorta a"=FALSE, "scorta 1"=FALSE, "scorta 2"=FALSE, "scorta 3"=FALSE, "scorta 4"=FALSE, "Scorta 5"=FALSE, "Scorta 6"=FALSE, "Scorta 7"=FALSE, "Scorta 8"=FALSE, "Scorta 9"=FALSE, "Scorta 10"=FALSE}, "AI plc"={"Allarmi 1"=0.0, "Allarmi 2"=0.0, "TC 1"=0.0, "TC 2"=0.0, "TC 3"=0.0, "TC 4"=0.0, "TC 5"=0.0, "TC 6"=0.0, "TC 7"=0.0, "TC 8"=0.0, "PT1000 1"=0.0, "PT1000 2"=0.0, "PT1000 3"=0.0, "PT1000 4"=0.0}}, "STATO PLC 3"={"USCITE PLC"={"AO (real) 2"={"SCORTA 1"=0.0, "SCORTA 2"=0.0, "SCORTA 3"=0.0, "SCORTA 4"=0.0, "SCORTA 5"=0.0, "SCORTA 6"=0.0, "SCORTA 7"=0.0, "SCORTA 8"=0.0}, "statoAO_PLC out"={"Rif velocità alimentatore"=0.0, "Scorta"=0.0, "Tipo Motore  keb"=0.0, "I nom keb"=0.0, "RPM nom keb"=0.0, "V nom keb"=0.0, "F nom keb"=0.0, "t rampa keb"=0.0}, "DO (bit)"={"Select linea Inverter"=FALSE, "Abilita sense wattmetro"=FALSE, "Bypass filtro LC"=FALSE, "Filtro LC"=FALSE, "Bypass trasformatore"=FALSE, "Trasformatore"=FALSE, "Abilita uscite variac"=FALSE, "Abilita linea 125 A"=FALSE, "Abilita linea 63 A"=FALSE, "Abilita linea 16 A"=FALSE, "Abilita Scrittura Dati Keb"=FALSE, "Abilita alimentatore"=FALSE, "Marcia alimentatore (1s)"=FALSE, "Stop alimentatore (1s)"=FALSE, "Senso rot mot prova"=FALSE, "Watchdog"=FALSE, "Aumenta tensione variac"=FALSE, "Diminuisci tensione variac "=FALSE, "Blocco elettroserrature"=FALSE, "Ripristino emergence"=FALSE, "Abilita ingresso variac"=FALSE, "Abilita ventilatore variac"=FALSE, "Reset Allarm"=FALSE, "Scorta 1"=FALSE, "Scorta 2"=FALSE, "Scorta 3"=FALSE, "Scorta 4"=FALSE, "Scorta 5"=FALSE, "Scorta 6"=FALSE, "Scorta 7"=FALSE, "Scorta 8"=FALSE, "Scorta 9"=FALSE, "Abilita collaudo"=FALSE, "Disabilita collaudo "=FALSE, "Scorta 10"=FALSE, "Scorta 11"=FALSE, "Scorta 12"=FALSE, "Scorta 13"=FALSE, "Scorta 14"=FALSE, "Scorta 15"=FALSE}}, "Stato DI_PLC"={"Sistema OK"=FALSE, "Rotore bloccato"=FALSE, "Filtro LC"=FALSE, "Bypass Filtro LC"=FALSE, "Scelta Trasformatore"=FALSE, "Scelta Bypass trasformatore"=FALSE, "Teleruttore wt abilitato"=FALSE, "Alimentatore abilitato"=FALSE, "Alimentatore in marcia"=FALSE, "Scorta 1"=FALSE, "Scorta 2"=FALSE, "Scorta 3"=FALSE, "Potenza abilitata"=FALSE, "Alimentatore in allarme"=FALSE, "Scorta 4"=FALSE, "Conferma dati KEB"=FALSE, "Scorta 5"=FALSE, "Warning Inverter Alimentatore"=FALSE, "Variac Abilitato"=FALSE, "Linea 125 A abilitata"=FALSE, "Linea 63 A abilitata"=FALSE, "Linea 16 A abilitata"=FALSE, "Scorta 6"=FALSE, "Enable force mode"=FALSE}, "AI plc"={"Allarmi 1"=0.0, "Allarmi 2"=0.0, "RPM motore prova"=0.0, "Corrente motore prova"=0.0, "RPM freno"=0.0, "Corrente freno"=0.0, "Tipo motore keb"=0.0, "I nom keb"=0.0, "RPM nom keb"=0.0, "V nom keb"=0.0, "F nom keb"=0.0, "T rampa keb"=0.0, "scorta"=0.0, "Scorta 2"=0.0}}, "DCREG"={"Parametri di misura"={"M000"=0.0, "M001"=0.0, "M002"=0.0, "M003"=0.0, "M004"=0.0, "M005"=0.0, "M006"=0.0, "M007"=0.0, "M008"=0.0, "M009"=0.0, "M010"=0.0, "M011"=0.0, "M012"=0.0, "M013"=0.0, "M014"=0.0, "M015"=0.0, "M016"=0.0, "M017"=0.0, "M018"=0.0, "M019"=0.0, "M020"=0.0, "M021"=0.0, "M022"=0.0, "M023"=0.0, "M024"=0.0, "M025"=0.0, "M026"=0.0, "M027"=0.0, "M028"=0.0, "M029"=0.0, "M030"=0.0, "M031"=0.0}, "Parametri di programmazione"={"P000"=0.0, "P001"=0.0, "P002"=0.0, "P003"=0.0, "P004"=0.0, "P005"=0.0, "P006"=0.0, "P010"=0.0, "P011"=0.0, "P012"=0.0, "P013"=0.0, "P014"=0.0, "P015"=0.0, "P016"=0.0, "P030"=0.0, "P031"=0.0, "P032"=0.0, "P033"=0.0, "P034"=0.0, "P035"=0.0, "P036"=0.0, "P037"=0.0, "P038"=0.0, "P039"=0.0, "P040"=0.0, "P050"=0.0, "P051"=0.0, "P052"=0.0, "P053"=0.0, "P054"=0.0, "P055"=0.0, "P056"=0.0, "P057"=0.0, "P058"=0.0, "P059"=0.0, "P060"=0.0, "P061"=0.0, "P062"=0.0, "P070"=0.0, "P071"=0.0, "P073"=0.0, "P074"=0.0, "P076"=0.0, "P077"=0.0, "P079"=0.0, "P080"=0.0, "P082"=0.0, "P083"=0.0, "P084"=0.0, "P085"=0.0, "P086"=0.0, "P087"=0.0, "P088"=0.0, "P100"=0.0, "P101"=0.0, "P102"=0.0, "P103"=0.0, "P104"=0.0, "P110"=0.0, "P111"=0.0, "P120"=0.0, "P121"=0.0, "P122"=0.0, "P123"=0.0, "P124"=0.0, "P125"=0.0, "P126"=0.0, "P127"=0.0, "P128"=0.0, "P129"=0.0, "P130"=0.0, "P131"=0.0, "P132"=0.0, "P133"=0.0, "P134"=0.0, "P150"=0.0, "P151"=0.0, "P152"=0.0, "P153"=0.0, "P154"=0.0, "P155"=0.0, "P156"=0.0, "P157"=0.0, "P158"=0.0, "P170"=0.0, "P171"=0.0, "P172"=0.0, "P173"=0.0, "P174"=0.0, "P175"=0.0, "P176"=0.0, "P177"=0.0, "P178"=0.0, "P179"=0.0, "P180"=0.0, "P181"=0.0, "P182"=0.0, "P183"=0.0, "P184"=0.0, "P185"=0.0, "P186"=0.0, "P187"=0.0, "P188"=0.0, "P189"=0.0, "P190"=0.0, "P191"=0.0, "P192"=0.0, "P193"=0.0, "P194"=0.0, "P195"=0.0, "P196"=0.0, "P197"=0.0, "P198"=0.0, "P199"=0.0, "P211"=0.0, "P212"=0.0, "P213"=0.0, "P214"=0.0, "P215"=0.0, "P216"=0.0, "P217"=0.0, "P221"=0.0, "P222"=0.0, "P223"=0.0, "P224"=0.0, "P230"=0.0, "P231"=0.0, "P240"=0.0, "P250"=0.0, "P251"=0.0}, "Parametri di configurazione"={"C000"=0.0, "C001"=0.0, "C002"=0.0, "C010"=0.0, "C011"=0.0, "C012"=0.0, "C014"=0.0, "C015"=0.0, "C016"=0.0, "C017"=0.0, "C018"=0.0, "C030"=0.0, "C050"=0.0, "C051"=0.0, "C052"=0.0, "C060"=0.0, "C061"=0.0, "C062"=0.0, "C063"=0.0, "C070"=0.0, "C072"=0.0, "C074"=0.0, "C090"=0.0, "C091"=0.0, "C092"=0.0, "C093"=0.0, "C094"=0.0, "C100"=0.0, "C101"=0.0, "C102"=0.0, "C103"=0.0, "C105"=0.0, "C106"=0.0, "C107"=0.0, "C108"=0.0, "C110"=0.0, "C111"=0.0, "C112"=0.0, "C120"=0.0, "C121"=0.0, "C122"=0.0, "C130"=0.0, "C131"=0.0, "C132"=0.0, "C133"=0.0, "C134"=0.0, "C135"=0.0, "C141"=0.0, "C142"=0.0, "C143"=0.0, "C150"=0.0, "C151"=0.0, "C153"=0.0, "C154"=0.0, "C155"=0.0, "C156"=0.0, "C157"=0.0, "C158"=0.0, "C159"=0.0, "C160"=0.0, "C161"=0.0, "C162"=0.0, "C163"=0.0, "C164"=0.0, "C165"=0.0, "C170"=0.0}, "Codice allarme"=0.0, "Comunicazione"=FALSE}}  # MISURE ALL
            n23 = Decrement(x=w93) -> (x-1=w104:i32)
            n24 = Decrement(x=w93) -> (x-1=w96:i32)
            n25 = Build Array("Settings\\Gestione sensori\\Assoc_Input_Sensori_B1.txt" ("name or relative path"), "Settings\\Gestione sensori\\Assoc_Input_Sensori_B2.txt" ("name or relative path")) -> (w97:string[])
            n26 = Build Array("Settings\\Gestione sensori\\measures_settings_INPUT_B1.txt" ("name or relative path"), "Settings\\Gestione sensori\\measures_settings_INPUT_B2.txt" ("name or relative path")) -> (w105:string[])
            n27 = Index Array(array=w97, index=w96) -> (element=w94:string)
            n28 = call <vilib>:"Application Directory.vi"() -> ("Application Directory"=w95:path)
            n29 = call <vilib>:"Application Directory.vi"() -> ("Application Directory"=w110:path)
            n30 = Index Array(array=w105, index=w104) -> (element=w103:string)
            n31 = Build Path(base path=w95, name or relative path=w94) -> (appended path=w98:path)
            n32 = Build Path(base path=w110, name or relative path=w103) -> (appended path=w109:path)
            n33 = call-poly <vilib>:"Read Delimited Spreadsheet.vi"("file path (dialog if empty)"=w98, "delimiter (\\t)"="::" ("delimiter (\\t)")) -> ("all rows"=→"assoc input sensori":string[][])  [unwired: 8 in, 5 out]
            n34 = call-poly <vilib>:"Read Delimited Spreadsheet.vi"("file path (dialog if empty)"=w109, "number of rows (all:-1)"=-1, "delimiter (\\t)"="::" ("delimiter (\\t)")) -> ("all rows"=w102:string[][])  [unwired: 7 in, 5 out]
            n35 = local write "Caratteristiche sensori in"(w102) -> ()
            n36 = local write "Acq res resistomat"(FALSE ("Acq res resistomat")) -> ()
            n37 = control-ref of="This VI"() -> (w114:refnum<vi>)
            n38 = Wait (ms)(milliseconds to wait=u32 500) -> ()  [unwired: 1 out]
          }
        }
      }
      frame "AGGIORNA INFO" {
        n39 = Variant To Data(type=w158, Variant=w159) -> (data=w119:T31)  [unwired: 1 in, 1 out]
        "Cluster INFO" <- w119
        n40 = Decrement(x=w115) -> (x-1=w141:i32)
        n41 = call <vilib>:"Application Directory.vi"() -> ("Application Directory"=w126:path)
        n42 = call <vilib>:"Application Directory.vi"() -> ("Application Directory"=w129:path)
        n43 = Build Array("Settings\\Gestione sensori\\measures_settings_INPUT_B1.txt" ("name or relative path"), "Settings\\Gestione sensori\\measures_settings_INPUT_B2.txt" ("name or relative path"), "Settings\\Gestione sensori\\measures_settings_INPUT_B3.txt" ("name or relative path")) -> (w142:string[])
        n44 = Build Path(base path=w126, name or relative path="Settings\\Gestione sensori\\Attriti torsiometro B2.txt") -> (appended path=w122:path)
        n45 = Index Array(array=w142, index=w141) -> (element=w140:string)
        n46 = Build Path(base path=w129, name or relative path="Settings\\Gestione sensori\\Attriti torsiometro B1.txt") -> (appended path=w124:path)
        n47 = call <vilib>:"Application Directory.vi"() -> ("Application Directory"=w150:path)
        n48 = Decrement(x=w115) -> (x-1=w133:i32)
        n49 = Build Array("Settings\\Gestione sensori\\Assoc_Input_Sensori_B1.txt" ("name or relative path"), "Settings\\Gestione sensori\\Assoc_Input_Sensori_B2.txt" ("name or relative path"), "Settings\\Gestione sensori\\Assoc_Input_Sensori_B3.txt" ("name or relative path")) -> (w134:string[])
        n50 = call-poly <vilib>:"Read Delimited Spreadsheet.vi"("file path (dialog if empty)"=w122, "delimiter (\\t)"="::" ("delimiter (\\t)")) -> ("all rows"=w120:string[][])  [unwired: 8 in, 5 out]
        n51 = Build Path(base path=w150, name or relative path=w140) -> (appended path=w149:path)
        n52 = call-poly <vilib>:"Read Delimited Spreadsheet.vi"("file path (dialog if empty)"=w124, "delimiter (\\t)"="::" ("delimiter (\\t)")) -> ("all rows"=w121:string[][])  [unwired: 8 in, 5 out]
        n53 = Index Array(array=w134, index=w133) -> (element=w131:string)
        n54 = call <vilib>:"Application Directory.vi"() -> ("Application Directory"=w132:path)
        n55 = call-poly <vilib>:"Read Delimited Spreadsheet.vi"("file path (dialog if empty)"=w149, "number of rows (all:-1)"=-1, "delimiter (\\t)"="::" ("delimiter (\\t)")) -> ("all rows"=→"Caratteristiche sensori in":string[][])  [unwired: 7 in, 5 out]
        n56 = Build Path(base path=w132, name or relative path=w131) -> (appended path=w135:path)
        n57 = for {
          tunnel: w121 -> [w168] mode=indexing
          tunnel: [w167] -> w117 mode=indexing
          n58 = for {
            tunnel: w168 -> [w170] mode=indexing
            tunnel: [w169] -> w167 mode=indexing
            n59 = call "String To Dbl.vi"("String"=w170) -> ("Numeric"=w169:dbl)  [unwired: 10 in]
          }
        }
        n60 = for {
          tunnel: w120 -> [w164] mode=indexing
          tunnel: [w163] -> w116 mode=indexing
          n61 = for {
            tunnel: w164 -> [w166] mode=indexing
            tunnel: [w165] -> w163 mode=indexing
            n62 = call "String To Dbl.vi"("String"=w166) -> ("Numeric"=w165:dbl)  [unwired: 10 in]
          }
        }
        n63 = call-poly <vilib>:"Read Delimited Spreadsheet.vi"("file path (dialog if empty)"=w135, "delimiter (\\t)"="::" ("delimiter (\\t)")) -> ("all rows"=w139:string[][])  [unwired: 8 in, 5 out]
        n64 = local write "assoc input sensori"(w139) -> ()
        n65 = Bundle By Name(cluster=w119, "Attriti B1"=w117, "Attriti B2"=w116) -> (w118:T31)
        n66 = call <userlib>:"media misure completa.vi"("Nomi Misure"=string[] ["Q1", "Q2", "Q3", "Q4", "N", "Tq", "RM1", "RM2", "P1", "P2", "P3", "P4", "T1", "T2", "Liv.", "Pbar"], "Error in"=w157, "Funzione"=T36."INITIALIZE") -> ("Error out"=w156:errorcluster)  [unwired: 8 in, 4 out]
      }
      frame "READ NI" {
        n67 = Variant To Data(type=T1 {"AI (0-10V)"={"AI 0"=0.0, "AI 1"=0.0, "AI 2"=0.0, "AI 3"=0.0, "AI 4"=0.0, "AI 5"=0.0, "AI 6"=0.0, "AI 7"=0.0, "AI 8"=0.0, "AI 9"=0.0, "AI 10"=0.0, "AI 11"=0.0, "AI 12"=0.0, "AI 13"=0.0, "AI 14"=0.0, "AI 15"=0.0, "AI 16"=0.0, "AI 17"=0.0, "AI 18"=0.0, "AI 19"=0.0, "AI 20"=0.0, "AI 21"=0.0, "AI 22"=0.0, "AI 23"=0.0, "AI 24"=0.0, "AI 25"=0.0, "AI 26"=0.0, "AI 27"=0.0, "AI 28"=0.0, "AI 29"=0.0, "AI 30"=0.0, "AI 31"=0.0}, "StatoAO_Cdaq[0-10V]"={"AO 1"=0.0, "AO 2"=0.0, "AO 3"=0.0, "AO 4"=0.0}, "Contatori [rpm]"={"RPM 1"=0.0, "RPM 2"=0.0}, "StatoAO_Cdaq [4-20mA]"={"Cdaq_AO [0-10V] 0 for Torque"=0.0, "Cdaq_AO [0-10V] 1"=0.0, "Cdaq_AO [0-10V] 2"=0.0, "Cdaq_AO [0-10V] 3"=0.0}, "StatoDO_Cdaq"={"Scorta 0"=FALSE, "Scorta 1"=FALSE, "Scorta 2"=FALSE, "Scorta 3"=FALSE, "Scorta 4"=FALSE, "Scorta 5"=FALSE, "Scorta 6"=FALSE, "Scorta 7"=FALSE, "Scorta 8"=FALSE, "Scorta 9"=FALSE, "Scorta 10"=FALSE, "Scorta 11"=FALSE, "Scorta 12"=FALSE, "Scorta 13"=FALSE, "Scorta 14"=FALSE, "Scorta 15"=FALSE, "Scorta 16"=FALSE, "Scorta 17"=FALSE, "Scorta 18"=FALSE, "Scorta 19"=FALSE, "Scorta 20"=FALSE, "Scorta 21"=FALSE, "Scorta 22"=FALSE, "Scorta 23"=FALSE, "Scorta 24"=FALSE, "Scorta 25"=FALSE, "Scorta 26"=FALSE, "Scorta 27"=FALSE, "Scorta 28"=FALSE, "Scorta 29"=FALSE, "Scorta 30"=FALSE, "Scorta 31"=FALSE}, "DI"={"Scorta 0"=FALSE, "Scorta 1"=FALSE, "Scorta 2"=FALSE, "Scorta 3"=FALSE, "Scorta 4"=FALSE, "Scorta 5"=FALSE, "Scorta 6"=FALSE, "Scorta 7"=FALSE, "Scorta 8"=FALSE, "Scorta 9"=FALSE, "Scorta 10"=FALSE, "Scorta 11"=FALSE, "Scorta 12"=FALSE, "Scorta 13"=FALSE, "Scorta 14"=FALSE, "Scorta 15"=FALSE, "Scorta 16"=FALSE, "Scorta 17"=FALSE, "Scorta 18"=FALSE, "Scorta 19"=FALSE, "Scorta 20"=FALSE, "Scorta 21"=FALSE, "Scorta 22"=FALSE, "Scorta 23"=FALSE, "Scorta 24"=FALSE, "Scorta 25"=FALSE, "Scorta 26"=FALSE, "Scorta 27"=FALSE, "Scorta 28"=FALSE, "Scorta 29"=FALSE, "Scorta 30"=FALSE, "Scorta 31"=FALSE}, "AI (4-20mA)"={"AI 0"=0.0, "AI 1"=0.0, "AI 2"=0.0, "AI 3"=0.0, "AI 4"=0.0, "AI 5"=0.0, "AI 6"=0.0, "AI 7"=0.0, "AI 8"=0.0, "AI 9"=0.0, "AI 10"=0.0, "AI 11"=0.0, "AI 12"=0.0, "AI 13"=0.0, "AI 14"=0.0, "AI 15"=0.0}, "TC [°C]"={"tc 1"=0.0, "tc 2"=0.0, "tc 3"=0.0, "tc 4"=0.0}, "NI Read Values"={"RPM"=0.0, "Frequency"=0.0, "Mod 1"={"Torsiometro 1"=0.0, "Torsiometro 2"=0.0, "Strin Gauge 1"=0.0, "Strin Gauge 2"=0.0}, "Mod 2"={"Termocoppia 1"=0.0, "Termocoppia 2"=0.0, "Termocoppia 3"=0.0, "Termocoppia 4"=0.0}, "Mod 3"={"PT 100 1"=0.0, "PT 100 2"=0.0, "PT 100 3"=0.0, "PT 100 4"=0.0}}} ("Cluster READ"), Variant=w181) -> (data=w172:T1)  [unwired: 1 in, 1 out]
        "Cluster READ NI" <- w172
        n68 = Unbundle By Name(w172) -> ("NI Read Values"=w171:T43)
        n69 = Bundle By Name(cluster=w178, "Cluster READ NI.NI Read Values"=w171) -> (w177:T9)
        n70 = local write "Task READ WT ok"(TRUE) -> ()
      }
      frame "Leggi PLC 1" {
        # "OFFSET PER COMPENSAZIONE VALORE RPM\n\nCI SONO DISTURBI CHE INTRODUCONO UN OFFSET NELL AI DEI RPM,\nTALE OFFSET è DIVERSO SE SI UTILIZZA IL FILTRO O MENO."
        n71 = Variant To Data(type=T15 {"USCITE PLC"={"AO (real) 2"={"SCORTA 1"=0.0, "SCORTA 2"=0.0, "SCORTA 3"=0.0, "SCORTA 4"=0.0, "SCORTA 5"=0.0, "SCORTA 6"=0.0, "SCORTA 7"=0.0, "SCORTA 8"=0.0}, "statoAO_PLC out"={"Rif Lim coppia freno [%]"=0.0, "Rif rpm freno [%]"=0.0, "Rif coppia freno [%]"=0.0, "Rif V alimentatore [%]"=0.0, "Rif F alimentatore [%]"=0.0}, "DO (bit)"={"Scelta banco 1"=FALSE, "Set dati motore freno 2"=FALSE, "Diretto inverter"=FALSE, "Filtro LC"=FALSE, "Marcia ALIM (1s)"=FALSE, "Marcia FRENO (1s)"=FALSE, "Stop AFE (1s)"=FALSE, "Stop freno (1s)"=FALSE, "Reset allarmi"=FALSE, "Watchdog"=FALSE, "Senso rotazione"=FALSE, "Abilita collaudo (1s)"=FALSE, "Disabilita collaudo (1s)"=FALSE, "Abilitazione ALIM"=FALSE, "Abilitazione FRENO"=FALSE, "Teleruttore WT"=FALSE, "Senso rot motore prova"=FALSE, "Scorta 7"=FALSE, "Scorta 8"=FALSE, "Scorta 9"=FALSE, "Scorta 10"=FALSE, "Scorta 11"=FALSE, "Scorta 12"=FALSE, "Scorta 13"=FALSE}}, "Stato DI_PLC"={"Sistema OK"=FALSE, "Rotore bloccato"=TRUE, "Scorta 1"=FALSE, "Prova diretto inverter"=FALSE, "Prova con filtro LC"=FALSE, "Teleruttore WT abilitato"=FALSE, "Alim sinus penta abilitato"=FALSE, "Alim sinus penta in marcia"=FALSE, "Freno abilitato"=FALSE, "Freno in marcia"=FALSE, "Senso rotazione freno"=FALSE, "Potenza abilitata"=FALSE, "Scorta 3"=FALSE, "Scorta 4"=FALSE, "scorta 5"=FALSE, "scorta 6"=FALSE}, "AI plc"={"Allarmi 1"=0.0, "Allarmi 2"=0.0, "Scorta 1"=0.0, "Scorta 2"=0.0, "RPM mot prova"=0.0, "I mot prova"=0.0, "RPM freno"=0.0, "I freno"=0.0, "Scorta 3"=0.0, "Scorta 4"=0.0}} ("STATO PLC"), Variant=w196) -> (data=w191:T15)  [unwired: 1 in, 1 out]
        n72 = Unbundle By Name(w191) -> ("AI plc.RPM freno"=w192:dbl, "USCITE PLC.DO (bit).Filtro LC"=w188:bool)
        n73 = Select(t=40.0, s=w188, f=250.0) -> (s? t:f=w186:dbl)
        n74 = Add(x=w192, y=w186) -> (x+y=w189:dbl)
        n75 = Bundle By Name(cluster=w191, "AI plc.RPM freno"=w189) -> (w190:T15)
        n76 = Bundle By Name(cluster=w194, "STATO PLC 1"=w190) -> (w193:T9)
      }
      frame "Leggi PLC 2" {
        n77 = Unbundle By Name(w205) -> ("STATO PLC 2"=w204:T20)
        n78 = Variant To Data(type=w204, Variant=w208) -> (data=w207:T20)  [unwired: 1 in, 1 out]
        n79 = Bundle By Name(cluster=w205, "STATO PLC 2"=w207) -> (w206:T9)
      }
      frame "Leggi PLC 3" {
        n80 = Unbundle By Name(w217) -> ("STATO PLC 3"=w216:T24)
        n81 = Variant To Data(type=w216, Variant=w220) -> (data=w219:T24)  [unwired: 1 in, 1 out]
        n82 = Bundle By Name(cluster=w217, "STATO PLC 3"=w219) -> (w218:T9)
      }
      frame "READ WT" {
        # "misure potenza in kw"
        n83 = Variant To Data(type=T6 {"URMS 1"=0.0, "IRMS 1"=0.0, "P 1"=0.0, "S 1"=0.0, "Q 1"=0.0, "LAMBDA 1"=0.0, "PHI 1"=0.0, "F U 1"=0.0, "F I 1"=0.0, "NONE 1"=0.0, "URMS 2"=0.0, "IRMS 2"=0.0, "P 2"=0.0, "S 2"=0.0, "Q 2"=0.0, "LAMBDA 2"=0.0, "PHI 2"=0.0, "F U 2"=0.0, "F I 2"=0.0, "NONE 2"=0.0, "URMS 3"=0.0, "IRMS 3"=0.0, "P 3"=0.0, "S 3"=0.0, "Q 3"=0.0, "LAMBDA 3"=0.0, "PHI 3"=0.0, "F U 3"=0.0, "F I 3"=0.0, "NONE 3"=0.0, "URMS SIGMA"=0.0, "IRMS SIGMA"=0.0, "P SIGMA"=0.0, "S SIGMA"=0.0, "Q SIGMA"=0.0, "LAMBDA SIGMA"=0.0, "PHI SIGMA"=0.0, "F U SIGMA"=0.0, "F I SIGMA"=0.0, "NONE 4"=0.0} ("MISURE WT"), Variant=w242) -> (data=w234:T6)  [unwired: 1 in, 1 out]
        "MISURE WT" <- w234
        n84 = local write "Task READ WT ok"(TRUE ("Task READ NI ok")) -> ()
        n85 = Unbundle By Name(w234) -> ("P 1"=w231:dbl, "P 2"=w230:dbl, "P 3"=w229:dbl, "P SIGMA"=w228:dbl)
        n86 = Bundle By Name(cluster=w234, "P 1"=w231, "P 2"=w230, "P 3"=w229, "P SIGMA"=w228) -> (w233:T6)
        n87 = Bundle By Name(cluster=w235, "MISURE WT"=w233) -> (w240:T9)
      }
      frame "READ SINUS PENTA" {
        n88 = Unbundle By Name(w247) -> ("READ SINUS PENTA"=w249:T19)
        n89 = Variant To Data(type=w249, Variant=w250) -> (data=w248:T19)  [unwired: 1 in, 1 out]
        n90 = Bundle By Name(cluster=w247, "READ SINUS PENTA"=w248) -> (w246:T9)
      }
      frame "READ DCREG" {
        n91 = Unbundle By Name(w259) -> ("DCREG"=w261:T28)
        n92 = Variant To Data(type=w261, Variant=w262) -> (data=w260:T28)  [unwired: 1 in, 1 out]
        n93 = Bundle By Name(cluster=w259, "DCREG"=w260) -> (w258:T9)
      }
      frame "READ RPM" {
        n94 = Variant To Data(type=0.0, Variant=w272) -> (data=w270:dbl)  [unwired: 1 in, 1 out]
        n95 = Bundle By Name(cluster=w274, "Cluster READ NI.Contatori [rpm].RPM 1"=w270, "Cluster READ NI.Contatori [rpm].RPM 2"=w270) -> (w273:T9)
      }
      frame "READ RESISTENZE RESISTOMAT" {
        n96 = Variant To Data(type=T5 {"Res Ch1"=0.0, "Res Ch2"=0.0, "Res Ch3"=0.0, "Tamb"=0.0} ("Cluster Resistenze"), Variant=w297) -> (data=w289:T5)  [unwired: 1 in, 1 out]
        n97 = Unbundle By Name(w289) -> ("Res Ch1"=w286:dbl, "Res Ch2"=w285:dbl, "Res Ch3"=w284:dbl, "Tamb"=w282:dbl)
        n98 = Bundle By Name(cluster=T5 {"Res Ch1"=0.0, "Res Ch2"=0.0, "Res Ch3"=0.0, "Tamb"=0.0} ("data"), "Res Ch1"=w286, "Res Ch2"=w285, "Res Ch3"=w284, "Tamb"=w282) -> (w288:T5)
        n99 = Bundle By Name(cluster=w296, "Resistenze Resistomat"=w288) -> (w295:T9)
        "Acq res resistomat" <- TRUE
      }
      frame "READ RESISTENZE RES METER" {
        n100 = Variant To Data(type=cluster{"[0]":dbl, "[1]":dbl} {"[0]"=0.0, "[1]"=0.0} ("cluster"), Variant=w313) -> (data=w306:cluster{"[0]":dbl, "[1]":dbl})  [unwired: 1 in, 1 out]
        n101 = Unbundle By Name(w306) -> ("[0]"=w302:dbl, "[1]"=w301:dbl)
        n102 = Bundle By Name(cluster=T5 {"Res Ch1"=0.0, "Res Ch2"=0.0, "Res Ch3"=0.0, "Tamb"=0.0} ("data"), "Res Ch1"=w302, "Res Ch2"=w301) -> (w305:T5)
        n103 = Bundle By Name(cluster=w312, "Resistenze Res Meter"=w305) -> (w311:T9)
      }
      frame "READ RES FREDDO RESISTOMAT" {
        # "AGGIORNO ANCHE CLUSTER RESISTENZE\nCOSì NEL CASO STIA USANDO IL RESISTOMAT\nLE PRIME ACQUISIZIONI HANNO DT=0°C"
        n104 = Variant To Data(type=T5 {"Res Ch1"=0.0, "Res Ch2"=0.0, "Res Ch3"=0.0, "Tamb"=0.0} ("Cluster Resistenze"), Variant=w328) -> (data=w318:T5)  [unwired: 1 in, 1 out]
        n105 = Unbundle By Name(w318) -> ("Res Ch1"=w323:dbl, "Res Ch2"=w326:dbl, "Res Ch3"=w325:dbl, "Tamb"=w324:dbl)
        n106 = Bundle By Name(cluster=w329, "FREDDO resistomat.Res Ch1"=w323, "FREDDO resistomat.Res Ch2"=w326, "FREDDO resistomat.Res Ch3"=w325, "FREDDO resistomat.tAMB"=w324) -> (w332:T9)
        n107 = global write "Global prova in corso.vi" "prova in corso?"(FALSE ("prova in corso?")) -> ()
        n108 = Bundle By Name(cluster=T37 {"Array of elements"=[], "Single element"={"String"="READ RESISTENZE RESISTOMAT", "variant"=variant}, "enque at\nopposite end (F)"=FALSE, "no replications (F)"=FALSE} ("Enqueue cluster"), "Single element.variant"=w318) -> (w322:T37)
        n109 = call <userlib>:"SMQ_MANAGER.vi"("Function"=enum16{"INITIALIZE", "ENQUEUE", "STOP ALL"}."ENQUEUE", "Queue name"="DATA_Q", "Enqueue cluster"=w322) -> ()  [unwired: 8 in, 1 out]
      }
      frame "READ RES FREDDO RES METER" {
        # "AGGIORNO ANCHE CLUSTER RESISTENZE\nCOSì NEL CASO STIA USANDO IL RESISTOMAT\nLE PRIME ACQUISIZIONI HANNO DT=0°C"
        n110 = Variant To Data(type=T38 {"Res Ch1"=0.0, "Res Ch2"=0.0, "tAMB"=0.0, "Res Ch3"=0.0} ("FREDDO resistomat"), Variant=w354) -> (data=w347:T38)  [unwired: 1 in, 1 out]
        n111 = Unbundle By Name(w344) -> ()  [unwired: 1 out]
        n112 = case shown="2" i16 2 ("#rami freddo\\eq term") {
          tunnel: w347 -> [_ w371 w375 w382]
          tunnel: [w363 w368 w373 w379] -> w346
          tunnel: [w363 w367 w372 w378] -> w345
          tunnel: [w363 "0" ("R3_freddo[ohm]") w372 w376] -> w343
          tunnel: [_ w364 _ _] -> w341
          frame 0, Default {
            w363 = "0"
          }
          frame 2 {
            n113 = Unbundle By Name(w371) -> ("tAMB"=w365:dbl, "Res Ch1"=w370:dbl, "Res Ch2"=w369:dbl)
            n114 = Number To Fractional String(number=w370) -> (F-format string=w368:string)  [unwired: 3 in]
            n115 = Number To Fractional String(number=w365) -> (F-format string=w364:string)  [unwired: 3 in]
            n116 = Number To Fractional String(number=w369) -> (F-format string=w367:string)  [unwired: 3 in]
          }
          frame 1 {
            w372 = "0" ("R3_freddo[ohm]")
            n117 = Unbundle By Name(w375) -> ("Res Ch1"=w374:dbl)  [unwired: 1 out]
            n118 = Number To Fractional String(number=w374) -> (F-format string=w373:string)  [unwired: 3 in]
          }
          frame 3 {
            n119 = Unbundle By Name(w382) -> ("Res Ch1"=w381:dbl, "Res Ch2"=w380:dbl, "Res Ch3"=w377:dbl)
            n120 = Number To Fractional String(number=w381) -> (F-format string=w379:string)  [unwired: 3 in]
            n121 = Number To Fractional String(number=w377) -> (F-format string=w376:string)  [unwired: 3 in]
            n122 = Number To Fractional String(number=w380) -> (F-format string=w378:string)  [unwired: 3 in]
          }
        }
        n123 = local read "Cluster MISURE"() -> (w340:T7)
        n124 = Unbundle By Name(w340) -> ("MISURE NM"=w339:T8)
        n125 = Bundle By Name(cluster=w339, "TambFreddo[°C]"=w341, "R1_freddo[ohm]"=w346, "R2_freddo[ohm]"=w345, "R3_freddo[ohm]"=w343, "R_Marcia_freddo[ohm]"=w346, "R_Aux_freddo[ohm]"=w345, "R_Arm_freddo[ohm]"=w346, "R_Ecc_freddo[ohm]"=w345) -> (w352:T8)
        n126 = Bundle By Name(cluster=w356, "FREDDO res meter"=w347) -> (w355:T9)
        n127 = global write "Global prova in corso.vi" "prova in corso?"(FALSE ("prova in corso?")) -> ()
        n128 = Bundle By Name(cluster=T37 {"Array of elements"=[], "Single element"={"String"="ACQ FREDDO RES METER", "variant"=variant}, "enque at\nopposite end (F)"=FALSE, "no replications (F)"=FALSE} ("Enqueue cluster"), "Single element.variant"=w352) -> (w351:T37)
        n129 = call <userlib>:"SMQ_MANAGER.vi"("Function"=enum16{"INITIALIZE", "ENQUEUE", "STOP ALL"}."ENQUEUE", "Queue name"="MAIN2_Q", "Enqueue cluster"=w351) -> ()  [unwired: 8 in, 1 out]
      }
      frame "CARICA RES FREDDO RES METER" {
        # "AGGIORNO ANCHE CLUSTER RESISTENZE\nCOSì NEL CASO STIA USANDO IL RESISTOMAT\nLE PRIME ACQUISIZIONI HANNO DT=0°C"
        n130 = Variant To Data(type=T38 {"Res Ch1"=0.0, "Res Ch2"=0.0, "tAMB"=0.0, "Res Ch3"=0.0} ("FREDDO resistomat"), Variant=w387) -> (data=w385:T38)  [unwired: 1 in, 1 out]
        n131 = Bundle By Name(cluster=w389, "FREDDO res meter"=w385) -> (w388:T9)
        n132 = global write "Global prova in corso.vi" "prova in corso?"(FALSE ("prova in corso?")) -> ()
      }
      frame "CARICA RES FREDDO RESISTOMAT" {
        # "BENAZZATO. SE CONTINUO COLLAUDO VADO A CARICARE LA R A FREDDO E AGGIORNO SIA CLUSTER R_FREDDO\nSIA R_RESISTOMAT PER FARE IN MODO CHE DT SIA NULLO QUANDO PARTE LA PROVA TERMICA.\nQUESTO CASE SERVE ANCHE SE L'UTENTE SVUOTA LA TABELLA DELLE R A FREDDO: IMPONGO A ZERO TUTTO"
        n133 = Variant To Data(type=T5 {"Res Ch1"=0.0, "Res Ch2"=0.0, "Res Ch3"=0.0, "Tamb"=0.0} ("Cluster Resistenze"), Variant=w402) -> (data=w403:T5)  [unwired: 1 in, 1 out]
        n134 = Unbundle By Name(w403) -> ("Res Ch1"=w399:dbl, "Res Ch2"=w398:dbl, "Res Ch3"=w397:dbl, "Tamb"=w396:dbl)
        n135 = Bundle By Name(cluster=w401, "FREDDO resistomat.Res Ch1"=w399, "FREDDO resistomat.Res Ch2"=w398, "FREDDO resistomat.Res Ch3"=w397, "FREDDO resistomat.tAMB"=w396, "Resistenze Resistomat.Res Ch1"=w399, "Resistenze Resistomat.Res Ch2"=w398, "Resistenze Resistomat.Res Ch3"=w397, "Resistenze Resistomat.Tamb"=w396) -> (w400:T9)
      }
      frame "CARICA RES RESISTOMAT" {
        # "BENAZZATO. QUANDO L'UTENTE SVUOTA TABELLA DELLA RESISTENZA TERMICA INIZIALIZZO IL CLUSTER DELLE R_RESISTOMAT\nUGUALE ALLA TABELLA DELLE R A FREDDO. SE LA TABELLA DELLA R A FREDDO E' VUOTA IMPONGO ZERO"
        n136 = local read "Cluster MISURE"() -> (w412:T7)
        n137 = Variant To Data(type=T5 {"Res Ch1"=0.0, "Res Ch2"=0.0, "Res Ch3"=0.0, "Tamb"=0.0} ("Cluster Resistenze"), Variant=w419) -> (data=w420:T5)  [unwired: 1 in, 1 out]
        n138 = Unbundle By Name(w412) -> ("MISURE NM.Tamb[°C]"=w417:string)
        n139 = Unbundle By Name(w420) -> ("Res Ch1"=w421:dbl, "Res Ch2"=w423:dbl, "Res Ch3"=w422:dbl)
        n140 = call "String To Dbl.vi"("String"=w417) -> ("Numeric"=w416:dbl)  [unwired: 10 in]
        n141 = Bundle By Name(cluster=w415, "Resistenze Resistomat.Res Ch1"=w421, "Resistenze Resistomat.Res Ch2"=w423, "Resistenze Resistomat.Res Ch3"=w422, "Resistenze Resistomat.Tamb"=w416) -> (w418:T9)
      }
      frame "AGGIORNA DATI TECNICI" {
        n142 = Variant To Data(type=T30 {"Numero"=0.0, "Tipo Pompa"=0.0, "Costruttore"=0.0, "n°serie"=0.0, "Tipo Motore"=0.0, "Costruttore"=0.0, "n°serie"=0.0, "Tipologia"=0.0, "Tipo Inverter"=0.0, "Costruttore"=0.0, "n°serie"=0.0, "Tipologia"=0.0, "Data"=0.0, "Nome Cliente"=0.0, "Test Engineer"=0.0, "Q1 [m3/h]"=0.0, "H1 [m]"=0.0, "Q2 [m3/h]"=0.0, "H2 [m]"=0.0, "Qmax [m3/h]"=0.0, "Hmax [m]"=0.0, "n° giranti"=0.0, "MEI"=0.0, "EEI"=0.0, "IE"=0.0, "fn [Hz]"=0.0, "Un [V]"=0.0, "In [A]"=0.0, "P1 [W]"=0.0, "P2 [W]"=0.0, "Crun [uF]"=0.0, "Cstart [uF]"=0.0, "Uc [V]"=0.0, "Numero Poli"=0.0, "n [rpm]"=0.0, "Tn [Nm]"=0.0, "pfn"=0.0, "etp [p.u.]"=0.0, "etg [p.u.]"=0.0, "C.I."=0.0, "Collegamento"=0.0, "Peso [kg]"=0.0, "Servizio"=0.0, "IP"=0.0, "Ru-w [Ohm]"=0.0, "Temp0 [°C]"=0.0, "DTavv. [°C]"=0.0, "DTcassa [°C]"=0.0, "IIr [A]"=0.0, "TIr [Nm]"=0.0, "Note1"=0.0, "Note2"=0.0, "Note3"=0.0, "Note4"=0.0, "Dislivello [m]"=0.0, "Tubo d1n [DN]"=0.0, "Tubo d1 [mm]"=0.0, "Tubo1 lungh [mm]"=0.0, "Tubo1 rug1"=0.0, "Tubo d2n [DN]"=0.0, "Tubo d2 [mm]"=0.0, "Tubo2 lungh [mm]"=0.0, "Tubo2 rug1"=0.0, "Cono1 d1 [mm]"=0.0, "Cono1 d2 [mm]"=0.0, "Cono1 l [mm]"=0.0, "Cono2 d1 [mm]"=0.0, "Cono2 d2 [mm]"=0.0, "Cono2 l [mm]"=0.0, "Note5"=0.0, "Note6"=0.0, "n° giranti"=0.0, "D1 girante [mm]"=0.0, "B2 girante [mm]"=0.0, "materiale"=0.0, "tenuta"=0.0, "oring"=0.0, "mod.girante"=0.0, "mod.corpo p"=0.0, "Note7"=0.0, "Note8"=0.0, "Pacco"=0.0, "d int. [mm]"=0.0, "d est. [mm]"=0.0, "d est.rotore[mm]"=0.0, "Traferro [mm]"=0.0, "Costruzione"=0.0, "Note9"=0.0, "Note10"=0.0, "f mod. [kHz]"=0.0, "Mod. Pot. [A]"=0.0, "Taglia [W]"=0.0, "Tipologia"=0.0} ("DATI NM 2"), Variant=w437) -> (data=w435:T30)  [unwired: 1 in, 1 out]
        n143 = case shown="True" w436 {
          tunnel: w435 -> [_ w442]
          frame False {
            # "UL"
          }
          frame True {
            # "NM"
            "DATI NM" <- w442
          }
        }
      }
      frame "AGGIORNA T&R" {
        n144 = Variant To Data(type=T39 {"Tamb[°C]"=0.0, "Ru-w"=0.0, "Rmarcia"=0.0, "Raux"=0.0, "Tamb Freddo[°C]"=0.0, "Ru-w freddo"=0.0, "Rmarcia freddo"=0.0, "Raux freddop"=0.0, "TC1"=0.0, "TC2"=0.0, "TC3"=0.0, "TC4"=0.0, "TC5"=0.0, "TC6"=0.0, "TC7"=0.0, "TC8"=0.0} ("Sett T e R 5"), Variant=w445) -> ()  [unwired: 1 in, 2 out]
      }
      frame "REF NPSH" {
        n145 = Variant To Data(type=T40 {"Cluster NPSH"=refnum, "Cluster ctrl NPSH"=refnum} ("output cluster"), Variant=w457) -> (data=w456:T40)  [unwired: 1 in, 1 out]
      }
      frame "SET Q REF" {
        n146 = Variant To Data(type=T41 {"Value"=TRUE, "Qref"=0.0, "Htot ref"=0.0, "MODALITA' SCELTA Qref Htot ref"=enum."Imposta manualmente"}, Variant=w466) -> (data=w463:T41)  [unwired: 1 in, 1 out]
        n147 = Unbundle By Name(w463) -> ("Value"=w465:bool)
        n148 = case shown="False" w465 {
          tunnel: w471 -> [w497 w512]
          tunnel: [FALSE TRUE] -> w469
          tunnel: w468 -> [w485 w509]
          tunnel: [_ w509] -> w467
          tunnel: w463 -> [w476 _]
          frame False {
            w478 = u32 16777216
            n149 = Unbundle By Name(w476) -> ("MODALITA' SCELTA Qref Htot ref"=w477:T44)
            n150 = Unbundle By Name(w497) -> ("Cluster NPSH"=w496:refnum<vi>, "Cluster ctrl NPSH"=w490:refnum<vi>)
            n151 = case shown="\"Parti da QH Regime\"" w477 {
              tunnel: w485 -> [w502 _ _]
              tunnel: [w499 w504 w507] -> w484
              tunnel: [w498 w503 w506] -> w483
              tunnel: w476 -> [_ w505 w508]
              frame "Imposta manualmente", Default {
                n152 = Unbundle(w502) -> (w501:dbl[], w500:dbl[])
                n153 = call-poly <vilib>:"Mean.vi"("X"=w501) -> ("mean"=w499:dbl)  [unwired: 1 out]
                n154 = call-poly <vilib>:"Mean.vi"("X"=w500) -> ("mean"=w498:dbl)  [unwired: 1 out]
              }
              frame "Parti da QH Freddo" {
                n155 = Unbundle By Name(w505) -> ("Qref"=w504:dbl, "Htot ref"=w503:dbl)
              }
              frame "Parti da QH Regime" {
                n156 = Unbundle By Name(w508) -> ("Qref"=w507:dbl, "Htot ref"=w506:dbl)
              }
            }
            n157 = property class="Clust (strict)"(reference=w496) -> (reference out=w494:refnum<vi>, "Value"=w495:T45)  [unwired: 1 in, 1 out]
            n158 = property class="Clust (strict)"(reference=w490, "DisabledEnum"=T42."Enabled" ("Disabled")) -> ()  [unwired: 1 in, 2 out]
            n159 = property class="Clust (strict)"(reference=w490) -> ("Controls[]"=w489:refnum<vi>[])  [unwired: 1 in, 2 out]
            n160 = Index Array(array=w489, index #1=0 ("index"), index #2=1 ("index"), index #3=3 ("index")) -> (element #1=w487:refnum<vi>, element #2=w480:refnum<vi>, element #3=w479:refnum<vi>)
            n161 = Bundle By Name(cluster=w495, "Q ref"=w484, "Htot ref"=w483) -> (w493:T45)
            n162 = property class="Clust (strict)"(reference=w494, "Value"=w493) -> ()  [unwired: 1 in, 2 out]
            n163 = property class="Ctl"(reference=w487, "Value"=FALSE) -> ()  [unwired: 1 in, 2 out]
            n164 = property class="Ctl"(reference=w480, "Caption.BGColor"=w478) -> ()  [unwired: 1 in, 2 out]
            n165 = property class="Ctl"(reference=w479, "Caption.BGColor"=w478) -> ()  [unwired: 1 in, 2 out]
          }
          frame True {
            n166 = Unbundle By Name(w512) -> ("Cluster ctrl NPSH"=w511:refnum<vi>)
            n167 = property class="Clust (strict)"(reference=w511, "DisabledEnum"=T42."Disabled" ("Disabled")) -> ()  [unwired: 1 in, 2 out]
          }
        }
      }
      frame "SEND?" {
        n168 = Variant To Data(type=TRUE, Variant=w521) -> (data=w519:bool)  [unwired: 1 in, 1 out]
        "SEND_Main?" <- w519
      }
      frame "SEND MAIN2?" {
        n169 = Variant To Data(type=TRUE, Variant=w532) -> (data=→"SEND_Main2?":bool)  [unwired: 1 in, 1 out]
      }
      frame "SEND DATA" {
        # "scala tutti gli ingressi e mappa\nl'interfaccia delle misure"
        n170 = local read "Caratteristiche sensori in"() -> (w544:string[][])
        n171 = local read "assoc input sensori"() -> (w543:string[][])
        n172 = local read "Acq res resistomat"() -> (w537:bool)
        n173 = call "Mappa interfaccia.vi"("Assoc_input_sensori"=w543, "Cluster INFO"=w535, "banco"=w542, "Caratteristiche Caricate"=w544, "MISURE ALL"=w546) -> ("MISURE ALL out"=w545:T9)  [unwired: 6 in]
        n174 = local read "DATI NM"() -> (w554:T30)
        n175 = call "MAPPA MISURE.vi"("Torsiometro"=w538, "DATI NM"=w554, "Cluster INFO"=w535, "MISURE ALL"=w545, "ACQ RESISTOMAT?"=w537, "SIMULAZIONE"=w541) -> ("Cluster MISURE"=w540:T7)  [unwired: 13 in]
        "Cluster MISURE" <- w540
        n176 = Unbundle By Name(w540) -> ("MISURE NM"=w539:T8)
        n177 = local read "SEND_Main2?"() -> (w548:bool)
        n178 = Bundle By Name(cluster=T37 {"Array of elements"=[], "Single element"={"String"="READ DATA", "variant"=variant}, "enque at\nopposite end (F)"=FALSE, "no replications (F)"=FALSE} ("Enqueue cluster"), "Single element.variant"=w540) -> (w555:T37)
        n179 = case shown="True" w537 {
          tunnel: w539 -> [_ w561]
          frame False {
          }
          frame True {
            n180 = Bundle By Name(cluster=T37 {"Array of elements"=[], "Single element"={"String"="ACQ RESISTOMAT", "variant"=variant}, "enque at\nopposite end (F)"=FALSE, "no replications (F)"=FALSE} ("Enqueue cluster"), "Single element.variant"=w561) -> (w562:T37)
            n181 = Unbundle By Name(w561) -> ("Tamb[°C]"=w560:string)
            n182 = call "String To Dbl.vi"("String"=w560) -> ("Numeric"=→"tamb":dbl)  [unwired: 10 in]
            n183 = local write "Acq res resistomat"(FALSE ("Acq res resistomat")) -> ()
            n184 = call <userlib>:"SMQ_MANAGER.vi"("Function"=enum16{"INITIALIZE", "ENQUEUE", "STOP ALL"}."ENQUEUE", "Queue name"="MAIN2_Q", "Enqueue cluster"=w562) -> ()  [unwired: 8 in, 1 out]
          }
        }
        n185 = case shown="True" w548 {
          tunnel: [string[] ["READ_DATA_1_Q"] string[] ["READ_DATA_1_Q", "READ_DATA_2_Q"]] -> w552
          frame False {
          }
          frame True {
          }
        }
        n186 = case shown="True" TRUE {
          tunnel: w557 -> [w569 w573]
          tunnel: w555 -> [_ w572]
          tunnel: [w569 w571] -> w553
          tunnel: w552 -> [_ w570]
          frame False {
          }
          frame True {
            n187 = for {
              tunnel: w572 -> [w576]
              shift-right: [w575] -> w571
              shift-left: w573 -> [w578]
              tunnel: w570 -> [w574] mode=indexing
              n188 = call <userlib>:"SMQ_MANAGER.vi"("Function"=enum16{"INITIALIZE", "ENQUEUE", "STOP ALL"}."ENQUEUE", "Queue name"=w574, "error in (no error)"=w578, "Enqueue cluster"=w576) -> ("error out"=w575:errorcluster)  [unwired: 7 in]
            }
          }
        }
        "simulazione 2" <- w541
      }
      frame "OPEN" {
        n189 = call <userlib>:"easy open VI panel.vi"("VI in"=w585) -> ()  [unwired: 10 in, 1 out]
      }
      frame "STOP" {
      }
    }
    n190 = Or(x=w74, y=w75) -> (x .or. y?=w68:bool)
  }
  "error out" <- w28
  n191 = while {
    shift-right: [w602] -> _
    shift-left: TRUE -> [w605]
    tunnel: w14 -> [_]
    stop <- w607 stop-if-true
    # "Sincronizzo su misure wt"
    # "PROCESSI CONTINUI"
    n192 = local read "Task READ WT ok"() -> (w596:bool)
    n193 = call "Elapsed Time"("Time Target (s)"=0.25, "Reset"=w605, "Auto Reset"=FALSE) -> ("Time has Elapsed"=w603:bool)  [unwired: 9 in, 7 out]
    n194 = call "Elapsed Time2"("Time Target (s)"=2.0, "Reset"=w596, "Auto Reset"=TRUE) -> ("Time has Elapsed"=w597:bool)  [unwired: 9 in, 7 out]
    n195 = And(x=w596, y=w603) -> ()  [unwired: 1 out]
    n196 = Or(x=w597, y=w596) -> (x .or. y?=w598:bool)
    n197 = case shown="True" w598 {
      tunnel: [_ TRUE] -> w602
      frame False {
      }
      frame True {
        (unwired) "DATA_Q" ("Queue Name")
        n198 = local read "Queue Name"() -> (w609:string)
        n199 = local write "Task READ WT ok"(FALSE ("Task READ NI ok")) -> ()
        n200 = call <userlib>:"SMQ_MANAGER.vi"("Function"=enum16{"INITIALIZE", "ENQUEUE", "STOP ALL"}."ENQUEUE", "Queue name"=w609, "Enqueue cluster"=T37 {"Array of elements"=[], "Single element"={"String"="SEND DATA", "variant"=variant}, "enque at\nopposite end (F)"=TRUE, "no replications (F)"=FALSE}) -> ()  [unwired: 8 in, 1 out]
      }
    }
    n201 = local read "Stopped"() -> (w607:bool)
    n202 = Wait Until Next ms Multiple(millisecond multiple=u32 10) -> ()  [unwired: 1 out]
  }
  n203 = while {
    stop <- w613 stop-if-true
    # "PROCESSI A EVENTI"
    n204 = event shown="[0] \"Stopped\": Value Change" {
      selector: _ -> [_]
      dyn-events: _ -> [_]
      timeout: _ -> [_]
      tunnel: [w614] -> w613
      event "Stopped": Value Change {
        n205 = event-data() -> ("NewVal"=w614:bool)  [unwired: 1 in]
      }
    }
  }
  n206 = property on="Stopped" class="Bool (strict)"("Val(Sgnl)"=w25) -> (error out=w17:errorcluster)  [unwired: 2 in, 1 out]
  n207 = property class="VI"(reference=w16, error in=w17) -> (reference out=w19:refnum<vi>, error out=w15:errorcluster, "FP.State"=w18:T46)
  n208 = case shown="\"Standard\"" w18 {
    tunnel: w19 -> [_ w616]
    tunnel: w15 -> [_ w615]
    frame "Invalid", Default {
    }
    frame "Standard" {
      n209 = invoke class="VI" method="FP.Close"(reference=w616, error in=w615) -> ()  [unwired: 1 in, 3 out]
    }
  }
  "Task READ WT ok" <- w1
